vi "Q14070-Z060B.vi"() -> ()   [LabVIEW 2013]
uses:
  <vilib>/Utility/file.llb/Read From Spreadsheet File (string).vi
  <vilib>/express/express arith-compare/Formula/XNode/ExpressFormulaBlockNode.xnode
  PCI8622_32.dll
  <vilib>/printing/EasyPrintingControls.llb/contents.ctl
  <vilib>/Utility/NIReport.llb/NI_ReportGenerationCore.lvlib
  <vilib>/printing/EasyPrintingControls.llb/report_type.ctl
  <vilib>/Utility/NIReport.llb/NI_report.lvclass
  <vilib>/printing/EasyPrinting.llb/Easy Print VI Panel or Documentation (path).vi
panel:
  in  "?":bool
  in  "密码":string
  in  "?":bool
  in  "?":bool
  in  "截取百分比":dbl=0.05
  in  "半行程":dbl=70.0
  in  "是否取消放行按钮":bool
  out "PLC":bool
  out "齿条传动比":dbl=200.0 caption="L+Lmax(mm)" format="%#.3f"
  out "右平均轴向力(N)":dbl caption="L+Lmax(mm)" format="%#.3f"
  out "左平均轴向力(N)":dbl caption="最大位移偏离Lmax(mm)" format="%#.3f"
  in  "确定按钮":bool
  out "员工ID":string
  in  "出支线工步号":dbl
  out "报警提示":string
  in  "报警工步号":dbl
  out "急停":bool
  out "DeviceHandle":u32
  in  "轴向力设定次数":dbl=5.0
  in  "最小间隙(mm)":dbl=0.0005 format="%#.3f"
  out "本备料状态H":bool
  out "本测试状态H":bool
  out "本自动状态H":bool
  out "夹头松开":bool
  out "测头右位":bool
  out "测头左位":bool
  in  "测头气缸右移":bool
  in  "测头气缸左移":bool
  in  "轴向力已做次数":dbl
  out "轴向力及全行程间隙合格":bool
  out "轴向力启动":bool
  out "间隙启动":bool
  out "夹头夹紧位":bool
  in  "夹头松开":bool
  in  "夹头夹紧":bool
  out "找帽扭矩":dbl=5.0 caption="压力传感器" format="%#.2f"
  out "error out":errorcluster
  out "型号数量":i32
  out "error out 4":errorcluster
  in  "间隙设定调整次数":dbl=5.0
  out "读取产品ID":string
  out "本备料状态":bool
  out "本测试状态":bool
  out "本自动状态":bool
  out "FGCS":string
  out "KSJJ":string
  out "Z060BRFID":string
  out "轴向力Y":dbl[](array[numeric])
  out "轴向力X":dbl[](array[numeric])
  out "间隙X数组":dbl[](array[numeric])
  out "间隙Y数组":dbl[](array[numeric])
  out "error out 3":errorcluster caption="错误输出"
  out "rfid工步号":u32
  out "芯片ID":string="201209190001"
  out "rfid完成":bool
  out "rfid触发":bool
  out "本序已做":bool
  in  "回零完成":bool
  in  "电动缸回零":bool
  in  "单点间隙已调试次数":dbl
  in  "需调整角度(度)":dbl
  in  "转向器中心":dbl
  out "扭矩到达":bool
  out "黄灯":bool
  out "红灯":bool
  out "基准位移":dbl caption="压力传感器" format="%#.4f"
  out "上序不合格":bool
  out "单点间隙合格":bool
  out "上序合格":bool
  out "测头机构电机":u32
  out "复位":bool
  in  "型号选择":u16(ring)=1 items=["J709", "J728", "J706"]
  in  "联线按钮":bool
  in  "工步号":u32
  in  "产品ID":string="201209190001"
  out "间隙位移(mm)":dbl caption="压力传感器" format="%#.3f"
  out "齿条推拉力(N)":dbl format="%#.2f"
  out "齿条扭矩(Nm)":dbl format="%#.2f"
  out "通讯状态":bool
  out "员工姓名":string
  out "工步提示":string
  out "ADODB._Connection Out 2":refnum<k7>
  out "旋转齿条电机":u32
  out "电动缸电机":u32
  in  "停止":bool
  in  "参数加载":bool
  in  "选项卡控件":T1(tab)
  in  "180°外全行程间隙标准(mm)":dbl=0.1 format="%#.3f"
  out "扭动曲线":cluster{"Y":dbl[], "Y":dbl[]}[](graph) caption="压球涨堵头1"
  out "中间位置间隙":dbl caption="间隙值L(mm)" format="%#.3f"
  in  "中间位置最大间隙标准(mm)":dbl=0.07 format="%#.3f"
  out "右180°外全行程间隙":dbl caption="正向最大间隙L1(mm)" format="%#.3f"
  out "左180°外全行程间隙":dbl caption="正向最大间隙L1(mm)" format="%#.3f"
  out "右180°内全行程间隙":dbl caption="正向最大间隙L1(mm)" format="%#.3f"
  out "左180°内全行程间隙":dbl caption="正向最大间隙L1(mm)" format="%#.3f"
  in  "180°内全行程间隙标准(mm)":dbl=0.07 format="%#.3f"
  in  "找帽OK":bool
  out "左全行程间隙":dbl caption="正向最大间隙L1(mm)" format="%#.3f"
  out "右全行程间隙":dbl caption="正向最大间隙L1(mm)" format="%#.3f"
  out "总圈数最大值":dbl
  out "总圈数标准":dbl
  out "总行程最大值":dbl
  out "总行程标准(mm)":dbl
  out "力波动标准(N)":dbl=60.0 caption="L+Lmax(mm)" format="%#.3f"
  out "轴向力标准(N)":dbl=100.0 caption="L+Lmax(mm)" format="%#.3f"
  out "右轴向力波动(N)":dbl caption="L+Lmax(mm)" format="%_4g"
  out "右最大轴向力(N)":dbl caption="L+Lmax(mm)" format="%_4g"
  out "左轴向力波动(N)":dbl caption="最大位移偏离Lmax(mm)" format="%_4g"
  out "左最大轴向力(N)":dbl caption="最大位移偏离Lmax(mm)" format="%_4g"
  out "行程跳动曲线":cluster{"Y":dbl[], "Y":dbl[]}[](graph) caption="压球涨堵头1"
  out "平均轴向力标准(N) max":dbl=200.0 caption="L+Lmax(mm)" format="%#.3f"
  out "总行程":dbl format="%_4g"
  out "总圈数":dbl format="%_4g"
  in  "不合格品":bool
  in  "扭矩停止值":dbl=16.0
  in  "齿条右极限":dbl=-70.0 caption="压力传感器" format="%#.2f"
  in  "齿条左极限":dbl=-262.0 caption="压力传感器" format="%#.2f"
  in  "齿条移动速度":dbl=5.0 caption="压力传感器" format="%#.2f"
  in  "旋转齿条轴找帽转速":dbl=5.0 caption="压力传感器" format="%#.2f"
  in  "测量点扭矩":dbl=4.0 caption="压力传感器" format="%#.2f"
  in  "旋转齿条轴测量转速":dbl caption="压力传感器" format="%#.2f"
  in  "测头机构轴后退位":dbl=30.0 caption="压力传感器" format="%#.2f"
  in  "测头机构轴待检位":dbl caption="压力传感器" format="%#.2f"
  in  "测头机构轴检测位":dbl caption="压力传感器" format="%#.2f"
  in  "测头机构轴移动速度":dbl caption="压力传感器" format="%#.2f"
  in  "机械间隙值":dbl=3.5
  in  "阻挡":bool
  in  "放行":bool
  in  "夹头松开":bool
  in  "夹头夹紧":bool
  in  "测头气缸右移":bool
  in  "测头气缸左移":bool
  in  "支线下降":bool
  in  "支线顶升":bool
  in  "出支线":bool
  in  "进支线":bool
  in  "主线下降":bool
  in  "主线顶升":bool
  in  "下阻挡器放行":bool
  in  "上阻挡器放行":bool
  in  "测头机构轴使能":bool
  in  "测头机构轴后退":bool
  in  "测头机构轴前进":bool
  in  "电动缸速度(mm/s)":dbl=10.0 format="%#.3f"
  out "电动缸位置(mm)":dbl=10000.0 format="%#.3f"
  in  "旋转齿条轴速度(°/s)":dbl=10.0 format="%#.3f"
  out "旋转齿条轴位置(°)":dbl=10000.0 format="%#.3f"
  in  "测头机构轴速度(mm/s)":dbl=10.0 format="%#.3f"
  out "测头机构轴位置(mm)":dbl=10000.0 format="%#.3f"
  in  "旋转齿条轴右转":bool
  in  "旋转齿条轴左转":bool
  in  "旋转齿条轴使能":bool
  in  "电动缸后退":bool
  in  "电动缸使能":bool
  in  "电动缸前进":bool
  in  "齿条扭矩比例偏移":dbl=1.0 format="%#.2f"
  in  "齿条扭矩零点偏移":dbl format="%#.2f"
  in  "齿条推拉力比例偏移":dbl=1.0 format="%#.2f"
  in  "齿条推拉力零点偏移":dbl format="%#.2f"
  in  "间隙位移比例偏移":dbl=1.0 format="%#.2f"
  in  "间隙位移零点偏移":dbl format="%#.2f"
  in  "传感器参数保存":bool
  in  "参数修改":bool
  in  "参数查询":bool
  in  "参数浏览表":string[][](table)
  # "芜湖机械转向器装配线"
  # "间隙及轴向力检测"
  # "Q14070机械转向器装配线"
  # "湖北唯思凌科装备制造有限公司 设计开发 (C)2015"
  # "间隙测量结果"
  # "间隙测量判定值"
  # "≤"
  # "≤"
  # "≤"
  # "轴向力测量结果"
  # "轴向力测量标准"
  # "≥"
  # "≤"
  # "≥"
  # "≤"
  # "≤"
  # "≥"
  # "不得大于20NM"
  # "传感器校验区"
  # "关于传感器校验：\n1、传感器校验需要由具备资质的单位或部门进行校验。\n2、具备权限的用户才能够修改传感器校验参数和试验参数。\n3、修改校验参数方法：先将比例偏移置为1，修改零点偏移，使零点值与校验的传感器一致；然后根据增幅调整比例偏移。"
  # "注意：\n具备权限的用户才能够修改传感器校验参数和试验参数！"
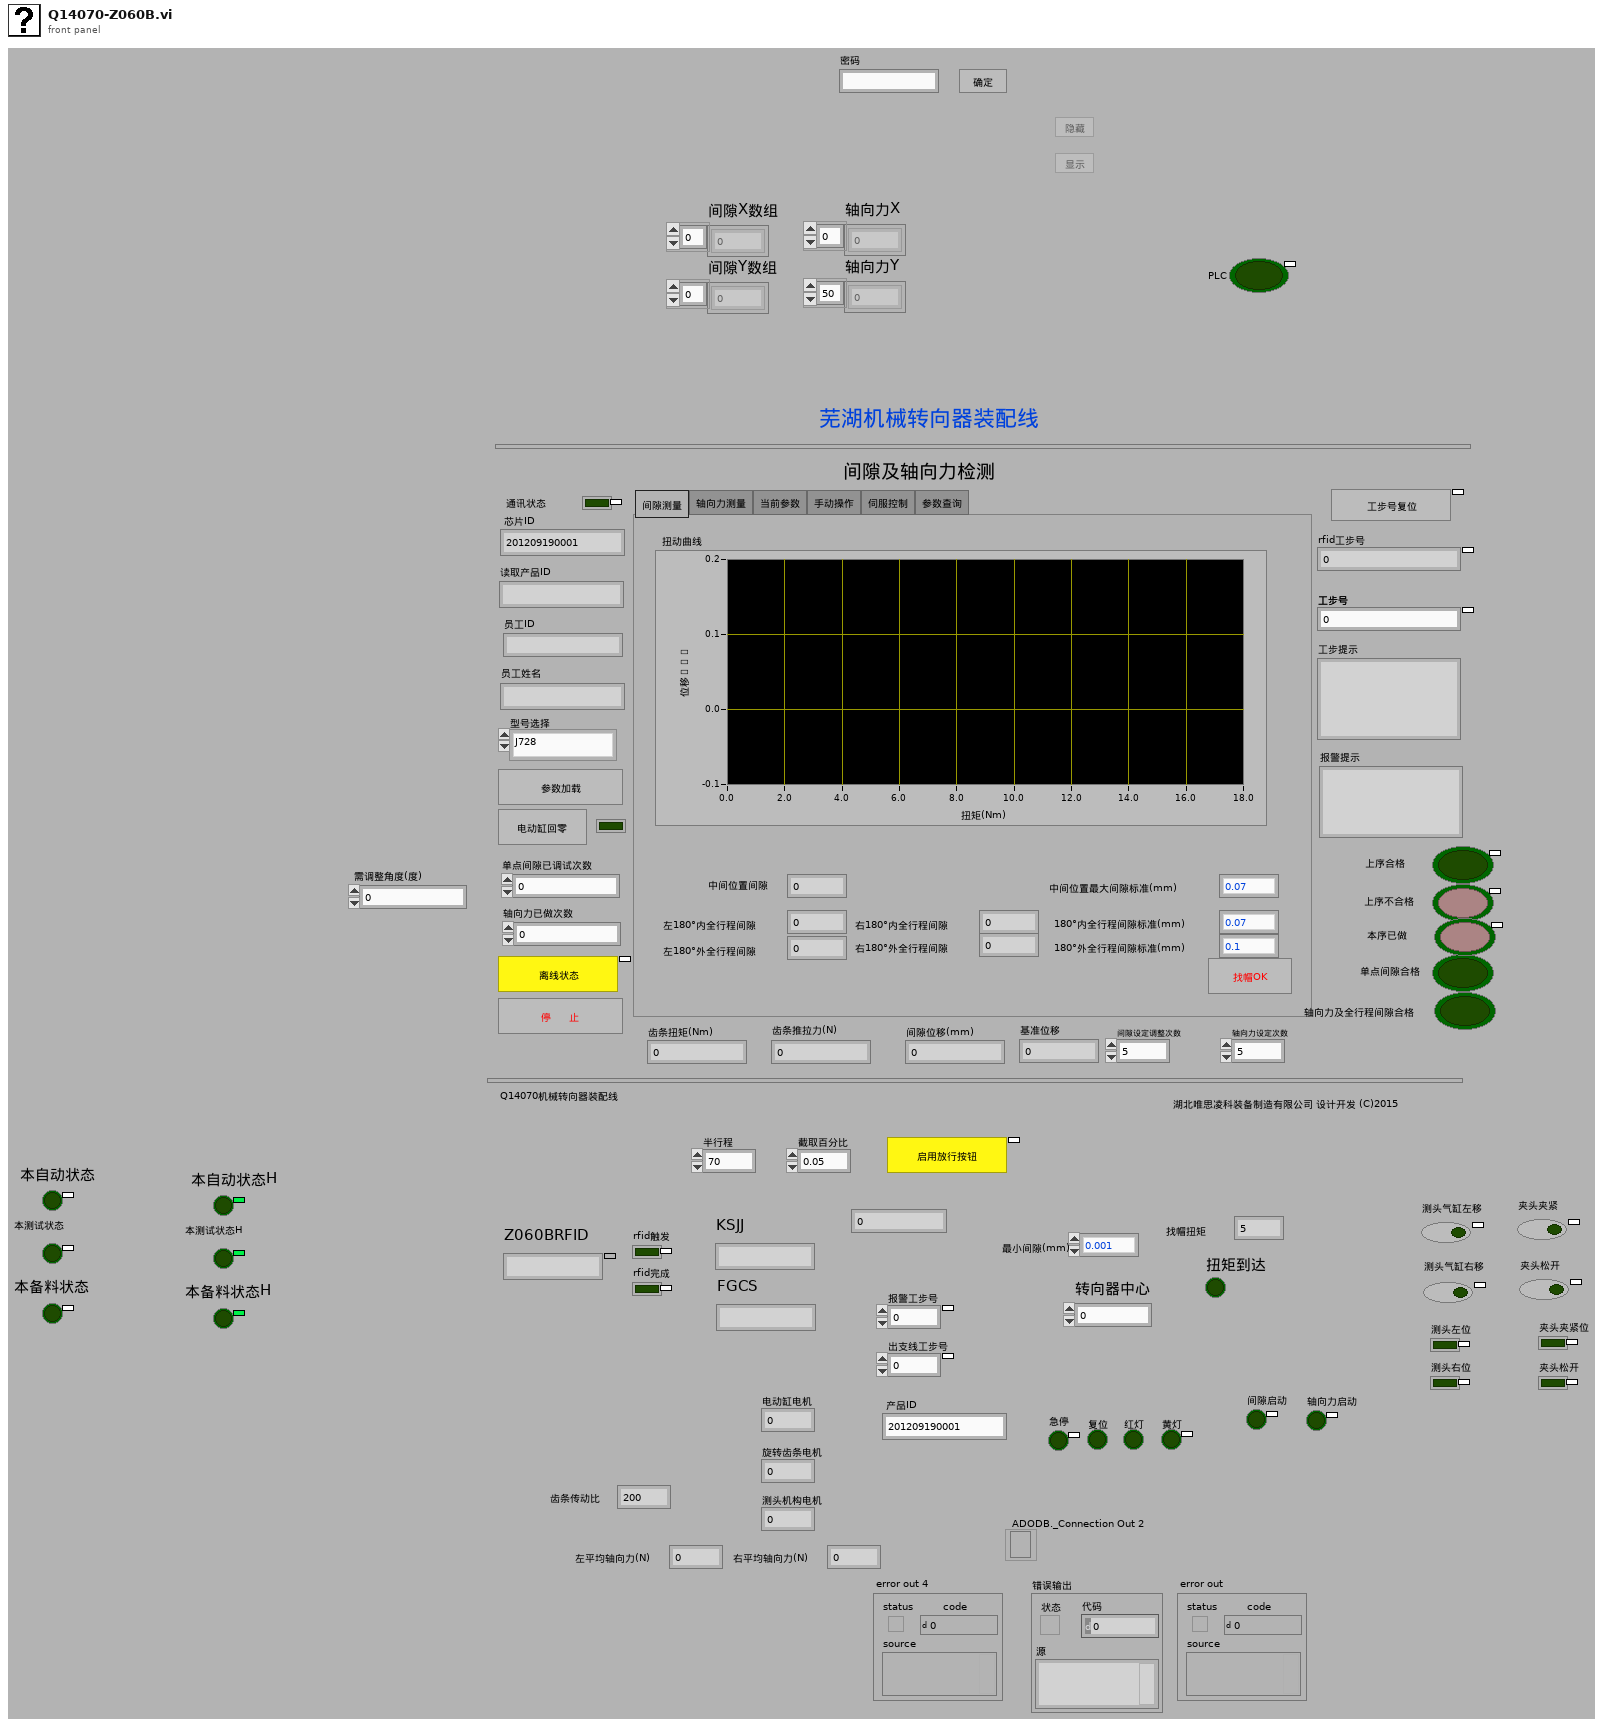
[diagram p1: front panel]
types:
  T1 = enum32{"间隙测量", "轴向力测量", "当前参数", "手动操作", "伺服控制", "传感器校验", "参数查询"}
  T2 = typedef "NI_ReportGenerationCore.lvlib/report_type.ctl" = u16
  T3 = typedef "NI_ReportGenerationCore.lvlib/contents.ctl" = u16
  T4 = typedef "imagedata.ctl" = cluster{"image type":i32, "image depth":i32, "image":u8[], "mask":u8[], "colors":u32[], "Rectangle":cluster{"left":i16, "top":i16, "right":i16, "bottom":i16}}
  T5 = enum8{"Enabled", "Disabled", "Disabled and Grayed Out"}
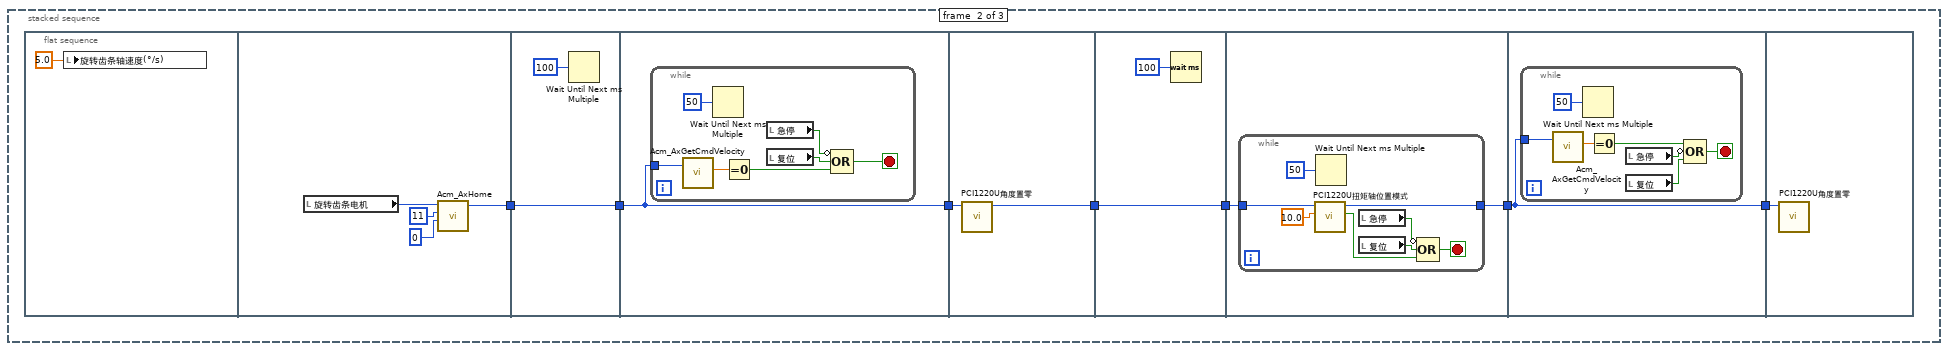
[diagram p2: hidden frame]
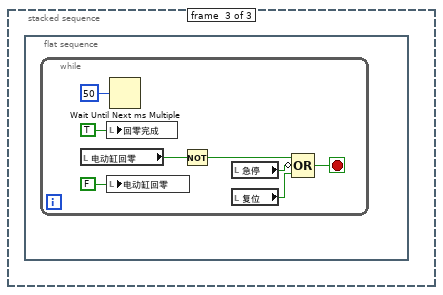
[diagram p3: hidden frame]
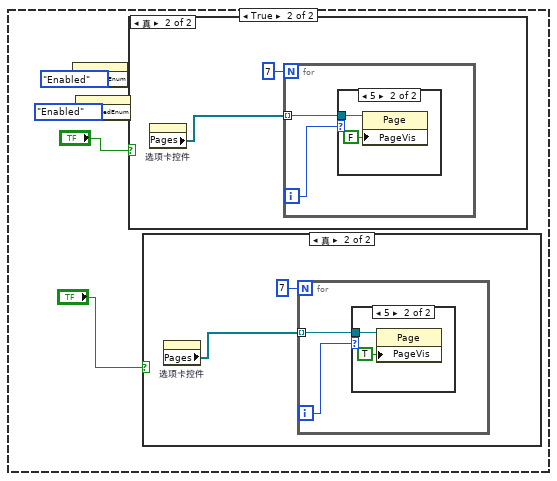
[diagram p5: hidden frame]
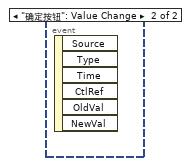
[diagram p10: hidden frame]
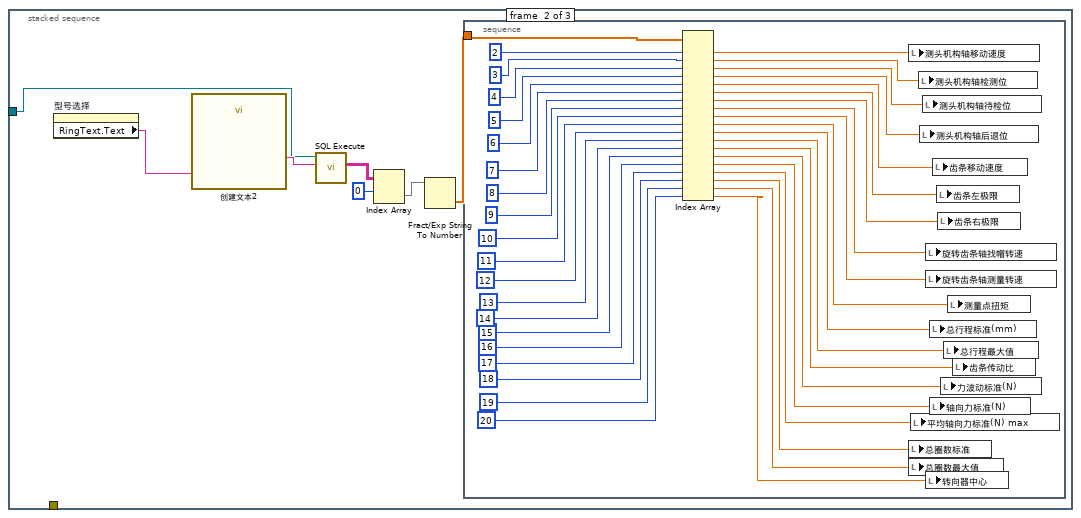
[diagram p13: hidden frame]
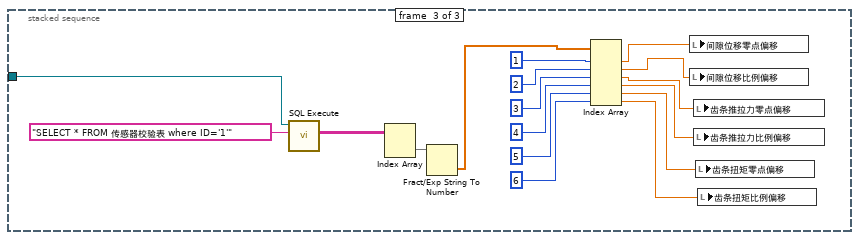
[diagram p14: hidden frame]
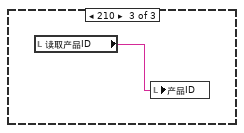
[diagram p16: hidden frame]
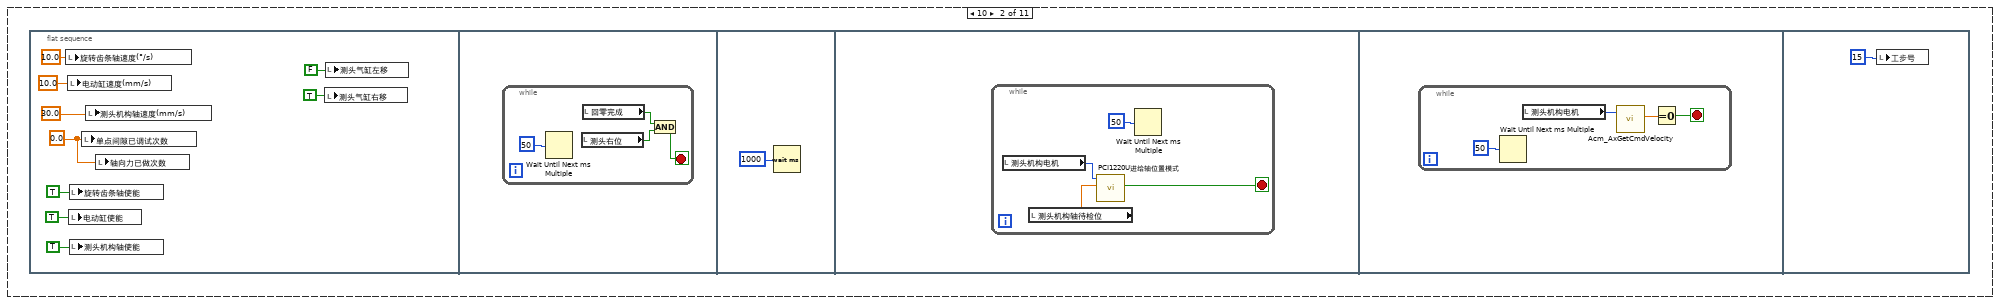
[diagram p18: hidden frame]
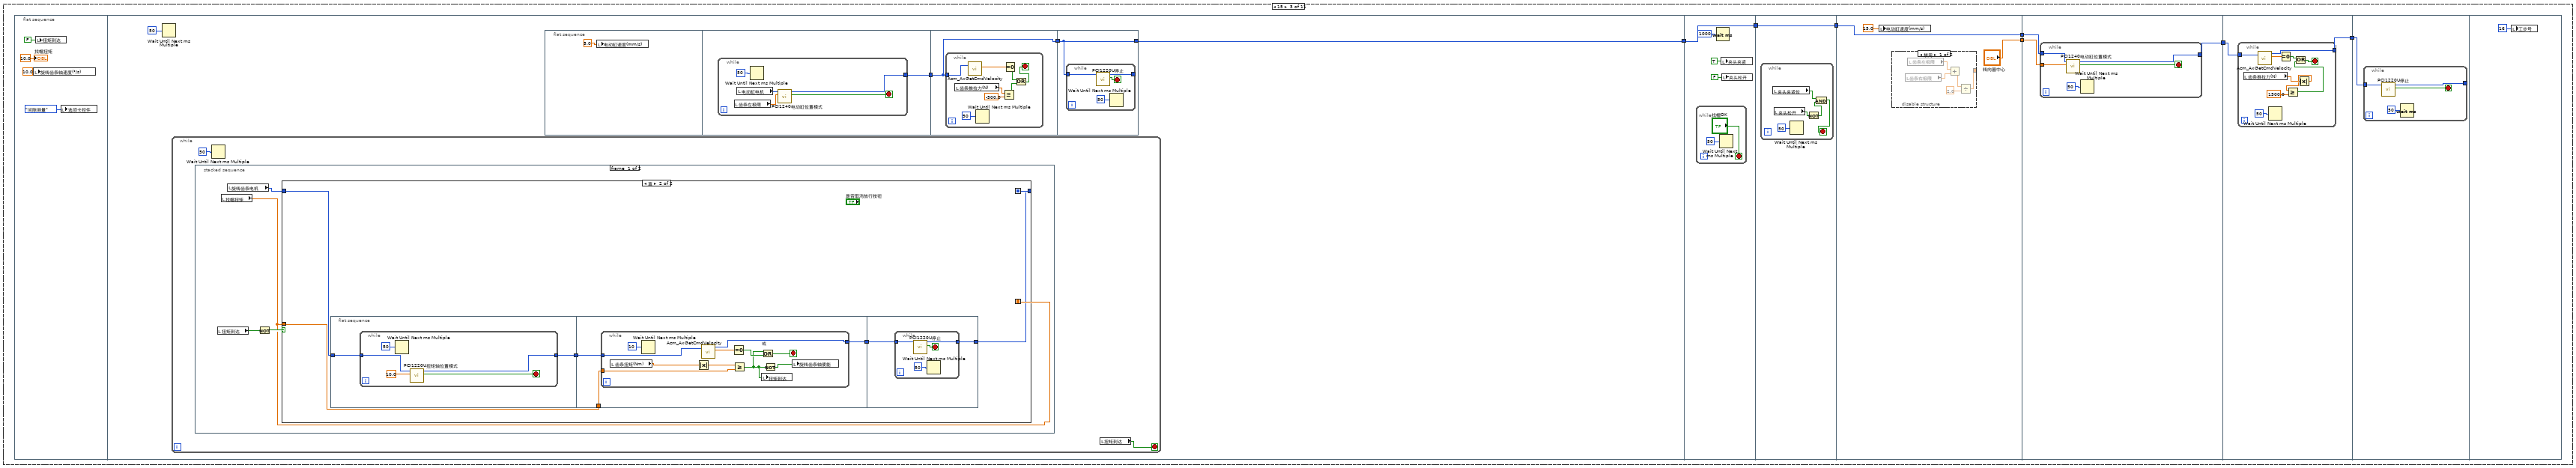
[diagram p19: hidden frame]
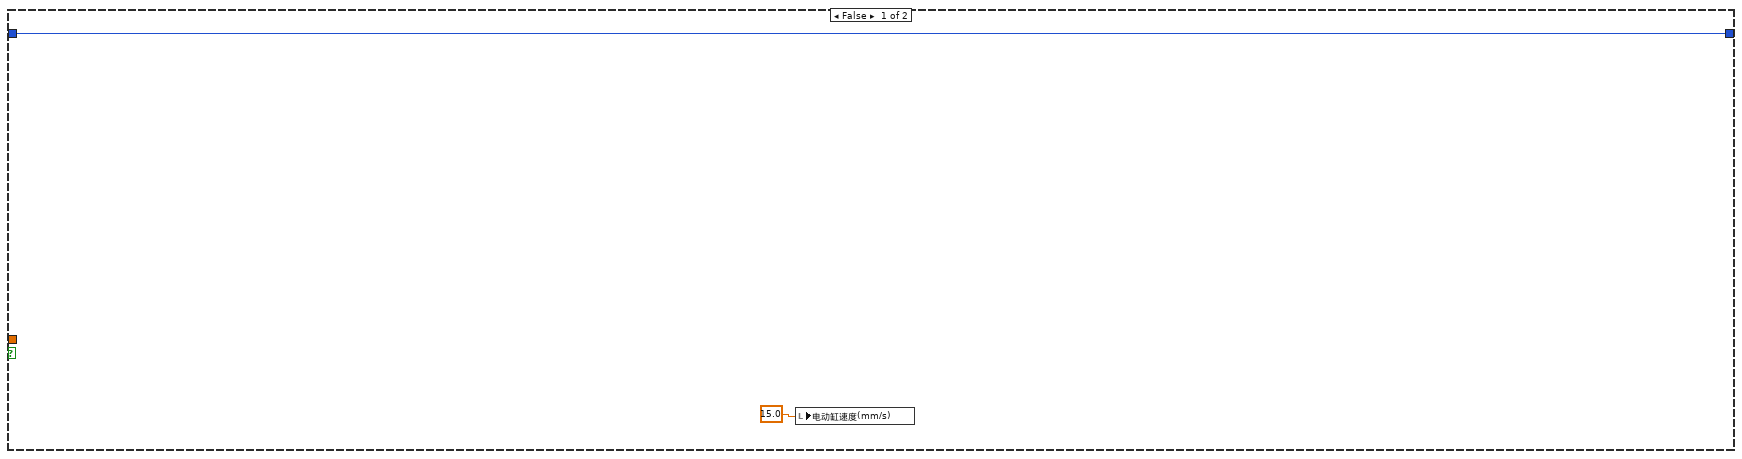
[diagram p20: hidden frame]
diagram:
  n1 = while {
    stop <- w7 stop-if-true
    n2 = local read "工步号"() -> (w5:u32)
    n3 = case shown="40" w5 {
      frame 0, Default {
      }
      frame 10 {
        n4 = flat-sequence {
          frame #0 {
            w8 = 0.0 ("已调试次数")
            n5 = local write "旋转齿条轴速度(°/s)"(10.0 ("旋转齿条轴速度(°/s)")) -> ()
            n6 = local write "电动缸速度(mm/s)"(10.0 ("电动缸速度(mm/s)")) -> ()
            n7 = local write "电动缸使能"(TRUE ("电动缸使能")) -> ()
            n8 = local write "旋转齿条轴使能"(TRUE ("旋转齿条轴使能")) -> ()
            n9 = local write "测头机构轴使能"(TRUE ("调整机构轴使能")) -> ()
            n10 = local write "单点间隙已调试次数"(w8) -> ()
            n11 = local write "测头机构轴速度(mm/s)"(30.0 ("调整机构轴速度(mm/s)")) -> ()
            n12 = local write "轴向力已做次数"(w8) -> ()
            n13 = local write "测头气缸右移"(TRUE ("测头气缸右移")) -> ()
            n14 = local write "测头气缸左移"(FALSE ("测头气缸左移")) -> ()
          }
          frame #1 {
            n15 = while {
              stop <- w17 stop-if-true
              n16 = Wait Until Next ms Multiple(millisecond multiple=u32 50 ("毫秒倍数")) -> ()  [unwired: 1 out]
              n17 = local read "测头右位"() -> (w18:bool)
              n18 = local read "回零完成"() -> (w19:bool)
              n19 = And(x=w19, y=w18) -> (x .and. y?=w17:bool)
            }
          }
          frame #2 {
            n20 = Wait (ms)(milliseconds to wait=u32 1000 ("等待时间（毫秒）")) -> ()  [unwired: 1 out]
          }
          frame #3 {
            n21 = while {
              stop <- w25 stop-if-true
              n22 = local read "测头机构电机"() -> (w23:u32)
              n23 = local read "测头机构轴待检位"() -> (w22:dbl)
              n24 = call "PCI1220U进给轴位置模式.vi"("Distance"=w22, "AxisHandle IN"=w23) -> ("AbsSuccess"=w25:bool)  [unwired: 8 in, 1 out]
              n25 = Wait Until Next ms Multiple(millisecond multiple=u32 50 ("毫秒倍数")) -> ()  [unwired: 1 out]
            }
          }
          frame #4 {
            n26 = while {
              stop <- w28 stop-if-true
              n27 = Wait Until Next ms Multiple(millisecond multiple=u32 50 ("毫秒倍数")) -> ()  [unwired: 1 out]
              n28 = local read "测头机构电机"() -> (w26:u32)
              n29 = call <userlib>:"Acm_AxGetCmdVelocity.vi"("AxisHandle"=w26) -> ("Velocity"=w29:dbl)  [unwired: 1 in, 3 out]
              n30 = Equal To 0?(x=w29) -> (x = 0?=w28:bool)
            }
          }
          frame #5 {
            n31 = local write "工步号"(u32 15 ("工步号")) -> ()
          }
        }
      }
      frame 15 {
        n32 = flat-sequence {
          tunnel: [w43] -> w34
          tunnel: w34 -> [w145]
          tunnel: [w145] -> w32
          tunnel: w32 -> [w149]
          tunnel: [w149] -> w31
          tunnel: [w156] -> w37
          tunnel: ["转向器中心"] -> w36
          tunnel: w31 -> [w156]
          tunnel: w37 -> [w165]
          tunnel: w36 -> [w164]
          tunnel: [w163] -> w35
          tunnel: w35 -> [w172]
          tunnel: [w171] -> w33
          tunnel: w33 -> [w183]
          frame #0 {
            n33 = local write "旋转齿条轴速度(°/s)"(10.0 ("旋转齿条轴速度(°/s)")) -> ()
            n34 = local write "扭矩到达"(FALSE ("扭矩到达")) -> ()
            n35 = local write "选项卡控件"(T1."间隙测量" ("选项卡控件")) -> ()
            "找帽扭矩" <- 10.0 ("找帽扭矩")
          }
          frame #1 {
            n36 = Wait Until Next ms Multiple(millisecond multiple=u32 50 ("毫秒倍数")) -> ()  [unwired: 1 out]
            n37 = while {
              stop <- w46 stop-if-true
              n38 = stacked-sequence {
                seq-local: [w48 _] -> [_ w89]
                seq-local: [w52 _] -> [_ w88]
                frame #0 {
                  n39 = local read "扭矩到达"() -> (w50:bool)
                  n40 = local read "找帽扭矩"() -> (w48:dbl)
                  n41 = local read "旋转齿条电机"() -> (w49:u32)
                  n42 = Not(x=w50) -> (.not. x?=w51:bool)
                  n43 = case shown="真" w51 {
                    tunnel: [w54 w55] -> w52
                    tunnel: w49 -> [w54 w59]
                    tunnel: w48 -> [_ w57]
                    frame False {
                      n44 = local write "电动缸速度(mm/s)"(15.0 ("电动缸速度(mm/s)")) -> ()
                    }
                    frame True {
                      n45 = flat-sequence {
                        tunnel: w59 -> [w61]
                        tunnel: [w60] -> w58
                        tunnel: w58 -> [w69]
                        tunnel: w57 -> [w68]
                        tunnel: [w67] -> w56
                        tunnel: w56 -> [w82]
                        tunnel: [w81] -> w55
                        frame #0 {
                          n46 = while {
                            tunnel: [w65] -> w60
                            tunnel: w61 -> [w62]
                            stop <- w64 stop-if-true
                            n47 = Wait Until Next ms Multiple(millisecond multiple=u32 50 ("毫秒倍数")) -> ()  [unwired: 1 out]
                            n48 = call "PCI1220U扭矩轴位置模式.vi"("Distance"=10.0, "AxisHandle IN"=w62) -> ("AbsSuccess"=w64:bool, "AxisHandle OUT"=w65:u32)  [unwired: 8 in]
                          }
                        }
                        frame #1 {
                          n49 = while {
                            tunnel: w69 -> [w79]
                            tunnel: w68 -> [w74]
                            tunnel: [w73] -> w67
                            stop <- w75 stop-if-true
                            n50 = local read "齿条扭矩(Nm)"() -> (w72:dbl)
                            n51 = Wait Until Next ms Multiple(millisecond multiple=u32 10 ("毫秒倍数")) -> ()  [unwired: 1 out]
                            n52 = Absolute Value(x=w72) -> (abs(x)=w77:dbl)
                            n53 = call <userlib>:"Acm_AxGetCmdVelocity.vi"("AxisHandle"=w79) -> ("Velocity"=w78:dbl, "AxisHandle"=w73:u32)  [unwired: 1 in, 2 out]
                            n54 = Equal To 0?(x=w78) -> (x = 0?=w76:bool)
                            n55 = Greater Or Equal?(x=w77, y=w74) -> (x >= y?=w71:bool)
                            n56 = Or "或"(x=w71, y=w76) -> (x .or. y?=w75:bool)
                            n57 = local write "扭矩到达"(w71) -> ()
                            n58 = Not(x=w71) -> (.not. x?=w70:bool)
                            n59 = local write "旋转齿条轴使能"(w70) -> ()
                          }
                        }
                        frame #2 {
                          n60 = while {
                            tunnel: w82 -> [w86]
                            tunnel: [w83] -> w81
                            stop <- w85 stop-if-true
                            n61 = call "PCI1220U停止.vi"("AxisHandle IN"=w86) -> ("完成"=w85:bool, "AxisHandle OUT"=w83:u32)  [unwired: 9 in]
                            n62 = Wait Until Next ms Multiple(millisecond multiple=u32 50 ("毫秒倍数")) -> ()  [unwired: 1 out]
                          }
                        }
                      }
                    }
                  }
                }
                frame #1 {
                  n63 = local read "扭矩到达"() -> (w87:bool)
                  n64 = Not(x=w87) -> (.not. x?=w90:bool)
                  n65 = case shown="假" w90 {
                    tunnel: w88 -> [_ w95]
                    tunnel: w89 -> [_ w93]
                    frame False {
                      n66 = local write "电动缸速度(mm/s)"(15.0 ("电动缸速度(mm/s)")) -> ()
                    }
                    frame True {
                      n67 = flat-sequence {
                        tunnel: w95 -> [w96]
                        tunnel: [w97] -> w94
                        tunnel: w94 -> [w105]
                        tunnel: w93 -> [w104]
                        tunnel: [w103] -> w92
                        tunnel: w92 -> [w117]
                        frame #0 {
                          n68 = while {
                            tunnel: [w101] -> w97
                            tunnel: w96 -> [w98]
                            stop <- w100 stop-if-true
                            n69 = Wait Until Next ms Multiple(millisecond multiple=u32 50 ("毫秒倍数")) -> ()  [unwired: 1 out]
                            n70 = call "PCI1220U扭矩轴位置模式.vi"("Distance"=-29.0, "AxisHandle IN"=w98) -> ("AbsSuccess"=w100:bool, "AxisHandle OUT"=w101:u32)  [unwired: 8 in]
                          }
                        }
                        frame #1 {
                          n71 = while {
                            tunnel: w105 -> [w115]
                            tunnel: [w110] -> w103
                            tunnel: w104 -> [w109]
                            stop <- w111 stop-if-true
                            n72 = local read "齿条扭矩(Nm)"() -> (w108:dbl)
                            n73 = Wait Until Next ms Multiple(millisecond multiple=u32 50 ("毫秒倍数")) -> ()  [unwired: 1 out]
                            n74 = Absolute Value(x=w108) -> (abs(x)=w113:dbl)
                            n75 = call <userlib>:"Acm_AxGetCmdVelocity.vi"("AxisHandle"=w115) -> ("Velocity"=w114:dbl, "AxisHandle"=w110:u32)  [unwired: 1 in, 2 out]
                            n76 = Equal To 0?(x=w114) -> (x = 0?=w112:bool)
                            n77 = Greater Or Equal?(x=w113, y=w109) -> (x >= y?=w106:bool)
                            n78 = Or(x=w106, y=w112) -> (x .or. y?=w111:bool)
                            n79 = Not(x=w106) -> (.not. x?=w107:bool)
                            n80 = local write "扭矩到达"(w106) -> ()
                            n81 = local write "旋转齿条轴使能"(w107) -> ()
                          }
                        }
                        frame #2 {
                          n82 = while {
                            tunnel: w117 -> [w121]
                            tunnel: [w118] -> _
                            stop <- w120 stop-if-true
                            n83 = call "PCI1220U停止.vi"("AxisHandle IN"=w121) -> ("完成"=w120:bool, "AxisHandle OUT"=w118:u32)  [unwired: 9 in]
                            n84 = Wait Until Next ms Multiple(millisecond multiple=u32 50 ("毫秒倍数")) -> ()  [unwired: 1 out]
                          }
                        }
                      }
                    }
                  }
                }
              }
              n85 = Wait Until Next ms Multiple(millisecond multiple=u32 50 ("毫秒倍数")) -> ()  [unwired: 1 out]
              n86 = local read "扭矩到达"() -> (w46:bool)
            }
            n87 = flat-sequence {
              tunnel: [w123] -> w45
              tunnel: w45 -> [w129]
              tunnel: [w129] -> w42
              tunnel: [w138] -> w43
              tunnel: w42 -> [w138]
              frame #0 {
                n88 = local write "电动缸速度(mm/s)"(5.0 ("电动缸速度(mm/s)")) -> ()
              }
              frame #1 {
                n89 = while {
                  tunnel: [w127] -> w123
                  stop <- w126 stop-if-true
                  n90 = local read "齿条左极限"() -> (w124:dbl)
                  n91 = local read "电动缸电机"() -> (w128:u32)
                  n92 = Wait Until Next ms Multiple(millisecond multiple=u32 50 ("毫秒倍数")) -> ()  [unwired: 1 out]
                  n93 = call "PCI1240电动缸位置模式 .vi"("Distance"=w124, "AxisHandle IN"=w128) -> ("AbsSuccess"=w126:bool, "AxisHandle OUT"=w127:u32)  [unwired: 8 in]
                }
              }
              frame #2 {
                n94 = while {
                  tunnel: w129 -> [w136]
                  stop <- w133 stop-if-true
                  n95 = local read "齿条推拉力(N)"() -> (w132:dbl)
                  n96 = call <userlib>:"Acm_AxGetCmdVelocity.vi"("AxisHandle"=w136) -> ("Velocity"=w137:dbl)  [unwired: 1 in, 3 out]
                  n97 = Wait Until Next ms Multiple(millisecond multiple=u32 50 ("毫秒倍数")) -> ()  [unwired: 1 out]
                  n98 = Less Or Equal?(x=w132, y=-500.0) -> (x <= y?=w130:bool)
                  n99 = Equal To 0?(x=w137) -> (x = 0?=w134:bool)
                  n100 = Or(x=w134, y=w130) -> (x .or. y?=w133:bool)
                }
              }
              frame #3 {
                n101 = while {
                  tunnel: w138 -> [w142]
                  tunnel: [w139] -> _
                  stop <- w141 stop-if-true
                  n102 = call "PCI1220U停止.vi"("AxisHandle IN"=w142) -> ("完成"=w141:bool, "AxisHandle OUT"=w139:u32)  [unwired: 9 in]
                  n103 = Wait Until Next ms Multiple(millisecond multiple=u32 50 ("毫秒倍数")) -> ()  [unwired: 1 out]
                }
              }
            }
          }
          frame #2 {
            n104 = while {
              stop <- "找帽OK" stop-if-true
              n105 = Wait Until Next ms Multiple(millisecond multiple=u32 50 ("毫秒倍数")) -> ()  [unwired: 1 out]
            }
            n106 = Wait (ms)(milliseconds to wait=u32 1000 ("毫秒倍数")) -> ()  [unwired: 1 out]
            n107 = local write "夹头夹紧"(TRUE ("夹头夹紧")) -> ()
            n108 = local write "夹头松开"(FALSE ("夹头松开")) -> ()
          }
          frame #3 {
            n109 = while {
              stop <- w151 stop-if-true
              n110 = local read "夹头夹紧位"() -> (w152:bool)
              n111 = local read "夹头松开"() -> (w154:bool)
              n112 = Wait Until Next ms Multiple(millisecond multiple=u32 50 ("毫秒倍数")) -> ()  [unwired: 1 out]
              n113 = Not(x=w154) -> (.not. x?=w153:bool)
              n114 = And(x=w152, y=w153) -> (x .and. y?=w151:bool)
            }
          }
          frame #4 {
            n115 = local write "电动缸速度(mm/s)"(15.0 ("电动缸轴移动速度")) -> ()
            n116 = disable-structure shown="禁用" {
              disable-tunnel: [w158 _] -> _
              frame Disabled {
                n117 = local read "齿条右极限"() -> (w161:dbl)
                n118 = local read "齿条左极限"() -> (w162:dbl)
                n119 = Add(x=w162, y=w161) -> (x+y=w160:dbl)
                n120 = Divide(x=w160, y=2.0) -> (x/y=w158:dbl)
              }
              frame Enabled {
              }
            }
          }
          frame #5 {
            n121 = while {
              tunnel: w165 -> [w170]
              tunnel: w164 -> [w169]
              tunnel: [w166] -> w163
              stop <- w168 stop-if-true
              n122 = call "PCI1240电动缸位置模式 .vi"("Distance"=w169, "AxisHandle IN"=w170) -> ("AbsSuccess"=w168:bool, "AxisHandle OUT"=w166:u32)  [unwired: 8 in]
              n123 = Wait Until Next ms Multiple(millisecond multiple=u32 50 ("毫秒倍数")) -> ()  [unwired: 1 out]
            }
          }
          frame #6 {
            n124 = while {
              tunnel: w172 -> [w182]
              tunnel: [w173] -> w171
              stop <- w174 stop-if-true
              n125 = local read "齿条推拉力(N)"() -> (w179:dbl)
              n126 = call <userlib>:"Acm_AxGetCmdVelocity.vi"("AxisHandle"=w182) -> ("Velocity"=w181:dbl, "AxisHandle"=w173:u32)  [unwired: 1 in, 2 out]
              n127 = Wait Until Next ms Multiple(millisecond multiple=u32 50 ("毫秒倍数")) -> ()  [unwired: 1 out]
              n128 = Equal To 0?(x=w181) -> (x = 0?=w176:bool)
              n129 = Absolute Value(x=w179) -> (abs(x)=w178:dbl)
              n130 = Greater Or Equal?(x=w178, y=1500.0) -> (x >= y?=w175:bool)
              n131 = Or(x=w176, y=w175) -> (x .or. y?=w174:bool)
            }
          }
          frame #7 {
            n132 = while {
              tunnel: w183 -> [w187]
              tunnel: [w186] -> _
              stop <- w185 stop-if-true
              n133 = call "PCI1220U停止.vi"("AxisHandle IN"=w187) -> ("完成"=w185:bool, "AxisHandle OUT"=w186:u32)  [unwired: 9 in]
              n134 = Wait (ms)(milliseconds to wait=u32 50 ("毫秒倍数")) -> ()  [unwired: 1 out]
            }
          }
          frame #8 {
            n135 = local write "工步号"(u32 16 ("工步号")) -> ()
          }
        }
      }
      frame 16 {
        n136 = flat-sequence {
          tunnel: [w201] -> w198
          tunnel: [w200] -> w197
          tunnel: w198 -> [w204]
          tunnel: w197 -> [w203]
          tunnel: [w202] -> w196
          tunnel: w196 -> [w211]
          tunnel: [w211] -> w195
          tunnel: w195 -> [w213]
          tunnel: [w212] -> w194
          tunnel: w194 -> [w225]
          tunnel: [w224] -> w192
          tunnel: [w231] -> w193
          tunnel: w192 -> [w231]
          tunnel: w193 -> [w234]
          tunnel: [w233] -> w191
          tunnel: w191 -> [w246]
          tunnel: [w245] -> w189
          tunnel: [w252] -> w190
          tunnel: w189 -> [w252]
          tunnel: w190 -> [w254]
          frame #0 {
            n137 = local read "电动缸电机"() -> (w201:u32)
            n138 = local read "齿条左极限"() -> (w200:dbl)
            n139 = local write "电动缸速度(mm/s)"(30.0 ("齿条移动速度")) -> ()
          }
          frame #1 {
            n140 = while {
              tunnel: w204 -> [w209]
              tunnel: w203 -> [w208]
              tunnel: [w205] -> w202
              stop <- w207 stop-if-true
              n141 = call "PCI1240电动缸位置模式 .vi"("Distance"=w208, "AxisHandle IN"=w209) -> ("AbsSuccess"=w207:bool, "AxisHandle OUT"=w205:u32)  [unwired: 8 in]
              n142 = Wait Until Next ms Multiple(millisecond multiple=u32 50 ("毫秒倍数")) -> ()  [unwired: 1 out]
            }
          }
          frame #2 {
            n143 = Wait Until Next ms Multiple(millisecond multiple=u32 200 ("毫秒倍数")) -> ()  [unwired: 1 out]
          }
          frame #3 {
            n144 = while {
              tunnel: w213 -> [w223]
              tunnel: [w214] -> w212
              stop <- w215 stop-if-true
              n145 = local read "齿条推拉力(N)"() -> (w220:dbl)
              n146 = call <userlib>:"Acm_AxGetCmdVelocity.vi"("AxisHandle"=w223) -> ("Velocity"=w222:dbl, "AxisHandle"=w214:u32)  [unwired: 1 in, 2 out]
              n147 = Wait Until Next ms Multiple(millisecond multiple=u32 50 ("毫秒倍数")) -> ()  [unwired: 1 out]
              n148 = Equal To 0?(x=w222) -> (x = 0?=w217:bool)
              n149 = Absolute Value(x=w220) -> (abs(x)=w219:dbl)
              n150 = Greater Or Equal?(x=w219, y=1500.0) -> (x >= y?=w216:bool)
              n151 = Or(x=w217, y=w216) -> (x .or. y?=w215:bool)
            }
          }
          frame #4 {
            n152 = while {
              tunnel: w225 -> [w230]
              tunnel: [w227] -> w224
              stop <- w229 stop-if-true
              n153 = local read "齿条右极限"() -> (w226:dbl)
              n154 = call "PCI1240电动缸位置模式 .vi"("Distance"=w226, "AxisHandle IN"=w230) -> ("AbsSuccess"=w229:bool, "AxisHandle OUT"=w227:u32)  [unwired: 8 in]
              n155 = Wait Until Next ms Multiple(millisecond multiple=u32 50 ("毫秒倍数")) -> ()  [unwired: 1 out]
            }
          }
          frame #5 {
            n156 = Wait Until Next ms Multiple(millisecond multiple=u32 200 ("毫秒倍数")) -> ()  [unwired: 1 out]
          }
          frame #6 {
            n157 = while {
              tunnel: w234 -> [w244]
              tunnel: [w235] -> w233
              stop <- w236 stop-if-true
              n158 = local read "齿条推拉力(N)"() -> (w241:dbl)
              n159 = call <userlib>:"Acm_AxGetCmdVelocity.vi"("AxisHandle"=w244) -> ("Velocity"=w243:dbl, "AxisHandle"=w235:u32)  [unwired: 1 in, 2 out]
              n160 = Wait Until Next ms Multiple(millisecond multiple=u32 50 ("毫秒倍数")) -> ()  [unwired: 1 out]
              n161 = Equal To 0?(x=w243) -> (x = 0?=w238:bool)
              n162 = Absolute Value(x=w241) -> (abs(x)=w240:dbl)
              n163 = Greater Or Equal?(x=w240, y=1000.0) -> (x >= y?=w237:bool)
              n164 = Or(x=w238, y=w237) -> (x .or. y?=w236:bool)
            }
          }
          frame #7 {
            n165 = while {
              tunnel: w246 -> [w251]
              tunnel: [w248] -> w245
              stop <- w250 stop-if-true
              n166 = local read "转向器中心"() -> (w247:dbl)
              n167 = call "PCI1240电动缸位置模式 .vi"("Distance"=w247, "AxisHandle IN"=w251) -> ("AbsSuccess"=w250:bool, "AxisHandle OUT"=w248:u32)  [unwired: 8 in]
              n168 = Wait Until Next ms Multiple(millisecond multiple=u32 50 ("毫秒倍数")) -> ()  [unwired: 1 out]
            }
          }
          frame #8 {
            n169 = Wait Until Next ms Multiple(millisecond multiple=u32 200 ("毫秒倍数")) -> ()  [unwired: 1 out]
          }
          frame #9 {
            n170 = while {
              tunnel: w254 -> [w264]
              tunnel: [w255] -> _
              stop <- w256 stop-if-true
              n171 = local read "齿条推拉力(N)"() -> (w261:dbl)
              n172 = call <userlib>:"Acm_AxGetCmdVelocity.vi"("AxisHandle"=w264) -> ("Velocity"=w263:dbl, "AxisHandle"=w255:u32)  [unwired: 1 in, 2 out]
              n173 = Wait Until Next ms Multiple(millisecond multiple=u32 50 ("毫秒倍数")) -> ()  [unwired: 1 out]
              n174 = Equal To 0?(x=w263) -> (x = 0?=w258:bool)
              n175 = Absolute Value(x=w261) -> (abs(x)=w260:dbl)
              n176 = Greater Or Equal?(x=w260, y=1500.0) -> (x >= y?=w257:bool)
              n177 = Or(x=w258, y=w257) -> (x .or. y?=w256:bool)
            }
          }
          frame #10 {
            n178 = local write "工步号"(u32 20 ("工步号")) -> ()
          }
        }
      }
      frame 20 {
        n179 = flat-sequence {
          tunnel: [w294] -> w275
          tunnel: w275 -> [w300]
          tunnel: [w307] -> w271
          tunnel: w271 -> [w314]
          tunnel: [w314] -> w270
          tunnel: w270 -> [w322]
          tunnel: [w322] -> w269
          tunnel: w269 -> [w323]
          tunnel: [w329] -> w273
          tunnel: [w331] -> w274
          tunnel: w273 -> [w331]
          tunnel: [w333] -> w280
          tunnel: w274 -> [w333]
          tunnel: w280 -> [w340]
          tunnel: [w339] -> w279
          tunnel: [w344] -> w278
          tunnel: [w343] -> w277
          tunnel: w279 -> [w342]
          tunnel: [w342] -> w276
          tunnel: [w371] -> w283
          tunnel: [w368] -> w282
          tunnel: w278 -> [w368]
          tunnel: [w367] -> w281
          tunnel: w277 -> [w367]
          tunnel: w276 -> [w371]
          tunnel: w283 -> [w375]
          tunnel: [w374] -> w272
          tunnel: w282 -> [w372]
          tunnel: w281 -> [w373]
          tunnel: w272 -> [w381]
          tunnel: [w380] -> w267
          tunnel: w267 -> [w388]
          tunnel: [w388] -> w266
          tunnel: w266 -> [w390]
          tunnel: [w389] -> w268
          tunnel: w268 -> [w400]
          frame #0 {
            n180 = local write "选项卡控件"(T1."间隙测量" ("选项卡控件")) -> ()
          }
          frame #1 {
            n181 = while {
              stop <- w285 stop-if-true
              n182 = local read "夹头松开"() -> (w287:bool)
              n183 = local read "夹头夹紧位"() -> (w286:bool)
              n184 = Wait Until Next ms Multiple(millisecond multiple=u32 50 ("毫秒倍数")) -> ()  [unwired: 1 out]
              n185 = Not(x=w287) -> (.not. x?=w288:bool)
              n186 = And(x=w286, y=w288) -> (x .and. y?=w285:bool)
            }
          }
          frame #2 {
            n187 = local read "转向器中心"() -> (w290:dbl)
            n188 = local read "电动缸电机"() -> (w293:u32)
            n189 = Add(x=w290, y=0.0) -> (x+y=w292:dbl)
            n190 = while {
              tunnel: w293 -> [w299]
              tunnel: w292 -> [w298]
              tunnel: [w295] -> w294
              stop <- w297 stop-if-true
              n191 = call "PCI1240电动缸位置模式 .vi"("Distance"=w298, "AxisHandle IN"=w299) -> ("AbsSuccess"=w297:bool, "AxisHandle OUT"=w295:u32)  [unwired: 8 in]
              n192 = Wait Until Next ms Multiple(millisecond multiple=u32 50 ("毫秒倍数")) -> ()  [unwired: 1 out]
            }
          }
          frame #3 {
            n193 = while {
              tunnel: w300 -> [w304]
              stop <- w302 stop-if-true
              n194 = call <userlib>:"Acm_AxGetCmdVelocity.vi"("AxisHandle"=w304) -> ("Velocity"=w303:dbl)  [unwired: 1 in, 3 out]
              n195 = Wait Until Next ms Multiple(millisecond multiple=u32 50 ("毫秒倍数")) -> ()  [unwired: 1 out]
              n196 = Equal To 0?(x=w303) -> (x = 0?=w302:bool)
            }
          }
          frame #4 {
            n197 = local write "测头机构轴速度(mm/s)"(30.0 ("测头机构轴速度(mm/s)")) -> ()
          }
          frame #5 {
            n198 = local read "测头机构电机"() -> (w308:u32)
            n199 = local read "测头机构轴检测位"() -> (w306:dbl)
            n200 = while {
              tunnel: w308 -> [w311]
              tunnel: w306 -> [w310]
              tunnel: [w309] -> w307
              stop <- w313 stop-if-true
              n201 = Wait Until Next ms Multiple(millisecond multiple=u32 50 ("毫秒倍数")) -> ()  [unwired: 1 out]
              n202 = call "PCI1220U进给轴位置模式.vi"("Distance"=w310, "AxisHandle IN"=w311) -> ("AbsSuccess"=w313:bool, "AxisHandle OUT"=w309:u32)  [unwired: 8 in]
            }
          }
          frame #6 {
            n203 = while {
              stop <- w317 stop-if-true
              n204 = local read "测头机构轴检测位"() -> (w319:dbl)
              n205 = local read "测头机构轴位置(mm)"() -> (w316:dbl)
              n206 = Wait Until Next ms Multiple(millisecond multiple=u32 50 ("毫秒倍数")) -> ()  [unwired: 1 out]
              n207 = Subtract(x=w319, y=20.0) -> (x-y=w315:dbl)
              n208 = Greater Or Equal?(x=w316, y=w315) -> (x >= y?=w317:bool)
            }
          }
          frame #7 {
            n209 = local write "测头机构轴速度(mm/s)"(10.0 ("测头机构轴速度(mm/s)")) -> ()
          }
          frame #8 {
            n210 = while {
              tunnel: w323 -> [w327]
              stop <- w325 stop-if-true
              n211 = call <userlib>:"Acm_AxGetCmdVelocity.vi"("AxisHandle"=w327) -> ("Velocity"=w326:dbl)  [unwired: 1 in, 3 out]
              n212 = Wait Until Next ms Multiple(millisecond multiple=u32 50 ("毫秒倍数")) -> ()  [unwired: 1 out]
              n213 = Equal To 0?(x=w326) -> (x = 0?=w325:bool)
            }
          }
          frame #9 {
            n214 = local write "旋转齿条轴使能"(TRUE ("旋转齿条轴使能")) -> ()
          }
          frame #10 {
            n215 = local read "旋转齿条电机"() -> (w329:u32)
            n216 = call "PCI1220U角度置零.vi"("AxisHandle IN"=w329) -> ()  [unwired: 10 in, 1 out]
          }
          frame #11 {
            n217 = local write "旋转齿条轴速度(°/s)"(1.0 ("旋转齿条轴速度(°/s)")) -> ()
            n218 = Wait Until Next ms Multiple(millisecond multiple=u32 2000 ("毫秒倍数")) -> ()  [unwired: 1 out]
          }
          frame #12 {
            n219 = while {
              i -> [w336]
              stop <- w334 stop-if-true
              n220 = local read "间隙位移(mm)"() -> (→"基准位移":dbl)
              n221 = Wait Until Next ms Multiple(millisecond multiple=u32 500 ("毫秒倍数")) -> ()  [unwired: 1 out]
              n222 = Greater Or Equal?(x=w336, y=4) -> (x >= y?=w334:bool)
            }
          }
          frame #13 {
            n223 = call "PCI1220U运行.vi"("方向"=enum32{"Negative", "Positive"}."Negative" ("Direction"), "AxisHandle IN"=w340) -> ("AxisHandle OUT"=w339:u32)  [unwired: 9 in]
          }
          frame #14 {
            w345 = dbl[] []
            n224 = while {
              shift-right: [w356] -> w344
              shift-left: w345 -> [w358]
              shift-right: [w355] -> w343
              shift-left: w345 -> [w357]
              stop <- w348 stop-if-true
              n225 = Wait (ms)(milliseconds to wait=u32 10 ("毫秒倍数")) -> ()  [unwired: 1 out]
              n226 = local read "间隙位移(mm)"() -> (w351:dbl)
              n227 = local read "基准位移"() -> (w349:dbl)
              n228 = local read "齿条扭矩(Nm)"() -> (w352:dbl)
              n229 = Subtract(x=w351, y=w349) -> (x-y=w350:dbl)
              n230 = Absolute Value(x=w352) -> (abs(x)=w347:dbl)
              n231 = Build Array (concatenate) ("创建数组")(w357, w350) -> (w355:dbl[])
              n232 = Build Array (concatenate) ("创建数组")(w358, w347) -> (w356:dbl[])
              n233 = Greater Or Equal?(x=w347, y="扭矩停止值") -> (x >= y?=w348:bool)
              n234 = Bundle ("捆绑")(w356, w355) -> (w353:cluster{dbl[], dbl[]})  [unwired: 1 in]
              n235 = Build Array ("创建数组")(w353) -> (w354:cluster{dbl[], dbl[]}[])
              n236 = local write "扭动曲线"(w354) -> ()
            }
          }
          frame #15 {
            n237 = Absolute Value(x=w368) -> (abs(x)=w369:dbl[])
            n238 = local read "测量点扭矩"() -> (w370:dbl)
            n239 = local read "基准位移"() -> (w364:dbl)
            n240 = call "自定义插值.vi"("压力"=w370, "扭矩数组"=w369, "位移数组"=w367) -> ("扭矩值"=w365:dbl)  [unwired: 8 in]
            n241 = Array Max & Min(array=w367) -> (min value=w366:dbl)  [unwired: 3 out]
            n242 = Absolute Value(x=w366) -> (abs(x)=w363:dbl)
            n243 = Subtract(x=w364, y=w363) -> (x-y=w362:dbl)
            n244 = Add(x=w363, y=w365) -> (x+y=w360:dbl)
            n245 = Absolute Value(x=w360) -> (abs(x)=w361:dbl)
            n246 = local write "中间位置间隙"(w361) -> ()
            n247 = local write "基准位移"(w362) -> ()
          }
          frame #16 {
            n248 = while {
              tunnel: w375 -> [w379]
              tunnel: [w378] -> w374
              stop <- w377 stop-if-true
              n249 = call "PCI1220U停止.vi"("AxisHandle IN"=w379) -> ("完成"=w377:bool, "AxisHandle OUT"=w378:u32)  [unwired: 9 in]
              n250 = Wait (ms)(milliseconds to wait=u32 50 ("毫秒倍数")) -> ()  [unwired: 1 out]
            }
            "间隙Y数组" <- w373
            "间隙X数组" <- w372
          }
          frame #17 {
            n251 = while {
              tunnel: [w386] -> w380
              tunnel: w381 -> [w384]
              stop <- w385 stop-if-true
              n252 = Wait Until Next ms Multiple(millisecond multiple=u32 50 ("毫秒倍数")) -> ()  [unwired: 1 out]
              n253 = call "PCI1220U扭矩轴位置模式.vi"("Distance"=0.0, "AxisHandle IN"=w384) -> ("AbsSuccess"=w385:bool, "AxisHandle OUT"=w386:u32)  [unwired: 8 in]
            }
          }
          frame #18 {
            n254 = Wait (ms)(milliseconds to wait=u32 500 ("等待时间（毫秒）")) -> ()  [unwired: 1 out]
          }
          frame #19 {
            n255 = while {
              tunnel: w390 -> [w398]
              tunnel: [w394] -> w389
              stop <- w395 stop-if-true
              n256 = local read "齿条扭矩(Nm)"() -> (w393:dbl)
              n257 = call <userlib>:"Acm_AxGetCmdVelocity.vi"("AxisHandle"=w398) -> ("Velocity"=w399:dbl, "AxisHandle"=w394:u32)  [unwired: 1 in, 2 out]
              n258 = Greater Or Equal?(x=w393, y=3.0) -> (x >= y?=w391:bool)
              n259 = Equal To 0?(x=w399) -> (x = 0?=w396:bool)
              n260 = Or(x=w396, y=w391) -> (x .or. y?=w395:bool)
              n261 = Wait Until Next ms Multiple(millisecond multiple=u32 50 ("毫秒倍数")) -> ()  [unwired: 1 out]
            }
          }
          frame #20 {
            n262 = while {
              tunnel: w400 -> [w404]
              tunnel: [w403] -> _
              stop <- w402 stop-if-true
              n263 = call "PCI1220U停止.vi"("AxisHandle IN"=w404) -> ("完成"=w402:bool, "AxisHandle OUT"=w403:u32)  [unwired: 9 in]
              n264 = Wait (ms)(milliseconds to wait=u32 50 ("毫秒倍数")) -> ()  [unwired: 1 out]
            }
          }
          frame #21 {
            n265 = local write "旋转齿条轴使能"(FALSE ("旋转齿条轴使能")) -> ()
            n266 = Wait (ms)(milliseconds to wait=u32 500 ("毫秒倍数")) -> ()  [unwired: 1 out]
          }
          frame #22 {
            n267 = local write "工步号"(u32 25 ("工步号")) -> ()
          }
        }
      }
      frame 25 {
        n268 = flat-sequence {
          frame #0 {
            n269 = local read "中间位置最大间隙标准(mm)"() -> (w409:dbl)
            n270 = local read "中间位置间隙"() -> (w410:dbl)
            n271 = local read "最小间隙(mm)"() -> (w408:dbl)
            n272 = In Range and Coerce(upper limit=w409, x=w410, lower limit=w408) -> (In Range?=w413:bool)  [unwired: 1 out]
            n273 = case shown="假" w413 {
              tunnel: [FALSE ("本序合格") TRUE ("本序合格")] -> w412
              tunnel: [w418 0.0 ("需调整角度(度)")] -> w411
              tunnel: w410 -> [w416 _]
              tunnel: w409 -> [w415 _]
              tunnel: w408 -> [w414 _]
              frame False {
                n274 = xnode "公式"("X"=w416, "Xmax"=w415, "Xmin"=w414) -> ("结果"=w418:dbl)  [unwired: 1 in, 1 out]
              }
              frame True {
              }
            }
            n275 = local write "单点间隙合格"(w412) -> ()
            n276 = local write "需调整角度(度)"(w411) -> ()
          }
          frame #1 {
            n277 = local read "单点间隙合格"() -> (w433:bool)
            n278 = case shown="假" w433 {
              frame False {
                n279 = local read "单点间隙已调试次数"() -> (w436:dbl)
                n280 = Less?(x=w436, y="间隙设定调整次数") -> (x < y?=w435:bool)
                n281 = case shown="假" w435 {
                  frame False {
                    n282 = local write "工步号"(u32 45 ("变更工步号")) -> ()
                  }
                  frame True {
                    n283 = local write "工步号"(u32 30 ("变更工步号")) -> ()
                  }
                }
              }
              frame True {
                n284 = local write "工步号"(u32 40 ("变更工步号")) -> ()
              }
            }
          }
        }
      }
      frame 30 {
        # "人工调整"
        n285 = flat-sequence {
          tunnel: [w442] -> w440
          tunnel: w440 -> [w449]
          frame #0 {
            n286 = local write "测头机构轴速度(mm/s)"(30.0 ("测头机构轴速度(mm/s)")) -> ()
          }
          frame #1 {
            n287 = local read "测头机构电机"() -> (w443:u32)
            n288 = while {
              tunnel: w443 -> [w446]
              tunnel: [w445] -> w442
              stop <- w448 stop-if-true
              n289 = local read "测头机构轴待检位"() -> (w444:dbl)
              n290 = call "PCI1220U进给轴位置模式.vi"("Distance"=w444, "AxisHandle IN"=w446) -> ("AbsSuccess"=w448:bool, "AxisHandle OUT"=w445:u32)  [unwired: 8 in]
              n291 = Wait Until Next ms Multiple(millisecond multiple=u32 50 ("毫秒倍数")) -> ()  [unwired: 1 out]
            }
          }
          frame #2 {
            n292 = while {
              tunnel: w449 -> [w453]
              stop <- w451 stop-if-true
              n293 = call <userlib>:"Acm_AxGetCmdVelocity.vi"("AxisHandle"=w453) -> ("Velocity"=w452:dbl)  [unwired: 1 in, 3 out]
              n294 = Wait Until Next ms Multiple(millisecond multiple=u32 50 ("毫秒倍数")) -> ()  [unwired: 1 out]
              n295 = Equal To 0?(x=w452) -> (x = 0?=w451:bool)
            }
          }
          frame #3 {
            n296 = while {
              stop <- w455 stop-if-true
              n297 = local read "测头机构轴位置(mm)"() -> (w457:dbl)
              n298 = Wait Until Next ms Multiple(millisecond multiple=u32 50 ("毫秒倍数")) -> ()  [unwired: 1 out]
              n299 = Less Or Equal?(x=w457, y=35.0) -> (x <= y?=w455:bool)
            }
          }
          frame #4 {
            n300 = local write "测头气缸左移"(TRUE ("测头气缸左移")) -> ()
            n301 = local write "测头气缸右移"(FALSE ("测头气缸右移")) -> ()
          }
          frame #5 {
            n302 = while {
              stop <- w460 stop-if-true
              # "等待启动"
              n303 = local read "间隙启动"() -> (w460:bool)
              n304 = Wait Until Next ms Multiple(millisecond multiple=u32 50 ("毫秒倍数")) -> ()  [unwired: 1 out]
            }
          }
          frame #6 {
            n305 = local read "不合格品"() -> (w462:bool)
            n306 = case shown="真" w462 {
              frame False {
                n307 = flat-sequence {
                  frame #0 {
                    n308 = local read "单点间隙已调试次数"() -> (w465:dbl)
                    n309 = local write "测头气缸左移"(FALSE ("测头气缸左移")) -> ()
                    n310 = local write "测头气缸右移"(TRUE ("测头气缸左移")) -> ()
                    n311 = Add(x=w465, y=1.0 ("已调试次数")) -> (x+y=w467:dbl)
                    n312 = local write "单点间隙已调试次数"(w467) -> ()
                  }
                  frame #1 {
                    n313 = while {
                      stop <- w468 stop-if-true
                      n314 = Wait Until Next ms Multiple(millisecond multiple=u32 50 ("毫秒倍数")) -> ()  [unwired: 1 out]
                      n315 = local read "测头右位"() -> (w468:bool)
                    }
                  }
                  frame #2 {
                    n316 = local write "工步号"(u32 20 ("工步号")) -> ()
                  }
                }
              }
              frame True {
                n317 = local write "工步号"(u32 45 ("工步号")) -> ()
              }
            }
          }
        }
      }
      frame 40 {
        n318 = flat-sequence {
          tunnel: [w632] -> w628
          tunnel: w628 -> [w634]
          tunnel: [w633] -> w626
          tunnel: w626 -> [w640]
          tunnel: [w640] -> w479
          tunnel: w479 -> [w650]
          tunnel: [w650] -> w478
          tunnel: w478 -> [w652]
          tunnel: [w651] -> w477
          tunnel: w477 -> [w658]
          tunnel: [w658] -> w480
          tunnel: w480 -> [w667]
          tunnel: [w667] -> w617
          tunnel: w617 -> [w674]
          tunnel: [w674] -> w625
          tunnel: w625 -> [w676]
          tunnel: [w677] -> w562
          tunnel: [w675] -> w561
          tunnel: w562 -> [w688]
          tunnel: [w688] -> w558
          tunnel: w561 -> [w687]
          tunnel: [w687] -> w557
          tunnel: [w685] -> w549
          tunnel: [w684] -> w545
          tunnel: [w683] -> w541
          tunnel: w558 -> [w725]
          tunnel: [w725] -> w556
          tunnel: w557 -> [w724]
          tunnel: [w724] -> w554
          tunnel: [w723] -> w550
          tunnel: w549 -> [w723]
          tunnel: [w722] -> w546
          tunnel: w545 -> [w722]
          tunnel: [w721] -> w542
          tunnel: w541 -> [w721]
          tunnel: w556 -> [w732]
          tunnel: [w732] -> w555
          tunnel: w554 -> [w731]
          tunnel: [w731] -> w553
          tunnel: [w729] -> w551
          tunnel: w550 -> [w729]
          tunnel: [w728] -> w547
          tunnel: w546 -> [w728]
          tunnel: [w727] -> w543
          tunnel: w542 -> [w727]
          tunnel: w555 -> [w738]
          tunnel: [w738] -> w560
          tunnel: w553 -> [w737]
          tunnel: [w733] -> w559
          tunnel: [w736] -> w552
          tunnel: w551 -> [w736]
          tunnel: [w735] -> w548
          tunnel: w547 -> [w735]
          tunnel: [w734] -> w544
          tunnel: w543 -> [w734]
          tunnel: [w752] -> w622
          tunnel: [w751] -> w621
          tunnel: [w750] -> w620
          tunnel: w560 -> [w749]
          tunnel: [w749] -> w619
          tunnel: [w748] -> w618
          tunnel: w559 -> [w747]
          tunnel: w552 -> [w746]
          tunnel: w548 -> [w745]
          tunnel: w544 -> [w744]
          tunnel: w622 -> [w797]
          tunnel: [w797] -> w502
          tunnel: w621 -> [w787]
          tunnel: [w787] -> w500
          tunnel: w620 -> [w800]
          tunnel: [w800] -> w498
          tunnel: w619 -> [w802]
          tunnel: [w802] -> w496
          tunnel: [w799] -> w494
          tunnel: w618 -> [w799]
          tunnel: [w801] -> w492
          tunnel: [w789] -> w490
          tunnel: [w798] -> w488
          tunnel: [w790] -> w486
          tunnel: [w796] -> w484
          tunnel: w502 -> [w818]
          tunnel: [w818] -> w501
          tunnel: w500 -> [w817]
          tunnel: [w817] -> w499
          tunnel: w498 -> [w816]
          tunnel: [w816] -> w497
          tunnel: w496 -> [w815]
          tunnel: [w815] -> w495
          tunnel: w494 -> [w814]
          tunnel: [w814] -> w493
          tunnel: w492 -> [w813]
          tunnel: [w813] -> w491
          tunnel: w490 -> [w812]
          tunnel: [w812] -> w489
          tunnel: w488 -> [w811]
          tunnel: [w811] -> w487
          tunnel: w486 -> [w810]
          tunnel: [w810] -> w485
          tunnel: w484 -> [w809]
          tunnel: [w809] -> w483
          tunnel: w501 -> [w836]
          tunnel: [w836] -> w540
          tunnel: w499 -> [w835]
          tunnel: [w835] -> w539
          tunnel: w497 -> [w834]
          tunnel: [w819] -> w538
          tunnel: w495 -> [w833]
          tunnel: [w833] -> w537
          tunnel: [w832] -> w536
          tunnel: w493 -> [w832]
          tunnel: [w831] -> w535
          tunnel: w491 -> [w831]
          tunnel: w489 -> [w827]
          tunnel: w487 -> [w830]
          tunnel: w485 -> [w828]
          tunnel: w483 -> [w829]
          tunnel: [w829] -> w534
          tunnel: [w821] -> w533
          tunnel: [w820] -> w532
          tunnel: w540 -> [w846]
          tunnel: w539 -> [w845]
          tunnel: w538 -> [w849]
          tunnel: [w848] -> w531
          tunnel: w537 -> [w850]
          tunnel: [w850] -> w530
          tunnel: w536 -> [w847]
          tunnel: [w843] -> w529
          tunnel: w535 -> [w854]
          tunnel: [w854] -> w528
          tunnel: w534 -> [w853]
          tunnel: [w853] -> w527
          tunnel: w533 -> [w852]
          tunnel: [w852] -> w526
          tunnel: w532 -> [w851]
          tunnel: [w851] -> w525
          tunnel: [w844] -> w482
          tunnel: [w842] -> w476
          tunnel: [w891] -> w517
          tunnel: w531 -> [w889]
          tunnel: w530 -> [w897]
          tunnel: [w897] -> w514
          tunnel: w529 -> [w896]
          tunnel: [w896] -> w512
          tunnel: w528 -> [w895]
          tunnel: [w895] -> w510
          tunnel: w527 -> [w894]
          tunnel: [w894] -> w508
          tunnel: w526 -> [w893]
          tunnel: [w893] -> w506
          tunnel: w525 -> [w892]
          tunnel: [w892] -> w504
          tunnel: w482 -> [w891]
          tunnel: w476 -> [w890]
          tunnel: [w890] -> w473
          tunnel: [w889] -> w472
          tunnel: w517 -> [w911]
          tunnel: [w911] -> w516
          tunnel: [w910] -> w515
          tunnel: w514 -> [w909]
          tunnel: [w909] -> w513
          tunnel: w512 -> [w908]
          tunnel: [w908] -> w511
          tunnel: w510 -> [w907]
          tunnel: [w907] -> w509
          tunnel: w508 -> [w906]
          tunnel: [w906] -> w507
          tunnel: w506 -> [w905]
          tunnel: [w905] -> w505
          tunnel: w504 -> [w904]
          tunnel: [w904] -> w503
          tunnel: [w902] -> w474
          tunnel: w473 -> [w902]
          tunnel: w472 -> [w910]
          tunnel: w516 -> [w920]
          tunnel: [w920] -> w524
          tunnel: w515 -> [w912]
          tunnel: w513 -> [w919]
          tunnel: [w919] -> w523
          tunnel: w511 -> [w918]
          tunnel: [w918] -> w522
          tunnel: w509 -> [w917]
          tunnel: [w917] -> w521
          tunnel: w507 -> [w916]
          tunnel: [w916] -> w520
          tunnel: w505 -> [w915]
          tunnel: [w915] -> w519
          tunnel: w503 -> [w914]
          tunnel: [w914] -> w518
          tunnel: [w912] -> w481
          tunnel: [w913] -> w475
          tunnel: w474 -> [w913]
          tunnel: [w937] -> w616
          tunnel: [w936] -> w615
          tunnel: w524 -> [w925]
          tunnel: [w935] -> w613
          tunnel: w523 -> [w928]
          tunnel: [w928] -> w611
          tunnel: w522 -> [w929]
          tunnel: w521 -> [w933]
          tunnel: [w934] -> w609
          tunnel: [w933] -> w607
          tunnel: w520 -> [w932]
          tunnel: [w932] -> w600
          tunnel: w519 -> [w930]
          tunnel: w518 -> [w931]
          tunnel: [w931] -> w582
          tunnel: [w930] -> w581
          tunnel: w481 -> [w927]
          tunnel: w475 -> [w926]
          tunnel: w616 -> [w976]
          tunnel: w615 -> [w984]
          tunnel: [w984] -> w614
          tunnel: w613 -> [w980]
          tunnel: [w980] -> w612
          tunnel: w611 -> [w983]
          tunnel: [w983] -> w610
          tunnel: w609 -> [w982]
          tunnel: [w982] -> w608
          tunnel: w607 -> [w981]
          tunnel: [w981] -> w606
          tunnel: w600 -> [w977]
          tunnel: [w977] -> w599
          tunnel: [w976] -> w598
          tunnel: [w975] -> w597
          tunnel: [w974] -> w596
          tunnel: w582 -> [w972]
          tunnel: w581 -> [w973]
          tunnel: [w973] -> w580
          tunnel: [w972] -> w579
          tunnel: w614 -> [w991]
          tunnel: [w1029] -> w627
          tunnel: w612 -> [w1029]
          tunnel: [w1028] -> w623
          tunnel: w610 -> [w1028]
          tunnel: w608 -> [w1027]
          tunnel: w606 -> [w992]
          tunnel: [w1025] -> w605
          tunnel: w599 -> [w1024]
          tunnel: w598 -> [w1023]
          tunnel: w597 -> [w1021]
          tunnel: w596 -> [w1020]
          tunnel: [w1018] -> w595
          tunnel: [w1017] -> w594
          tunnel: [w1016] -> w593
          tunnel: [w1013] -> w584
          tunnel: [w1012] -> w583
          tunnel: w580 -> [w1011]
          tunnel: w579 -> [w1010]
          tunnel: [w1011] -> w578
          tunnel: [w1010] -> w577
          tunnel: [w1009] -> w572
          tunnel: [w1008] -> w570
          tunnel: [w1005] -> w567
          tunnel: [w1000] -> w565
          tunnel: [w995] -> w563
          tunnel: w627 -> [w1056]
          tunnel: [w1056] -> w592
          tunnel: w623 -> [_]
          tunnel: [w1052] -> w590
          tunnel: w605 -> [w1054]
          tunnel: [w1051] -> w588
          tunnel: w595 -> [w1050]
          tunnel: w594 -> [w1049]
          tunnel: w593 -> [w1048]
          tunnel: [w1047] -> w586
          tunnel: [w1046] -> w585
          tunnel: w584 -> [w1045]
          tunnel: w583 -> [w1044]
          tunnel: w578 -> [w1039]
          tunnel: w577 -> [w1038]
          tunnel: [w1039] -> w576
          tunnel: [w1038] -> w575
          tunnel: [w1037] -> w574
          tunnel: [w1036] -> w573
          tunnel: w572 -> [w1036]
          tunnel: [w1035] -> w571
          tunnel: w570 -> [w1035]
          tunnel: [w1034] -> w569
          tunnel: [w1033] -> w568
          tunnel: w567 -> [w1032]
          tunnel: [w1031] -> w566
          tunnel: w565 -> [w1031]
          tunnel: [w1030] -> w564
          tunnel: w563 -> [w1030]
          tunnel: w592 -> [w1073]
          tunnel: [w1073] -> w591
          tunnel: w590 -> [w1072]
          tunnel: [w1072] -> w589
          tunnel: w588 -> [w1071]
          tunnel: [w1071] -> w587
          tunnel: w586 -> [w1066]
          tunnel: w585 -> [w1065]
          tunnel: w576 -> [w1068]
          tunnel: w575 -> [w1067]
          tunnel: w574 -> [w1064]
          tunnel: w573 -> [w1063]
          tunnel: w571 -> [w1062]
          tunnel: w569 -> [w1061]
          tunnel: w568 -> [w1060]
          tunnel: w566 -> [w1058]
          tunnel: w564 -> [w1057]
          tunnel: w591 -> [w1077]
          tunnel: [w1076] -> w624
          tunnel: w589 -> [w1075]
          tunnel: w587 -> [w1074]
          tunnel: [w1074] -> w602
          tunnel: w624 -> [w1084]
          tunnel: [w1084] -> w604
          tunnel: w602 -> [w1083]
          tunnel: [w1083] -> w601
          tunnel: w604 -> [w1091]
          tunnel: [w1090] -> w603
          tunnel: w601 -> [w1089]
          tunnel: w603 -> [w1097]
          frame #0 {
            n319 = local write "选项卡控件"(T1."轴向力测量" ("选项卡控件")) -> ()
          }
          frame #1 {
            n320 = local write "电动缸速度(mm/s)"(15.0 ("电动缸速度(mm/s)")) -> ()
            n321 = local write "单点间隙已调试次数"(0.0 ("单点间隙已调试次数")) -> ()
            n322 = local read "电动缸电机"() -> (w632:u32)
          }
          frame #2 {
            n323 = while {
              tunnel: w634 -> [w639]
              tunnel: [w638] -> w633
              stop <- w637 stop-if-true
              n324 = local read "齿条左极限"() -> (w635:dbl)
              n325 = Wait (ms)(milliseconds to wait=u32 50 ("毫秒倍数")) -> ()  [unwired: 1 out]
              n326 = call "PCI1240电动缸位置模式 .vi"("Distance"=w635, "AxisHandle IN"=w639) -> ("AbsSuccess"=w637:bool, "AxisHandle OUT"=w638:u32)  [unwired: 8 in]
            }
          }
          frame #3 {
            n327 = while {
              tunnel: w640 -> [w648]
              stop <- w641 stop-if-true
              n328 = local read "齿条推拉力(N)"() -> (w645:dbl)
              n329 = call <userlib>:"Acm_AxGetCmdVelocity.vi"("AxisHandle"=w648) -> ("Velocity"=w647:dbl)  [unwired: 1 in, 3 out]
              n330 = Wait (ms)(milliseconds to wait=u32 50 ("毫秒倍数")) -> ()  [unwired: 1 out]
              n331 = Equal To 0?(x=w647) -> (x = 0?=w643:bool)
              n332 = Less Or Equal?(x=w645, y=-500.0) -> (x <= y?=w642:bool)
              n333 = Or ("或")(x=w643, y=w642) -> (x .or. y?=w641:bool)
            }
          }
          frame #4 {
            n334 = local write "电动缸速度(mm/s)"(1.0 ("电动缸速度(mm/s)")) -> ()
          }
          frame #5 {
            n335 = while {
              tunnel: w652 -> [w657]
              tunnel: [w654] -> w651
              stop <- w655 stop-if-true
              n336 = Wait (ms)(milliseconds to wait=u32 50 ("毫秒倍数")) -> ()  [unwired: 1 out]
              n337 = call "PCI1240电动缸位置模式 .vi"("Distance"=10000.0, "AxisHandle IN"=w657) -> ("AbsSuccess"=w655:bool, "AxisHandle OUT"=w654:u32)  [unwired: 8 in]
            }
          }
          frame #6 {
            n338 = while {
              tunnel: w658 -> [w665]
              stop <- w659 stop-if-true
              n339 = local read "齿条推拉力(N)"() -> (w664:dbl)
              n340 = call <userlib>:"Acm_AxGetCmdVelocity.vi"("AxisHandle"=w665) -> ("Velocity"=w662:dbl)  [unwired: 1 in, 3 out]
              n341 = Wait (ms)(milliseconds to wait=u32 50 ("毫秒倍数")) -> ()  [unwired: 1 out]
              n342 = Less Or Equal?(x=w664, y=-500.0) -> (x <= y?=w660:bool)
              n343 = Equal To 0?(x=w662) -> (x = 0?=w661:bool)
              n344 = Or ("或")(x=w661, y=w660) -> (x .or. y?=w659:bool)
            }
          }
          frame #7 {
            n345 = while {
              tunnel: w667 -> [w671]
              tunnel: [w670] -> _
              stop <- w669 stop-if-true
              n346 = call "PCI1220U停止.vi"("AxisHandle IN"=w671) -> ("完成"=w669:bool, "AxisHandle OUT"=w670:u32)  [unwired: 9 in]
              n347 = Wait (ms)(milliseconds to wait=u32 50 ("毫秒倍数")) -> ()  [unwired: 1 out]
            }
          }
          frame #8 {
            n348 = Wait Until Next ms Multiple(millisecond multiple=u32 50 ("毫秒倍数")) -> ()  [unwired: 1 out]
            n349 = local write "电动缸速度(mm/s)"(15.0 ("电动缸速度(mm/s)")) -> ()
          }
          frame #9 {
            n350 = while {
              tunnel: w676 -> [w682]
              tunnel: [w679] -> w675
              stop <- w680 stop-if-true
              n351 = local read "齿条右极限"() -> (w678:dbl)
              n352 = Wait (ms)(milliseconds to wait=u32 50 ("毫秒倍数")) -> ()  [unwired: 1 out]
              n353 = call "PCI1240电动缸位置模式 .vi"("Distance"=w678, "AxisHandle IN"=w682) -> ("AbsSuccess"=w680:bool, "AxisHandle OUT"=w679:u32)  [unwired: 8 in]
            }
            n354 = local read "转向器中心"() -> (w677:dbl)
          }
          frame #10 {
            w686 = dbl[] []
            n355 = while {
              shift-right: [w708] -> w684
              shift-left: w686 -> [w719]
              shift-right: [w717] -> w685
              shift-left: w686 -> [w718]
              tunnel: w687 -> [w713]
              tunnel: [w713] -> _
              tunnel: w688 -> [w711]
              shift-right: [w707] -> w683
              shift-left: w686 -> [w709]
              stop <- w701 stop-if-true
              n356 = local read "中间位置间隙"() -> (w698:dbl)
              n357 = local read "基准位移"() -> (w714:dbl)
              n358 = local read "间隙位移(mm)"() -> (w697:dbl)
              n359 = call <userlib>:"Acm_AxGetCmdVelocity.vi"("AxisHandle"=w713) -> ("Velocity"=w706:dbl)  [unwired: 1 in, 3 out]
              n360 = Wait (ms)(milliseconds to wait=u32 40 ("毫秒倍数")) -> ()  [unwired: 1 out]
              n361 = local read "齿条推拉力(N)"() -> (w704:dbl)
              n362 = call "PCI1240电动缸读取位置.vi"("AxisHandle IN"=w713) -> ("位置"=w712:dbl)  [unwired: 9 in, 1 out]
              n363 = Subtract(x=w697, y=w714) -> (x-y=w700:dbl)
              n364 = Subtract(x=w712, y=w711) -> (x-y=w691:dbl)
              n365 = Add(x=w700, y=w698) -> (x+y=w699:dbl)
              n366 = Multiply(x=w691, y=1.0) -> (x*y=w689:dbl)
              n367 = Build Array (concatenate) ("创建数组")(w718, w699) -> (w717:dbl[])
              n368 = Build Array (concatenate) ("创建数组")(w719, w689) -> (w708:dbl[])
              n369 = Build Array (concatenate) ("创建数组")(w709, w704) -> (w707:dbl[])
              n370 = Greater Or Equal?(x=w704, y=500.0) -> (x >= y?=w702:bool)
              n371 = Less Or Equal?(x=w697, y=-1.0) -> (x <= y?=w696:bool)
              n372 = Greater Or Equal?(x=w697, y=4.0) -> (x >= y?=w695:bool)
              n373 = Equal To 0?(x=w706) -> (x = 0?=w703:bool)
              n374 = Or(x=w695, y=w696) -> (x .or. y?=w694:bool)
              n375 = Bundle ("捆绑")(w708, w717) -> (w715:cluster{dbl[], dbl[]})  [unwired: 1 in]
              n376 = Or(x=w703, y=w702) -> (x .or. y?=w701:bool)
              n377 = Bundle ("捆绑")(w708, w707) -> (w710:cluster{dbl[], dbl[]})  [unwired: 1 in]
              n378 = property on="间隙位移(mm)" class="DigNum (严格)"("Blinking"=w694) -> ()  [unwired: 2 in, 2 out]
              n379 = Build Array ("创建数组")(w715, w710) -> (w716:cluster{dbl[], dbl[]}[])
              n380 = local write "行程跳动曲线"(w716) -> ()
            }
          }
          frame #11 {
            n381 = disable-structure shown="禁用" {
              disable-tunnel: w724 -> [w726 _]
              frame Disabled {
                n382 = call "PCI1220U停止.vi"("AxisHandle IN"=w726) -> ()  [unwired: 9 in, 2 out]
              }
              frame Enabled {
              }
            }
          }
          frame #12 {
            n383 = local write "电动缸速度(mm/s)"(1.0 ("电动缸速度(mm/s)")) -> ()
          }
          frame #13 {
            n384 = while {
              tunnel: w737 -> [w743]
              tunnel: [w740] -> w733
              stop <- w741 stop-if-true
              # "该位置为最右边"
              n385 = Wait (ms)(milliseconds to wait=u32 50 ("毫秒倍数")) -> ()  [unwired: 1 out]
              n386 = call "PCI1240电动缸位置模式 .vi"("Distance"=-10.0, "AxisHandle IN"=w743) -> ("AbsSuccess"=w741:bool, "AxisHandle OUT"=w740:u32)  [unwired: 8 in]
            }
          }
          frame #14 {
            n387 = while {
              shift-right: [w772] -> w751
              shift-left: w745 -> [w783]
              shift-right: [w781] -> w752
              shift-left: w746 -> [w782]
              tunnel: w747 -> [w777]
              tunnel: [w777] -> w750
              tunnel: w749 -> [w775]
              shift-right: [w771] -> w748
              shift-left: w744 -> [w773]
              stop <- w765 stop-if-true
              n388 = local read "中间位置间隙"() -> (w762:dbl)
              n389 = local read "基准位移"() -> (w778:dbl)
              n390 = local read "间隙位移(mm)"() -> (w761:dbl)
              n391 = call <userlib>:"Acm_AxGetCmdVelocity.vi"("AxisHandle"=w777) -> ("Velocity"=w770:dbl)  [unwired: 1 in, 3 out]
              n392 = Wait (ms)(milliseconds to wait=u32 40 ("毫秒倍数")) -> ()  [unwired: 1 out]
              n393 = local read "齿条推拉力(N)"() -> (w768:dbl)
              n394 = call "PCI1240电动缸读取位置.vi"("AxisHandle IN"=w777) -> ("位置"=w776:dbl)  [unwired: 9 in, 1 out]
              n395 = Subtract(x=w761, y=w778) -> (x-y=w764:dbl)
              n396 = Subtract(x=w776, y=w775) -> (x-y=w755:dbl)
              n397 = Add(x=w764, y=w762) -> (x+y=w763:dbl)
              n398 = Multiply(x=w755, y=1.0) -> (x*y=w753:dbl)
              n399 = Build Array (concatenate) ("创建数组")(w782, w763) -> (w781:dbl[])
              n400 = Build Array (concatenate) ("创建数组")(w783, w753) -> (w772:dbl[])
              n401 = Build Array (concatenate) ("创建数组")(w773, w768) -> (w771:dbl[])
              n402 = Greater Or Equal?(x=w768, y=500.0) -> (x >= y?=w766:bool)
              n403 = Less Or Equal?(x=w761, y=-1.0) -> (x <= y?=w760:bool)
              n404 = Greater Or Equal?(x=w761, y=4.0) -> (x >= y?=w759:bool)
              n405 = Equal To 0?(x=w770) -> (x = 0?=w767:bool)
              n406 = Or(x=w759, y=w760) -> (x .or. y?=w758:bool)
              n407 = Bundle ("捆绑")(w772, w781) -> (w779:cluster{dbl[], dbl[]})  [unwired: 1 in]
              n408 = Or(x=w767, y=w766) -> (x .or. y?=w765:bool)
              n409 = Bundle ("捆绑")(w772, w771) -> (w774:cluster{dbl[], dbl[]})  [unwired: 1 in]
              n410 = property on="间隙位移(mm)" class="DigNum (严格)"("Blinking"=w758) -> ()  [unwired: 2 in, 2 out]
              n411 = Build Array ("创建数组")(w779, w774) -> (w780:cluster{dbl[], dbl[]}[])
              n412 = local write "行程跳动曲线"(w780) -> ()
            }
          }
          frame #15 {
            n413 = while {
              tunnel: w800 -> [w807]
              tunnel: [w806] -> _
              stop <- w805 stop-if-true
              n414 = call "PCI1220U停止.vi"("AxisHandle IN"=w807) -> ("完成"=w805:bool, "AxisHandle OUT"=w806:u32)  [unwired: 9 in]
              n415 = Wait (ms)(milliseconds to wait=u32 50 ("毫秒倍数")) -> ()  [unwired: 1 out]
            }
            n416 = Array Size(array=w799) -> (size(s)=w801:i32)
            n417 = Array Size(array=w797) -> (size(s)=w796:i32)
            n418 = call "功能计算_何 截取位移左.vi"("位移数组"=w787, "拉压力数组"=w799, "半行程"="半行程", "截取百分比"="截取百分比") -> ("峰值扭矩"=w789:dbl, "平均扭矩"=w798:dbl, "扭差"=w790:dbl)  [unwired: 12 in, 1 out]
            "左轴向力波动(N)" <- w790
            "左最大轴向力(N)" <- w789
            n419 = call "间隙计算.vi"("扭矩数组"=w797) -> ("峰值间隙1"=w795:dbl, "峰值间隙2"=w794:dbl)  [unwired: 6 in, 3 out]
            n420 = local read "180°内全行程间隙标准(mm)"() -> (w793:dbl)
            n421 = local read "180°外全行程间隙标准(mm)"() -> (w788:dbl)
            n422 = local write "左平均轴向力(N)"(w798) -> ()
            n423 = local write "左180°外全行程间隙"(w794) -> ()
            n424 = local write "左180°内全行程间隙"(w795) -> ()
            n425 = disable-structure shown="禁用" {
              frame Disabled {
                n426 = Wait Until Next ms Multiple(millisecond multiple=u32 500 ("毫秒倍数")) -> ()  [unwired: 1 out]
              }
              frame Enabled {
              }
            }
            n427 = Greater?(x=w795, y=w793) -> (0:w792:bool)
            n428 = Greater?(x=w794, y=w788) -> (0:w791:bool)
            n429 = property on="左180°内全行程间隙" class="DigNum (严格)"("Blinking"=w792) -> ()  [unwired: 2 in, 2 out]
            n430 = property on="左180°外全行程间隙" class="DigNum (严格)"("Blinking"=w791) -> ()  [unwired: 2 in, 2 out]
          }
          frame #16 {
            n431 = local write "电动缸速度(mm/s)"(15.0 ("电动缸速度(mm/s)")) -> ()
          }
          frame #17 {
            n432 = while {
              tunnel: w834 -> [w841]
              tunnel: w833 -> [_]
              tunnel: [w837] -> w819
              stop <- w840 stop-if-true
              n433 = Wait (ms)(milliseconds to wait=u32 50 ("毫秒倍数")) -> ()  [unwired: 1 out]
              n434 = local read "齿条左极限"() -> (w838:dbl)
              n435 = call "PCI1240电动缸位置模式 .vi"("Distance"=w838, "AxisHandle IN"=w841) -> ("AbsSuccess"=w840:bool, "AxisHandle OUT"=w837:u32)  [unwired: 8 in]
            }
            n436 = local read "齿条传动比"() -> (w825:dbl)
            n437 = local read "轴向力标准(N)"() -> (w824:dbl)
            n438 = local read "平均轴向力标准(N) max"() -> (w823:dbl)
            n439 = local read "力波动标准(N)"() -> (w822:dbl)
            n440 = call "判断.vi"("y 3"=w822, "y 2-2"=w823, "y 2-1"=w824, "y"=w825, "x 3"=w828, "x 2"=w830, "x"=w827) -> ("非x? 3"=w820:bool, "非x? 2"=w826:bool, "非x?"=w821:bool)  [unwired: 2 in]
            n441 = property on="左最大轴向力(N)" class="DigNum (严格)"("Blinking"=w821) -> ()  [unwired: 2 in, 2 out]
            n442 = property on="左平均轴向力(N)" class="DigNum (严格)"("Blinking"=w826) -> ()  [unwired: 2 in, 2 out]
            n443 = property on="左轴向力波动(N)" class="DigNum (严格)"("Blinking"=w820) -> ()  [unwired: 2 in, 2 out]
          }
          frame #18 {
            n444 = while {
              shift-right: [w877] -> w842
              shift-left: w845 -> [w887]
              shift-right: [w885] -> w844
              shift-left: w846 -> [w886]
              tunnel: w849 -> [w880]
              tunnel: [w880] -> w848
              tunnel: w850 -> [w878]
              shift-right: [w874] -> w843
              shift-left: w847 -> [w875]
              stop <- w869 stop-if-true
              n445 = call <userlib>:"Acm_AxGetCmdVelocity.vi"("AxisHandle"=w880) -> ("Velocity"=w867:dbl)  [unwired: 1 in, 3 out]
              n446 = local read "间隙位移(mm)"() -> (w861:dbl)
              n447 = local read "基准位移"() -> (w881:dbl)
              n448 = Wait (ms)(milliseconds to wait=u32 40 ("毫秒倍数")) -> ()  [unwired: 1 out]
              n449 = local read "中间位置间隙"() -> (w866:dbl)
              n450 = local read "齿条推拉力(N)"() -> (w873:dbl)
              n451 = call "PCI1240电动缸读取位置.vi"("AxisHandle IN"=w880) -> ("位置"=w879:dbl)  [unwired: 9 in, 1 out]
              n452 = Add(x=1.47, y=w879) -> (x+y=w856:dbl)
              n453 = Subtract(x=w861, y=w881) -> (x-y=w882:dbl)
              n454 = Subtract(x=w856, y=w878) -> (x-y=w859:dbl)
              n455 = Add(x=w882, y=w866) -> (x+y=w868:dbl)
              n456 = Multiply(x=w859, y=1.0) -> (x*y=w857:dbl)
              n457 = Build Array (concatenate) ("创建数组")(w887, w857) -> (w877:dbl[])
              n458 = Less Or Equal?(x=w873, y=-500.0) -> (x <= y?=w870:bool)
              n459 = Build Array (concatenate) ("创建数组")(w875, w873) -> (w874:dbl[])
              n460 = Equal To 0?(x=w867) -> (x = 0?=w871:bool)
              n461 = Build Array (concatenate) ("创建数组")(w886, w868) -> (w885:dbl[])
              n462 = Bundle ("捆绑")(w877, w874) -> (w876:cluster{dbl[], dbl[]})  [unwired: 1 in]
              n463 = Or(x=w871, y=w870) -> (x .or. y?=w869:bool)
              n464 = Bundle ("捆绑")(w877, w885) -> (w883:cluster{dbl[], dbl[]})  [unwired: 1 in]
              n465 = Build Array ("创建数组")(w883, w876) -> (w884:cluster{dbl[], dbl[]}[])
              n466 = Less Or Equal?(x=w861, y=-1.0) -> (x <= y?=w865:bool)
              n467 = Greater Or Equal?(x=w861, y=4.0) -> (x >= y?=w864:bool)
              n468 = local write "行程跳动曲线"(w884) -> ()
              n469 = Or(x=w864, y=w865) -> (x .or. y?=w860:bool)
              n470 = property on="间隙位移(mm)" class="DigNum (严格)"("Blinking"=w860) -> ()  [unwired: 2 in, 2 out]
            }
          }
          frame #19 {
            n471 = disable-structure shown="禁用" {
              disable-tunnel: w889 -> [w898 _]
              frame Disabled {
                n472 = while {
                  tunnel: w898 -> [w901]
                  stop <- w900 stop-if-true
                  n473 = call "PCI1220U停止.vi"("AxisHandle IN"=w901) -> ("完成"=w900:bool)  [unwired: 9 in, 1 out]
                  n474 = Wait (ms)(milliseconds to wait=u32 50 ("毫秒倍数")) -> ()  [unwired: 1 out]
                }
              }
              frame Enabled {
              }
            }
          }
          frame #20 {
            n475 = local write "电动缸速度(mm/s)"(1.0 ("电动缸速度(mm/s)")) -> ()
          }
          frame #21 {
            n476 = while {
              tunnel: w912 -> [w924]
              stop <- w922 stop-if-true
              # "该位置为最左边"
              n477 = Wait (ms)(milliseconds to wait=u32 50 ("毫秒倍数")) -> ()  [unwired: 1 out]
              n478 = call "PCI1240电动缸位置模式 .vi"("Distance"=160.0, "AxisHandle IN"=w924) -> ("AbsSuccess"=w922:bool)  [unwired: 8 in, 1 out]
            }
          }
          frame #22 {
            n479 = while {
              shift-right: [w960] -> w936
              shift-left: w926 -> [w970]
              shift-right: [w968] -> w937
              shift-left: w925 -> [w969]
              tunnel: w927 -> [w963]
              tunnel: [w963] -> w935
              tunnel: w928 -> [w961]
              shift-right: [w957] -> w934
              shift-left: w929 -> [w958]
              stop <- w952 stop-if-true
              n480 = call <userlib>:"Acm_AxGetCmdVelocity.vi"("AxisHandle"=w963) -> ("Velocity"=w950:dbl)  [unwired: 1 in, 3 out]
              n481 = local read "间隙位移(mm)"() -> (w944:dbl)
              n482 = local read "基准位移"() -> (w964:dbl)
              n483 = Wait (ms)(milliseconds to wait=u32 40 ("毫秒倍数")) -> ()  [unwired: 1 out]
              n484 = local read "中间位置间隙"() -> (w949:dbl)
              n485 = local read "齿条推拉力(N)"() -> (w956:dbl)
              n486 = call "PCI1240电动缸读取位置.vi"("AxisHandle IN"=w963) -> ("位置"=w962:dbl)  [unwired: 9 in, 1 out]
              n487 = Subtract(x=w944, y=w964) -> (x-y=w965:dbl)
              n488 = Add(x=1.45, y=w962) -> (x+y=w939:dbl)
              n489 = Subtract(x=w939, y=w961) -> (x-y=w942:dbl)
              n490 = Add(x=w965, y=w949) -> (x+y=w951:dbl)
              n491 = Multiply(x=w942, y=1.0) -> (x*y=w940:dbl)
              n492 = Build Array (concatenate) ("创建数组")(w970, w940) -> (w960:dbl[])
              n493 = Less Or Equal?(x=w956, y=-500.0) -> (x <= y?=w953:bool)
              n494 = Build Array (concatenate) ("创建数组")(w958, w956) -> (w957:dbl[])
              n495 = Equal To 0?(x=w950) -> (x = 0?=w954:bool)
              n496 = Build Array (concatenate) ("创建数组")(w969, w951) -> (w968:dbl[])
              n497 = Bundle ("捆绑")(w960, w957) -> (w959:cluster{dbl[], dbl[]})  [unwired: 1 in]
              n498 = Or(x=w954, y=w953) -> (x .or. y?=w952:bool)
              n499 = Bundle ("捆绑")(w960, w968) -> (w966:cluster{dbl[], dbl[]})  [unwired: 1 in]
              n500 = Build Array ("创建数组")(w966, w959) -> (w967:cluster{dbl[], dbl[]}[])
              n501 = Less Or Equal?(x=w944, y=-1.0) -> (x <= y?=w948:bool)
              n502 = Greater Or Equal?(x=w944, y=4.0) -> (x >= y?=w947:bool)
              n503 = local write "行程跳动曲线"(w967) -> ()
              n504 = Or(x=w947, y=w948) -> (x .or. y?=w943:bool)
              n505 = property on="间隙位移(mm)" class="DigNum (严格)"("Blinking"=w943) -> ()  [unwired: 2 in, 2 out]
            }
          }
          frame #23 {
            n506 = while {
              tunnel: w980 -> [w988]
              tunnel: [w987] -> _
              stop <- w986 stop-if-true
              n507 = call "PCI1220U停止.vi"("AxisHandle IN"=w988) -> ("完成"=w986:bool, "AxisHandle OUT"=w987:u32)  [unwired: 9 in]
              n508 = Wait (ms)(milliseconds to wait=u32 50 ("毫秒倍数")) -> ()  [unwired: 1 out]
            }
            n509 = Array Max & Min(array=w976) -> (max value=w979:dbl, min value=w978:dbl)  [unwired: 2 out]
            n510 = Absolute Value(x=w979) -> (abs(x)=w975:dbl)
            n511 = Absolute Value(x=w978) -> (abs(x)=w974:dbl)
            n512 = local write "左全行程间隙"(w975) -> ()
            n513 = local write "右全行程间隙"(w974) -> ()
          }
          frame #24 {
            n514 = local read "180°内全行程间隙标准(mm)"() -> (w1019:dbl)
            n515 = local read "截取百分比"() -> (w989:dbl)
            n516 = local read "齿条传动比"() -> (w994:dbl)
            n517 = local read "半行程"() -> (w990:dbl)
            n518 = Split 1D Array(array=w1027, index=w992) -> (second subarray=w1026:dbl[])  [unwired: 1 out]
            n519 = Split 1D Array(array=w991, index=w992) -> (second subarray=w993:dbl[])  [unwired: 1 out]
            n520 = Array Max & Min(array=w991) -> (max value=w1015:dbl, min value=w1014:dbl)  [unwired: 2 out]
            n521 = local read "机械间隙值"() -> (w1006:dbl)
            n522 = local read "总圈数标准"() -> (w998:dbl)
            n523 = local read "总圈数最大值"() -> (w999:dbl)
            n524 = Subtract(x=w1015, y=w1014) -> (x-y=w1007:dbl)
            n525 = call "功能计算_何 截取位移右.vi"("位移数组"=w993, "拉压力数组"=w1026, "半行程"=w990, "截取百分比"=w989) -> ("峰值扭矩"=w1013:dbl, "平均扭矩"=w1025:dbl, "扭差"=w1012:dbl)  [unwired: 12 in, 1 out]
            n526 = Subtract(x=w1007, y=w1006) -> (x-y=w1004:dbl)
            n527 = Split 1D Array(array=w1023, index=w1024) -> (second subarray=w1022:dbl[])  [unwired: 1 out]
            n528 = Greater?(x=w1021, y=w1019) -> (0:w1009:bool)
            n529 = Greater?(x=w1020, y=w1019) -> (0:w1008:bool)
            n530 = local write "右最大轴向力(N)"(w1013) -> ()
            n531 = call "间隙计算.vi"("扭矩数组"=w1022) -> ("峰值间隙1"=w1017:dbl, "峰值间隙2"=w1016:dbl)  [unwired: 6 in, 3 out]
            n532 = Divide(x=w1004, y=w994) -> (x/y=w997:dbl)
            n533 = In Range and Coerce(upper limit=w999, x=w997, lower limit=w998) -> (In Range?=w996:bool)  [unwired: 1 out]
            n534 = Not(x=w996) -> (.not. x?=w995:bool)
            n535 = property on="总圈数" class="DigNum (严格)"("Blinking"=w995) -> ()  [unwired: 2 in, 2 out]
            n536 = property on="左全行程间隙" class="DigNum (严格)"("Blinking"=w1009) -> ()  [unwired: 2 in, 2 out]
            n537 = property on="右全行程间隙" class="DigNum (严格)"("Blinking"=w1008) -> ()  [unwired: 2 in, 2 out]
            n538 = local write "右平均轴向力(N)"(w1025) -> ()
            n539 = local write "右轴向力波动(N)"(w1012) -> ()
            n540 = local write "总圈数"(w997) -> ()
            n541 = local read "180°内全行程间隙标准(mm)"() -> (w1018:dbl)
            n542 = local read "总行程标准(mm)"() -> (w1002:dbl)
            n543 = local read "总行程最大值"() -> (w1003:dbl)
            n544 = In Range and Coerce(upper limit=w1003, x=w1004, lower limit=w1002) -> (In Range?=w1001:bool)  [unwired: 1 out]
            n545 = local write "右180°外全行程间隙"(w1016) -> ()
            n546 = local write "右180°内全行程间隙"(w1017) -> ()
            n547 = local read "180°外全行程间隙标准(mm)"() -> (w1005:dbl)
            n548 = Not(x=w1001) -> (.not. x?=w1000:bool)
            n549 = local write "总行程"(w1004) -> ()
            n550 = property on="总行程" class="DigNum (严格)"("Blinking"=w1000) -> ()  [unwired: 2 in, 2 out]
            "轴向力X" <- w991
            "轴向力Y" <- w1027
          }
          frame #25 {
            n551 = local read "齿条传动比"() -> (w1043:dbl)
            n552 = local read "轴向力标准(N)"() -> (w1042:dbl)
            n553 = local read "平均轴向力标准(N) max"() -> (w1041:dbl)
            n554 = Greater?(x=w1049, y=w1050) -> (0:w1034:bool)
            n555 = Greater?(x=w1048, y=w1032) -> (0:w1033:bool)
            n556 = local write "电动缸速度(mm/s)"(15.0 ("电动缸速度(mm/s)")) -> ()
            n557 = local read "转向器中心"() -> (w1051:dbl)
            n558 = local read "力波动标准(N)"() -> (w1040:dbl)
            n559 = call "判断.vi"("y 3"=w1040, "y 2-2"=w1041, "y 2-1"=w1042, "y"=w1043, "x 3"=w1044, "x 2"=w1054, "x"=w1045) -> ("非x? 3"=w1037:bool, "非x? 2"=w1046:bool, "非x?"=w1047:bool)  [unwired: 2 in]
            n560 = property on="右180°内全行程间隙" class="DigNum (严格)"("Blinking"=w1034) -> ()  [unwired: 2 in, 2 out]
            n561 = property on="右180°外全行程间隙" class="DigNum (严格)"("Blinking"=w1033) -> ()  [unwired: 2 in, 2 out]
            n562 = Add(x=w1051, y=-10.0) -> (x+y=w1052:dbl)
          }
          frame #26 {
            n563 = Compound Arithmetic op=OR(w1063, w1062, w1061, w1060) -> (w1059:bool)
            n564 = property on="右最大轴向力(N)" class="DigNum (严格)"("Blinking"=w1066) -> ()  [unwired: 2 in, 2 out]
            n565 = property on="右平均轴向力(N)" class="DigNum (严格)"("Blinking"=w1065) -> ()  [unwired: 2 in, 2 out]
            n566 = property on="右轴向力波动(N)" class="DigNum (严格)"("Blinking"=w1064) -> ()  [unwired: 2 in, 2 out]
            n567 = Compound Arithmetic op=OR(w1057, w1059, w1066, w1064, w1068, w1067, w1058) -> (w1070:bool)
            n568 = Not(x=w1070) -> (.not. x?=w1069:bool)
            n569 = local write "轴向力及全行程间隙合格"(w1069) -> ()
          }
          frame #27 {
            n570 = while {
              tunnel: w1077 -> [w1081]
              tunnel: [w1079] -> w1076
              tunnel: w1075 -> [w1078]
              stop <- w1080 stop-if-true
              n571 = call "PCI1240电动缸位置模式 .vi"("Distance"=w1078, "AxisHandle IN"=w1081) -> ("AbsSuccess"=w1080:bool, "AxisHandle OUT"=w1079:u32)  [unwired: 8 in]
              n572 = Wait (ms)(milliseconds to wait=u32 50 ("毫秒倍数")) -> ()  [unwired: 1 out]
            }
          }
          frame #28 {
            n573 = while {
              tunnel: w1084 -> [w1088]
              stop <- w1086 stop-if-true
              n574 = call <userlib>:"Acm_AxGetCmdVelocity.vi"("AxisHandle"=w1088) -> ("Velocity"=w1087:dbl)  [unwired: 1 in, 3 out]
              n575 = Wait Until Next ms Multiple(millisecond multiple=u32 50 ("毫秒倍数")) -> ()  [unwired: 1 out]
              n576 = Equal To 0?(x=w1087) -> (x = 0?=w1086:bool)
            }
          }
          frame #29 {
            n577 = while {
              tunnel: w1091 -> [w1095]
              tunnel: [w1093] -> w1090
              tunnel: w1089 -> [w1092]
              stop <- w1094 stop-if-true
              n578 = call "PCI1240电动缸位置模式 .vi"("Distance"=w1092, "AxisHandle IN"=w1095) -> ("AbsSuccess"=w1094:bool, "AxisHandle OUT"=w1093:u32)  [unwired: 8 in]
              n579 = Wait (ms)(milliseconds to wait=u32 50 ("毫秒倍数")) -> ()  [unwired: 1 out]
            }
          }
          frame #30 {
            n580 = while {
              tunnel: w1097 -> [w1101]
              stop <- w1099 stop-if-true
              n581 = call <userlib>:"Acm_AxGetCmdVelocity.vi"("AxisHandle"=w1101) -> ("Velocity"=w1100:dbl)  [unwired: 1 in, 3 out]
              n582 = Wait Until Next ms Multiple(millisecond multiple=u32 50 ("毫秒倍数")) -> ()  [unwired: 1 out]
              n583 = Equal To 0?(x=w1100) -> (x = 0?=w1099:bool)
            }
          }
          frame #31 {
            n584 = local read "轴向力已做次数"() -> (w1104:dbl)
            n585 = Add(x=w1104, y=1.0) -> (x+y=w1102:dbl)
            n586 = local write "轴向力已做次数"(w1102) -> ()
          }
          frame #32 {
            n587 = local read "轴向力及全行程间隙合格"() -> (w1105:bool)
            n588 = case shown="假" w1105 {
              frame False {
                n589 = Less?(x="轴向力已做次数", y="轴向力设定次数") -> (x < y?=w1107:bool)
                n590 = case shown="真" w1107 {
                  frame False {
                    n591 = local write "工步号"(u32 45 ("工步号")) -> ()
                  }
                  frame True {
                    n592 = local write "工步号"(u32 30 ("工步号")) -> ()
                  }
                }
              }
              frame True {
                n593 = local write "工步号"(u32 45 ("工步号")) -> ()
              }
            }
          }
        }
      }
      frame 45 {
        # "测头退回"
        n594 = flat-sequence {
          tunnel: [w1115] -> w1112
          tunnel: w1112 -> [w1122]
          frame #0 {
            n595 = local write "测头机构轴速度(mm/s)"(30.0 ("测头机构轴速度(mm/s)")) -> ()
          }
          frame #1 {
            n596 = local read "测头机构轴后退位"() -> (w1114:dbl)
            n597 = local read "测头机构电机"() -> (w1116:u32)
            n598 = while {
              tunnel: w1116 -> [w1120]
              tunnel: w1114 -> [w1119]
              tunnel: [w1118] -> w1115
              stop <- w1121 stop-if-true
              n599 = Wait Until Next ms Multiple(millisecond multiple=u32 50 ("毫秒倍数")) -> ()  [unwired: 1 out]
              n600 = call "PCI1220U进给轴位置模式.vi"("Distance"=w1119, "AxisHandle IN"=w1120) -> ("AbsSuccess"=w1121:bool, "AxisHandle OUT"=w1118:u32)  [unwired: 8 in]
            }
          }
          frame #2 {
            n601 = while {
              tunnel: w1122 -> [w1126]
              stop <- w1124 stop-if-true
              n602 = call <userlib>:"Acm_AxGetCmdVelocity.vi"("AxisHandle"=w1126) -> ("Velocity"=w1125:dbl)  [unwired: 1 in, 3 out]
              n603 = Wait Until Next ms Multiple(millisecond multiple=u32 50 ("毫秒倍数")) -> ()  [unwired: 1 out]
              n604 = Equal To 0?(x=w1125) -> (x = 0?=w1124:bool)
            }
          }
          frame #3 {
            n605 = while {
              stop <- w1128 stop-if-true
              n606 = local read "测头机构轴位置(mm)"() -> (w1130:dbl)
              n607 = Wait Until Next ms Multiple(millisecond multiple=u32 50 ("毫秒倍数")) -> ()  [unwired: 1 out]
              n608 = Less Or Equal?(x=w1130, y=35.0) -> (x <= y?=w1128:bool)
            }
          }
          frame #4 {
            n609 = local write "测头气缸右移"(FALSE ("测头气缸右移")) -> ()
            n610 = local write "测头气缸左移"(TRUE ("测头气缸左移")) -> ()
          }
          frame #5 {
            n611 = Wait Until Next ms Multiple(millisecond multiple=u32 500 ("毫秒倍数")) -> ()  [unwired: 1 out]
          }
          frame #6 {
            n612 = local write "工步号"(u32 50 ("工步号")) -> ()
          }
        }
      }
      frame 50 {
        n613 = flat-sequence {
          tunnel: [w1157] -> w1146
          tunnel: w1146 -> [w1164]
          tunnel: [w1163] -> w1143
          tunnel: w1143 -> [w1175]
          tunnel: [w1181] -> w1140
          tunnel: w1140 -> [w1184]
          tunnel: [w1183] -> w1139
          tunnel: w1139 -> [w1188]
          tunnel: [w1188] -> w1138
          tunnel: w1138 -> [w1190]
          tunnel: [w1189] -> w1136
          tunnel: [w1196] -> w1137
          tunnel: w1136 -> [w1197]
          tunnel: w1137 -> [w1199]
          tunnel: [w1198] -> w1135
          tunnel: [w1205] -> w1145
          tunnel: w1135 -> [w1205]
          tunnel: w1145 -> [w1208]
          tunnel: [w1207] -> w1144
          tunnel: w1144 -> [w1214]
          tunnel: [w1215] -> w1142
          tunnel: w1142 -> [w1222]
          tunnel: [w1221] -> w1141
          tunnel: w1141 -> [w1232]
          frame #0 {
            n614 = local write "旋转齿条轴速度(°/s)"(15.0 ("调整螺塞轴速度(°/s)")) -> ()
            n615 = local write "测头机构轴速度(mm/s)"(15.0 ("调整机构轴速度(mm/s)")) -> ()
            n616 = local write "电动缸速度(mm/s)"(15.0 ("电动缸速度(mm/s)")) -> ()
            n617 = local write "夹头夹紧"(FALSE ("夹头夹紧")) -> ()
            n618 = local write "夹头松开"(TRUE ("夹头松开")) -> ()
          }
          frame #1 {
            n619 = while {
              stop <- w1152 stop-if-true
              n620 = local read "夹头松开"() -> (w1153:bool)
              n621 = local read "夹头夹紧"() -> (w1155:bool)
              n622 = Wait Until Next ms Multiple(millisecond multiple=u32 50 ("毫秒倍数")) -> ()  [unwired: 1 out]
              n623 = Not(x=w1155) -> (.not. x?=w1154:bool)
              n624 = And(x=w1154, y=w1153) -> (x .and. y?=w1152:bool)
            }
          }
          frame #2 {
            n625 = while {
              tunnel: [w1160] -> w1157
              stop <- w1159 stop-if-true
              n626 = local read "电动缸电机"() -> (w1161:u32)
              n627 = Wait Until Next ms Multiple(millisecond multiple=u32 50 ("毫秒倍数")) -> ()  [unwired: 1 out]
              n628 = local read "齿条右极限"() -> (w1158:dbl)
              n629 = call "PCI1240电动缸位置模式 .vi"("Distance"=w1158, "AxisHandle IN"=w1161) -> ("AbsSuccess"=w1159:bool, "AxisHandle OUT"=w1160:u32)  [unwired: 8 in]
            }
          }
          frame #3 {
            n630 = while {
              tunnel: w1164 -> [w1173]
              tunnel: [w1165] -> w1163
              stop <- w1166 stop-if-true
              n631 = local read "齿条推拉力(N)"() -> (w1171:dbl)
              n632 = Wait Until Next ms Multiple(millisecond multiple=u32 50 ("毫秒倍数")) -> ()  [unwired: 1 out]
              n633 = call <userlib>:"Acm_AxGetCmdVelocity.vi"("AxisHandle"=w1173) -> ("Velocity"=w1174:dbl, "AxisHandle"=w1165:u32)  [unwired: 1 in, 2 out]
              n634 = Equal To 0?(x=w1174) -> (x = 0?=w1168:bool)
              n635 = Absolute Value(x=w1171) -> (abs(x)=w1170:dbl)
              n636 = Greater Or Equal?(x=w1170, y=1000.0) -> (x >= y?=w1167:bool)
              n637 = Or(x=w1168, y=w1167) -> (x .or. y?=w1166:bool)
            }
          }
          frame #4 {
            n638 = while {
              tunnel: w1175 -> [w1179]
              tunnel: [w1178] -> _
              stop <- w1177 stop-if-true
              n639 = call "PCI1220U停止.vi"("AxisHandle IN"=w1179) -> ("完成"=w1177:bool, "AxisHandle OUT"=w1178:u32)  [unwired: 9 in]
              n640 = Wait (ms)(milliseconds to wait=u32 50 ("毫秒倍数")) -> ()  [unwired: 1 out]
            }
          }
          frame #5 {
            n641 = local write "旋转齿条轴使能"(TRUE ("旋转齿条轴使能")) -> ()
          }
          frame #6 {
            n642 = local read "旋转齿条电机"() -> (w1181:u32)
            n643 = Wait Until Next ms Multiple(millisecond multiple=u32 500 ("毫秒倍数")) -> ()  [unwired: 1 out]
          }
          frame #7 {
            n644 = call <userlib>:"Acm_AxHome.vi"("DirMode"=u32 0, "HomeMode"=u32 11, "AxisHandle"=w1184) -> ("AxisHandle"=w1183:u32)  [unwired: 1 in, 2 out]
          }
          frame #8 {
            n645 = Wait Until Next ms Multiple(millisecond multiple=u32 100 ("毫秒倍数")) -> ()  [unwired: 1 out]
          }
          frame #9 {
            n646 = while {
              tunnel: w1190 -> [w1193]
              tunnel: [w1192] -> w1189
              stop <- w1191 stop-if-true
              n647 = call <userlib>:"Acm_AxGetCmdVelocity.vi"("AxisHandle"=w1193) -> ("Velocity"=w1195:dbl, "AxisHandle"=w1192:u32)  [unwired: 1 in, 2 out]
              n648 = Wait Until Next ms Multiple(millisecond multiple=u32 50 ("毫秒倍数")) -> ()  [unwired: 1 out]
              n649 = Equal To 0?(x=w1195) -> (x = 0?=w1191:bool)
            }
          }
          frame #10 {
            n650 = call "PCI1220U角度置零.vi"("AxisHandle IN"=w1197) -> ("AxisHandle OUT"=w1196:u32)  [unwired: 10 in]
          }
          frame #11 {
            n651 = while {
              tunnel: w1199 -> [w1201]
              tunnel: [w1200] -> w1198
              stop <- w1204 stop-if-true
              n652 = Wait Until Next ms Multiple(millisecond multiple=u32 50 ("毫秒倍数")) -> ()  [unwired: 1 out]
              n653 = call "PCI1220U扭矩轴位置模式.vi"("Distance"=10.0, "AxisHandle IN"=w1201) -> ("AbsSuccess"=w1204:bool, "AxisHandle OUT"=w1200:u32)  [unwired: 8 in]
            }
          }
          frame #12 {
            n654 = Wait Until Next ms Multiple(millisecond multiple=u32 500 ("毫秒倍数")) -> ()  [unwired: 1 out]
          }
          frame #13 {
            n655 = while {
              tunnel: w1208 -> [w1211]
              tunnel: [w1210] -> w1207
              stop <- w1209 stop-if-true
              n656 = call <userlib>:"Acm_AxGetCmdVelocity.vi"("AxisHandle"=w1211) -> ("Velocity"=w1213:dbl, "AxisHandle"=w1210:u32)  [unwired: 1 in, 2 out]
              n657 = Wait Until Next ms Multiple(millisecond multiple=u32 50 ("毫秒倍数")) -> ()  [unwired: 1 out]
              n658 = Equal To 0?(x=w1213) -> (x = 0?=w1209:bool)
            }
          }
          frame #14 {
            n659 = call "PCI1220U角度置零.vi"("AxisHandle IN"=w1214) -> ()  [unwired: 10 in, 1 out]
          }
          frame #15 {
            n660 = while {
              tunnel: [w1218] -> w1215
              stop <- w1217 stop-if-true
              n661 = local read "电动缸电机"() -> (w1219:u32)
              n662 = Wait Until Next ms Multiple(millisecond multiple=u32 50 ("毫秒倍数")) -> ()  [unwired: 1 out]
              n663 = local read "齿条右极限"() -> (w1216:dbl)
              n664 = call "PCI1240电动缸位置模式 .vi"("Distance"=w1216, "AxisHandle IN"=w1219) -> ("AbsSuccess"=w1217:bool, "AxisHandle OUT"=w1218:u32)  [unwired: 8 in]
            }
          }
          frame #16 {
            n665 = while {
              tunnel: w1222 -> [w1230]
              tunnel: [w1228] -> w1221
              stop <- w1223 stop-if-true
              n666 = local read "齿条推拉力(N)"() -> (w1227:dbl)
              n667 = Wait Until Next ms Multiple(millisecond multiple=u32 50 ("毫秒倍数")) -> ()  [unwired: 1 out]
              n668 = call <userlib>:"Acm_AxGetCmdVelocity.vi"("AxisHandle"=w1230) -> ("Velocity"=w1231:dbl, "AxisHandle"=w1228:u32)  [unwired: 1 in, 2 out]
              n669 = Equal To 0?(x=w1231) -> (x = 0?=w1225:bool)
              n670 = Greater Or Equal?(x=w1227, y=300.0) -> (x >= y?=w1224:bool)
              n671 = Or(x=w1225, y=w1224) -> (x .or. y?=w1223:bool)
            }
          }
          frame #17 {
            n672 = while {
              tunnel: w1232 -> [w1236]
              tunnel: [w1235] -> _
              stop <- w1234 stop-if-true
              n673 = call "PCI1220U停止.vi"("AxisHandle IN"=w1236) -> ("完成"=w1234:bool, "AxisHandle OUT"=w1235:u32)  [unwired: 9 in]
              n674 = Wait (ms)(milliseconds to wait=u32 50 ("毫秒倍数")) -> ()  [unwired: 1 out]
            }
          }
          frame #18 {
            n675 = local write "工步号"(u32 100 ("工步号")) -> ()
          }
        }
      }
      frame 100 {
        n676 = flat-sequence {
          tunnel: [w1271] -> w1261
          tunnel: [w1269] -> w1260
          tunnel: [w1263] -> w1248
          tunnel: [w1262] -> w1245
          tunnel: w1261 -> [w1278]
          tunnel: w1260 -> [w1275]
          tunnel: ["F:\\报表存储\\" ("字符串")] -> w1259
          tunnel: w1248 -> [w1277]
          tunnel: [w1278] -> w1247
          tunnel: [w1277] -> w1246
          tunnel: w1245 -> [w1276]
          tunnel: [w1276] -> w1244
          tunnel: [w1275] -> w1243
          tunnel: w1259 -> [w1290]
          tunnel: [w1297] -> w1258
          tunnel: [w1295] -> w1257
          tunnel: [w1294] -> w1256
          tunnel: [w1293] -> w1255
          tunnel: w1247 -> [w1289]
          tunnel: w1246 -> [w1288]
          tunnel: w1244 -> [w1287]
          tunnel: w1243 -> [w1280]
          tunnel: [w1282] -> w1238
          tunnel: w1258 -> [w1304]
          tunnel: [w1305] -> w1254
          tunnel: w1257 -> [w1305]
          tunnel: w1256 -> [w1303]
          tunnel: w1255 -> [w1302]
          tunnel: [w1301] -> w1253
          tunnel: [w1300] -> w1252
          tunnel: [w1299] -> w1239
          tunnel: w1238 -> [w1299]
          tunnel: [w1312] -> w1251
          tunnel: w1254 -> [w1312]
          tunnel: w1253 -> [w1311]
          tunnel: [w1311] -> w1250
          tunnel: [w1310] -> w1249
          tunnel: w1252 -> [w1310]
          tunnel: [w1308] -> w1240
          tunnel: w1239 -> [w1308]
          tunnel: w1251 -> [w1315]
          tunnel: w1250 -> [w1323]
          tunnel: w1249 -> [w1322]
          tunnel: [w1314] -> w1241
          tunnel: w1240 -> [w1314]
          tunnel: [w1331] -> w1242
          tunnel: w1241 -> [w1331]
          tunnel: w1242 -> [w1333]
          frame #0 {
            n677 = local read "产品ID"() -> (w1270:string)
            n678 = Format Date/Time String(time format string (%c)="%Y%m%d" ("时间格式字符串(%c)")) -> (date/time string=w1264:string)  [unwired: 2 in]
            n679 = String Subset(string=w1264, offset (0)=6 ("偏移量(0)"), length (rest)=2 ("长度（剩余）")) -> (substring=w1262:string)
            n680 = String Subset(string=w1264, offset (0)=4 ("偏移量(0)"), length (rest)=2 ("长度（剩余）")) -> (substring=w1263:string)
            n681 = String Subset(string=w1264, offset (0)=0 ("偏移量(0)"), length (rest)=4 ("长度（剩余）")) -> (substring=w1271:string)
            n682 = call <vilib>:"Trim Whitespace.vi"("string"=w1270) -> ("trimmed string"=w1269:string)  [unwired: 1 in]
          }
          frame #1 {
          }
          frame #2 {
            w1281 = "\\" ("字符串")
            n683 = Concatenate Strings(w1290, w1289, w1281, w1288, w1281, w1287, w1281, w1280, w1281) -> (w1284:string)
            n684 = Concatenate Strings(w1290, w1289, w1281, w1288, w1281, w1287, w1281, w1280, w1281) -> (w1298:string)
            n685 = Concatenate Strings(w1284, w1280, "间隙曲线.JPG" ("字符串")) -> (w1296:string)
            n686 = Concatenate Strings(w1284, "轴向力曲线数组.txt" ("字符串")) -> (w1293:string)
            n687 = Concatenate Strings(w1284, "扭动曲线数组.txt" ("字符串")) -> (w1294:string)
            n688 = Concatenate Strings(w1284, w1280, "轴向力曲线.JPG" ("字符串")) -> (w1286:string)
            n689 = String To Path(string=w1296) -> (path=w1295:path)
            n690 = String To Path(string=w1298) -> (path=w1297:path)
            n691 = String To Path(string=w1286) -> (path=w1282:path)
          }
          frame #3 {
            n692 = call <vilib>:"Check if File or Folder Exists.vi"("path"=w1304) -> ("file or folder exists?"=w1306:bool)  [unwired: 8 in, 2 out]
            n693 = case shown="假" w1306 {
              tunnel: w1304 -> [w1307 _]
              frame False {
                n694 = Create Folder(path (use dialog)=w1307) -> ()  [unwired: 2 in, 3 out]
              }
              frame True {
              }
            }
            n695 = String To Path(string=w1302) -> (path=w1300:path)
            n696 = String To Path(string=w1303) -> (path=w1301:path)
          }
          frame #4 {
            n697 = local write "选项卡控件"(T1."间隙测量" ("选项卡控件")) -> ()
            n698 = Wait Until Next ms Multiple(millisecond multiple=u32 1000 ("毫秒倍数")) -> ()  [unwired: 1 out]
          }
          frame #5 {
            n699 = disable-structure shown="禁用" {
              disable-tunnel: w1315 -> [w1324 _]
              frame Disabled {
                w1328 = T2 2 items=["快速打印", "标准报表", "HTML", "双字节", "Excel"] ("report type (Quick Print)")
                w1327 = T3 1 items=["完整前面板", "前面板可见部分", "图标、说明、前面板和程序框图", "说明信息: 使用前面板", "说明信息: 作为子VI使用", "说明信息: 完整", "说明信息: 自定义"] ("contents (complete front panel)")
                n700 = Current VI's Path() -> (path=w1326:path)
                n701 = call-poly <vilib>:"Easy Print VI Panel or Documentation.vi"("report type (Quick Print)"=w1328, "contents (complete front panel)"=w1327, "VI path"=w1326) -> ("error out"=w1330:errorcluster, "report out"=w1329:refnum<class "NI_report.lvclass">)  [unwired: 1 in, 6 out]
                n702 = call-dynamic "Save Report to File.vi"("report in"=w1329, "report file path"=w1324, "error in (no error)"=w1330) -> ("error out"=→"error out 3":errorcluster)  [unwired: 2 in, 10 out]
              }
              frame Enabled {
              }
            }
            n703 = local read "间隙Y数组"() -> (w1320:dbl[])
            n704 = local read "间隙X数组"() -> (w1321:dbl[])
            n705 = local read "轴向力Y"() -> (w1318:dbl[])
            n706 = local read "轴向力X"() -> (w1319:dbl[])
            n707 = call "导出曲线数组.vi"("file path (dialog if empty)"=w1323, "数组 2"=w1320, "数组"=w1321) -> ()  [unwired: 9 in]
            n708 = call "导出曲线数组.vi"("file path (dialog if empty)"=w1322, "数组 2"=w1318, "数组"=w1319) -> ()  [unwired: 9 in]
            n709 = control-ref of="本VI"() -> (w1317:refnum<vi>)
            n710 = invoke class="VI" method="FP.Get Image"(reference=w1317) -> ("image data"=w1316:T4)  [unwired: 5 in, 5 out]
            n711 = call <vilib>:"Write JPEG File.vi"("image data"=w1316, "path to JPEG file"=w1315) -> ()  [unwired: 8 in, 2 out]
          }
          frame #6 {
            n712 = local write "选项卡控件"(T1."轴向力测量" ("选项卡控件")) -> ()
          }
          frame #7 {
            n713 = control-ref of="本VI"() -> (w1334:refnum<vi>)
            n714 = invoke class="VI" method="FP.Get Image"(reference=w1334) -> ("image data"=w1335:T4)  [unwired: 5 in, 5 out]
            n715 = call <vilib>:"Write JPEG File.vi"("image data"=w1335, "path to JPEG file"=w1333) -> ()  [unwired: 8 in, 2 out]
          }
          frame #8 {
            n716 = local read "联线按钮"() -> (w1336:bool)
            n717 = case shown="真" w1336 {
              frame False {
              }
              frame True {
                n718 = flat-sequence {
                  tunnel: [w1339] -> w1337
                  tunnel: [w1367] -> w1338
                  tunnel: w1337 -> [w1363]
                  tunnel: w1338 -> [w1379]
                  frame #0 {
                    n719 = local read "轴向力及全行程间隙合格"() -> (w1340:bool)
                    n720 = local read "单点间隙合格"() -> (w1341:bool)
                    n721 = And(x=w1341, y=w1340) -> (x .and. y?=w1339:bool)
                  }
                  frame #1 {
                    w1361 = i16 3 ("精度(6)")
                    n722 = local read "右180°内全行程间隙"() -> (w1360:dbl)
                    n723 = local read "右180°外全行程间隙"() -> (w1353:dbl)
                    n724 = local read "左180°外全行程间隙"() -> (w1352:dbl)
                    n725 = local read "左180°内全行程间隙"() -> (w1370:dbl)
                    n726 = local read "右最大轴向力(N)"() -> (w1355:dbl)
                    n727 = local read "左轴向力波动(N)"() -> (w1356:dbl)
                    n728 = local read "左最大轴向力(N)"() -> (w1354:dbl)
                    n729 = local read "员工ID"() -> (w1342:string)
                    n730 = local read "右轴向力波动(N)"() -> (w1357:dbl)
                    n731 = Boolean To (0,1)(Boolean=w1363) -> (0, 1=w1365:i16)
                    n732 = local read "中间位置间隙"() -> (w1372:dbl)
                    n733 = local read "总圈数"() -> (w1359:dbl)
                    n734 = local read "总行程"() -> (w1358:dbl)
                    n735 = local read "FGCS"() -> (w1374:string)
                    n736 = local read "KSJJ"() -> (w1376:string)
                    n737 = local read "产品ID"() -> (w1377:string)
                    n738 = Number To Decimal String(number=w1365, width (-)=i16 1 ("宽度(-)")) -> (decimal integer string=w1362:string)
                    n739 = Format Date/Time String(time format string (%c)="%Y%m%d%H%M" ("时间格式字符串(%c)")) -> (date/time string=w1375:string)  [unwired: 2 in]
                    n740 = Number To Fractional String(number=w1358, precision (6)=w1361) -> (F-format string=w1344:string)  [unwired: 2 in]
                    n741 = Number To Fractional String(number=w1353, precision (6)=w1361) -> (F-format string=w1349:string)  [unwired: 2 in]
                    n742 = Number To Fractional String(number=w1356, precision (6)=w1361) -> (F-format string=w1346:string)  [unwired: 2 in]
                    n743 = Number To Fractional String(number=w1360, precision (6)=w1361) -> (F-format string=w1351:string)  [unwired: 2 in]
                    n744 = Number To Fractional String(number=w1355, precision (6)=w1361) -> (F-format string=w1347:string)  [unwired: 2 in]
                    n745 = Number To Fractional String(number=w1357, precision (6)=w1361) -> (F-format string=w1345:string)  [unwired: 2 in]
                    n746 = Number To Fractional String(number=w1370, precision (6)=w1361) -> (F-format string=w1368:string)  [unwired: 2 in]
                    n747 = Number To Fractional String(number=w1354, precision (6)=w1361) -> (F-format string=w1348:string)  [unwired: 2 in]
                    n748 = Number To Fractional String(number=w1359, precision (6)=w1361) -> (F-format string=w1343:string)  [unwired: 2 in]
                    n749 = Number To Fractional String(number=w1352, precision (6)=w1361) -> (F-format string=w1350:string)  [unwired: 2 in]
                    n750 = Number To Fractional String(number=w1372, precision (6)=i16 3 ("精度(6)")) -> (F-format string=w1369:string)  [unwired: 2 in]
                    n751 = Build Array(w1377, w1342, "1", w1362, w1376, w1375, w1374, "Q14073-11A", w1369, w1368, w1351, w1350, w1349, w1348, w1347, w1346, w1345, w1344, w1343) -> (w1367:string[])
                  }
                  frame #2 {
                    n752 = Wait (ms)(milliseconds to wait=u32 500 ("等待时间（毫秒）")) -> ()  [unwired: 1 out]
                    n753 = call "数据库更新.vi"("设备号"="06", "数据"=w1379) -> ()  [unwired: 13 in, 1 out]
                  }
                  frame #3 {
                  }
                }
              }
            }
          }
          frame #9 {
            n754 = local write "产品ID"("") -> ()
            n755 = local write "工步号"(u32 0 ("工步号")) -> ()
          }
        }
      }
    }
    n756 = Wait (ms)(milliseconds to wait=u32 50 ("毫秒倍数")) -> ()  [unwired: 1 out]
    n757 = local read "停止"() -> (w7:bool)
  }
  n758 = while {
    stop <- w1384 stop-if-true
    n759 = event shown="[6] \"电动缸回零\": 鼠标按下" {
      selector: _ -> [_ _ _ _ _ _ _]
      dyn-events: _ -> [_ _ _ _ _ _ _]
      timeout: 500 -> [_ _ _ _ _ _ _]
      event Timeout {
        n760 = event-data() -> ()  [unwired: 3 out]
      }
      event "停止": Value Change {
        n761 = event-data() -> ()  [unwired: 6 out]
        n762 = flat-sequence {
          frame #0 {
            n763 = Wait (ms)(milliseconds to wait=u32 1000 ("毫秒倍数")) -> ()  [unwired: 1 out]
          }
          frame #1 {
            n764 = Quit LabVIEW(quit? (T)=TRUE ("停止？(T)")) -> ()
          }
        }
      }
      event "参数修改": Value Change {
        n765 = event-data() -> ()  [unwired: 6 out]
        n766 = while {
          i -> [w1391]
          stop <- w1390 stop-if-true
          n767 = local read "型号数量"() -> (w1392:i32)
          n768 = local read "参数浏览表"() -> (w1393:string[][])
          n769 = Wait Until Next ms Multiple(millisecond multiple=u32 50 ("毫秒倍数")) -> ()  [unwired: 1 out]
          n770 = Greater Or Equal?(x=w1391, y=w1392) -> (x >= y?=w1390:bool)
          n771 = Index Array(array=w1393, index (col)=w1391) -> (element=w1389:string[])  [unwired: 1 in]
          n772 = stacked-sequence {
            tunnel: w1389 -> [w1429]
            frame #0 {
              n773 = Index Array(array=w1429, index #1=0 ("索引"), index #2=2 ("索引"), index #3=3 ("索引"), index #4=4 ("索引"), index #5=5 ("索引"), index #6=6 ("索引"), index #7=7 ("索引"), index #8=8 ("索引"), index #9=9 ("索引"), index #10=10 ("索引"), index #11=11 ("索引"), index #12=12 ("索引"), index #13=13 ("索引"), index #14=14 ("索引"), index #15=15 ("索引"), index #16=16 ("索引"), index #17=17 ("索引"), index #18=18 ("索引"), index #19=19 ("索引"), index #20=20 ("索引")) -> (element #1=w1396:string, element #2=w1425:string, element #3=w1424:string, element #4=w1423:string, element #5=w1422:string, element #6=w1421:string, element #7=w1420:string, element #8=w1419:string, element #9=w1418:string, element #10=w1417:string, element #11=w1416:string, element #12=w1407:string, element #13=w1406:string, element #14=w1405:string, element #15=w1404:string, element #16=w1403:string, element #17=w1402:string, element #18=w1399:string, element #19=w1398:string, element #20=w1395:string)
              n774 = call "创建文本"("测头机构轴移动速度"=w1425, "测头机构轴检测位"=w1424, "测头机构轴待检位"=w1423, "测头机构轴后退位"=w1422, "齿条移动速度"=w1421, "齿条左极限"=w1420, "齿条右极限"=w1419, "旋转齿条轴找帽转速"=w1418, "旋转齿条轴测量转速"=w1417, "测量点扭矩"=w1416, "总行程最小值"=w1407, "总行程最大值"=w1406, "最大轴向力"=w1405, "轴向力波动"=w1404, "平均轴向力最小值"=w1403, "平均轴向力最大值"=w1402, "总圈数最小值"=w1399, "总圈数最大值"=w1398, "中间位置"=w1395, "产品型号"=w1396) -> ("Result"=w1415:string)  [unwired: 6 in, 1 out]
              n775 = local read "ADODB._Connection Out 2"() -> (w1414:refnum<k7>)
              n776 = call "SQL Execute.vi"("Command Text"=w1415, "ADODB._Connection In"=w1414) -> ("error out"=w1427:errorcluster, "ADODB._Connection Out"=w1428:refnum<k7>)  [unwired: 6 in, 2 out]
              n777 = call "ADO Connection Close.vi"("error in (no error)"=w1427, "ADODB._Connection In"=w1428) -> ("error out"=→"error out":errorcluster)  [unwired: 8 in, 1 out]
            }
          }
        }
      }
      event "参数查询": Value Change {
        n778 = event-data() -> ()  [unwired: 6 out]
        n779 = flat-sequence {
          tunnel: [w1452] -> w1445
          tunnel: [w1451] -> w1444
          tunnel: [w1450] -> w1441
          tunnel: w1445 -> [w1456]
          tunnel: w1444 -> [w1458]
          tunnel: [w1458] -> w1443
          tunnel: [w1457] -> w1442
          tunnel: w1441 -> [w1457]
          tunnel: w1443 -> [_]
          tunnel: w1442 -> [_]
          frame #0 {
            n780 = call-poly <vilib>:"Read From Spreadsheet File.vi"("file path (dialog if empty)"=path "D:/Q14070-Z060人机界面/参数/参数项.txt") -> ("first row"=w1446:string[])  [unwired: 6 in, 4 out]
            n781 = property on="参数浏览表" class="Tbl (严格)"("Row Headers[]"=w1446) -> ()  [unwired: 2 in, 2 out]
          }
          frame #1 {
            n782 = local read "ADODB._Connection Out 2"() -> (w1449:refnum<k7>)
            n783 = call "SQL Execute.vi"("Command Text"="SELECT * FROM 测试参数表;", "ADODB._Connection In"=w1449) -> ("error out"=w1450:errorcluster, "Data"=w1454:string[][], "ADODB._Connection Out"=w1451:refnum<k7>)  [unwired: 6 in, 1 out]
            n784 = Transpose 2D Array "二维数组转置"(2D array=w1454) -> (transposed array=w1452:string[][])
            n785 = Index Array(array=w1452, index (row)=0 ("索引 (行)")) -> (element=w1453:string[])  [unwired: 1 in]
            n786 = property on="参数浏览表" class="Tbl (严格)"("Column Headers[]"=w1453) -> ()  [unwired: 2 in, 2 out]
          }
          frame #2 {
            n787 = local write "参数浏览表"(w1456) -> ()
          }
          frame #3 {
          }
        }
      }
      event "传感器参数保存": Value Change {
        n788 = event-data() -> ()  [unwired: 6 out]
        n789 = flat-sequence {
          tunnel: [w1484] -> w1481
          tunnel: [w1483] -> w1480
          tunnel: [w1482] -> w1479
          tunnel: [w1490] -> w1478
          tunnel: w1481 -> [w1490]
          tunnel: [w1489] -> w1477
          tunnel: w1480 -> [w1489]
          tunnel: [w1488] -> w1476
          tunnel: w1479 -> [w1488]
          tunnel: [w1487] -> w1475
          tunnel: [w1486] -> w1474
          tunnel: [w1485] -> w1473
          tunnel: [w1491] -> w1472
          tunnel: [w1497] -> w1471
          tunnel: w1478 -> [w1497]
          tunnel: [w1496] -> w1470
          tunnel: w1477 -> [w1496]
          tunnel: w1476 -> [w1495]
          tunnel: [w1495] -> w1469
          tunnel: [w1494] -> w1468
          tunnel: w1475 -> [w1494]
          tunnel: [w1493] -> w1467
          tunnel: w1474 -> [w1493]
          tunnel: [w1492] -> w1466
          tunnel: w1473 -> [w1492]
          tunnel: w1472 -> [w1516]
          tunnel: [w1516] -> w1465
          tunnel: w1471 -> [w1515]
          tunnel: w1470 -> [w1508]
          tunnel: w1469 -> [w1507]
          tunnel: w1468 -> [w1501]
          tunnel: w1467 -> [w1500]
          tunnel: w1466 -> [w1506]
          tunnel: [w1505] -> w1464
          tunnel: [w1504] -> w1463
          tunnel: [w1503] -> w1462
          tunnel: [w1499] -> w1461
          tunnel: [w1498] -> w1460
          tunnel: [w1502] -> w1459
          tunnel: w1465 -> [w1524]
          tunnel: w1464 -> [w1523]
          tunnel: w1463 -> [w1522]
          tunnel: w1462 -> [w1521]
          tunnel: w1461 -> [w1520]
          tunnel: w1460 -> [w1519]
          tunnel: w1459 -> [w1518]
          frame #0 {
            n790 = local read "齿条推拉力零点偏移"() -> (w1483:dbl)
            n791 = local read "间隙位移零点偏移"() -> (w1484:dbl)
            n792 = local read "齿条扭矩零点偏移"() -> (w1482:dbl)
          }
          frame #1 {
            n793 = local read "齿条推拉力比例偏移"() -> (w1486:dbl)
            n794 = local read "间隙位移比例偏移"() -> (w1487:dbl)
            n795 = local read "齿条扭矩比例偏移"() -> (w1485:dbl)
          }
          frame #2 {
            n796 = local read "ADODB._Connection Out 2"() -> (w1491:refnum<k7>)
          }
          frame #3 {
            n797 = Number To Fractional String(number=w1515, precision (6)=i16 2 ("精度(6)")) -> (F-format string=w1505:string)  [unwired: 2 in]
            n798 = Number To Fractional String(number=w1507, precision (6)=i16 2 ("精度(6)")) -> (F-format string=w1503:string)  [unwired: 2 in]
            n799 = Number To Fractional String(number=w1506, precision (6)=i16 2 ("精度(6)")) -> (F-format string=w1502:string)  [unwired: 2 in]
            n800 = Number To Fractional String(number=w1508, precision (6)=i16 2 ("精度(6)")) -> (F-format string=w1504:string)  [unwired: 2 in]
            n801 = Number To Fractional String(number=w1501, precision (6)=i16 2 ("精度(6)")) -> (F-format string=w1499:string)  [unwired: 2 in]
            n802 = Number To Fractional String(number=w1500, precision (6)=i16 2 ("精度(6)")) -> (F-format string=w1498:string)  [unwired: 2 in]
          }
          frame #4 {
            n803 = call "创建文本3"("4"=w1520, "6"=w1518, "1"=w1523, "2"=w1522, "3"=w1521, "5"=w1519) -> ("Result"=w1525:string)  [unwired: 8 in, 1 out]
            n804 = call "SQL Execute.vi"("Command Text"=w1525, "ADODB._Connection In"=w1524) -> ("error out"=→"error out 4":errorcluster)  [unwired: 6 in, 3 out]
          }
        }
      }
      event "产品ID": Value Change {
        n805 = event-data() -> ()  [unwired: 7 out]
        n806 = Format Date/Time String(time format string (%c)="%Y%m%d%H%M" ("时间格式字符串(%c)")) -> (date/time string=w1526:string)  [unwired: 2 in]
        n807 = local write "KSJJ"(w1526) -> ()
      }
      event "电动缸回零": Mouse Down {
        n808 = event-data() -> ()  [unwired: 6 out]
        n809 = Wait Until Next ms Multiple(millisecond multiple=u32 50 ("毫秒倍数")) -> ()  [unwired: 1 out]
      }
    }
    n810 = Wait (ms)(milliseconds to wait=u32 50 ("毫秒倍数")) -> ()  [unwired: 1 out]
    n811 = local read "停止"() -> (w1384:bool)
  }
  n812 = stacked-sequence {
    frame #0 {
      n813 = flat-sequence {
        tunnel: [w1544] -> w1534
        tunnel: [w1537] -> w1533
        tunnel: w1534 -> [w1547]
        tunnel: [w1547] -> w1532
        tunnel: [w1545] -> w1531
        tunnel: w1533 -> [w1545]
        tunnel: w1532 -> [w1549]
        tunnel: [w1549] -> w1530
        tunnel: w1531 -> [w1548]
        tunnel: [w1548] -> w1529
        tunnel: w1530 -> [w1565]
        tunnel: w1529 -> [w1564]
        frame #0 {
          n814 = local write "电动缸速度(mm/s)"(15.0 ("电动缸速度(mm/s)")) -> ()
          n815 = local write "测头机构轴速度(mm/s)"(10.0 ("电动缸速度(mm/s)")) -> ()
        }
        frame #1 {
          n816 = local read "测头机构电机"() -> (w1541:u32)
          n817 = local read "电动缸电机"() -> (w1538:u32)
          n818 = call <userlib>:"Acm_AxHome.vi"("DirMode"=u32 1, "HomeMode"=u32 11, "AxisHandle"=w1538) -> ("AxisHandle"=w1537:u32)  [unwired: 1 in, 2 out]
          n819 = call <userlib>:"Acm_AxHome.vi"("DirMode"=u32 0, "HomeMode"=u32 11, "AxisHandle"=w1541) -> ("AxisHandle"=w1544:u32)  [unwired: 1 in, 2 out]
        }
        frame #2 {
          n820 = Wait Until Next ms Multiple(millisecond multiple=u32 100 ("毫秒倍数")) -> ()  [unwired: 1 out]
        }
        frame #3 {
          n821 = while {
            tunnel: w1548 -> [w1556]
            stop <- w1551 stop-if-true
            n822 = call <userlib>:"Acm_AxGetCmdVelocity.vi"("AxisHandle"=w1556) -> ("Velocity"=w1555:dbl)  [unwired: 1 in, 3 out]
            n823 = Wait Until Next ms Multiple(millisecond multiple=u32 50 ("毫秒倍数")) -> ()  [unwired: 1 out]
            n824 = Equal To 0?(x=w1555) -> (x = 0?=w1550:bool)
            n825 = local read "急停"() -> (w1552:bool)
            n826 = local read "复位"() -> (w1553:bool)
            n827 = Compound Arithmetic op=OR(invert w1552, w1553, w1550) -> (w1551:bool)
          }
          n828 = while {
            tunnel: w1549 -> [w1563]
            stop <- w1559 stop-if-true
            n829 = call <userlib>:"Acm_AxGetCmdVelocity.vi"("AxisHandle"=w1563) -> ("Velocity"=w1562:dbl)  [unwired: 1 in, 3 out]
            n830 = Wait Until Next ms Multiple(millisecond multiple=u32 50 ("毫秒倍数")) -> ()  [unwired: 1 out]
            n831 = Equal To 0?(x=w1562) -> (x = 0?=w1560:bool)
            n832 = local read "急停"() -> (w1557:bool)
            n833 = local read "复位"() -> (w1558:bool)
            n834 = Compound Arithmetic op=OR(invert w1557, w1558, w1560) -> (w1559:bool)
          }
        }
        frame #4 {
          n835 = call "PCI1220U角度置零.vi"("AxisHandle IN"=w1564) -> ()  [unwired: 10 in, 1 out]
          n836 = call "PCI1220U角度置零.vi"("AxisHandle IN"=w1565) -> ()  [unwired: 10 in, 1 out]
        }
      }
    }
    frame #1 {
      n837 = flat-sequence {
        tunnel: [w1577] -> w1572
        tunnel: w1572 -> [w1579]
        tunnel: [w1579] -> w1571
        tunnel: w1571 -> [w1580]
        tunnel: [w1580] -> w1570
        tunnel: w1570 -> [w1589]
        tunnel: [w1588] -> w1567
        tunnel: w1567 -> [w1591]
        tunnel: [w1591] -> w1566
        tunnel: w1566 -> [w1593]
        tunnel: [w1592] -> w1569
        tunnel: w1569 -> [w1602]
        tunnel: [w1602] -> w1568
        tunnel: w1568 -> [w1610]
        frame #0 {
          n838 = local write "旋转齿条轴速度(°/s)"(5.0 ("电动缸速度(mm/s)")) -> ()
        }
        frame #1 {
          n839 = local read "旋转齿条电机"() -> (w1574:u32)
          n840 = call <userlib>:"Acm_AxHome.vi"("DirMode"=u32 0, "HomeMode"=u32 11, "AxisHandle"=w1574) -> ("AxisHandle"=w1577:u32)  [unwired: 1 in, 2 out]
        }
        frame #2 {
          n841 = Wait Until Next ms Multiple(millisecond multiple=u32 100 ("毫秒倍数")) -> ()  [unwired: 1 out]
        }
        frame #3 {
          n842 = while {
            tunnel: w1580 -> [w1587]
            stop <- w1581 stop-if-true
            n843 = call <userlib>:"Acm_AxGetCmdVelocity.vi"("AxisHandle"=w1587) -> ("Velocity"=w1586:dbl)  [unwired: 1 in, 3 out]
            n844 = Wait Until Next ms Multiple(millisecond multiple=u32 50 ("毫秒倍数")) -> ()  [unwired: 1 out]
            n845 = Equal To 0?(x=w1586) -> (x = 0?=w1582:bool)
            n846 = local read "急停"() -> (w1584:bool)
            n847 = local read "复位"() -> (w1583:bool)
            n848 = Compound Arithmetic op=OR(invert w1584, w1583, w1582) -> (w1581:bool)
          }
        }
        frame #4 {
          n849 = call "PCI1220U角度置零.vi"("AxisHandle IN"=w1589) -> ("AxisHandle OUT"=w1588:u32)  [unwired: 10 in]
        }
        frame #5 {
          n850 = Wait (ms)(milliseconds to wait=u32 100 ("等待时间（毫秒）")) -> ()  [unwired: 1 out]
        }
        frame #6 {
          n851 = while {
            tunnel: [w1600] -> w1592
            tunnel: w1593 -> [w1598]
            stop <- w1595 stop-if-true
            n852 = call "PCI1220U扭矩轴位置模式.vi"("Distance"=10.0, "AxisHandle IN"=w1598) -> ("AbsSuccess"=w1594:bool, "AxisHandle OUT"=w1600:u32)  [unwired: 8 in]
            n853 = Wait Until Next ms Multiple(millisecond multiple=u32 50 ("毫秒倍数")) -> ()  [unwired: 1 out]
            n854 = local read "急停"() -> (w1597:bool)
            n855 = local read "复位"() -> (w1596:bool)
            n856 = Compound Arithmetic op=OR(invert w1597, w1596, w1594) -> (w1595:bool)
          }
        }
        frame #7 {
          n857 = while {
            tunnel: w1602 -> [w1608]
            stop <- w1603 stop-if-true
            n858 = call <userlib>:"Acm_AxGetCmdVelocity.vi"("AxisHandle"=w1608) -> ("Velocity"=w1609:dbl)  [unwired: 1 in, 3 out]
            n859 = Wait Until Next ms Multiple(millisecond multiple=u32 50 ("毫秒倍数")) -> ()  [unwired: 1 out]
            n860 = Equal To 0?(x=w1609) -> (x = 0?=w1604:bool)
            n861 = local read "急停"() -> (w1606:bool)
            n862 = local read "复位"() -> (w1605:bool)
            n863 = Compound Arithmetic op=OR(w1604, invert w1606, w1605) -> (w1603:bool)
          }
        }
        frame #8 {
          n864 = call "PCI1220U角度置零.vi"("AxisHandle IN"=w1610) -> ()  [unwired: 10 in, 1 out]
        }
      }
    }
    frame #2 {
      n865 = flat-sequence {
        frame #0 {
          n866 = while {
            stop <- w1611 stop-if-true
            n867 = local read "电动缸回零"() -> (w1618:bool)
            n868 = local write "回零完成"(TRUE ("回零完成")) -> ()
            n869 = local write "电动缸回零"(FALSE ("电动缸回零")) -> ()
            n870 = Wait Until Next ms Multiple(millisecond multiple=u32 50 ("毫秒倍数")) -> ()  [unwired: 1 out]
            n871 = Not(x=w1618) -> (.not. x?=w1612:bool)
            n872 = local read "急停"() -> (w1613:bool)
            n873 = local read "复位"() -> (w1614:bool)
            n874 = Compound Arithmetic op=OR(w1612, invert w1613, w1614) -> (w1611:bool)
          }
        }
      }
    }
  }
  n875 = while {
    stop <- w1620 stop-if-true
    n876 = stacked-sequence {
      frame #0 {
        n877 = flat-sequence {
          frame #0 {
          }
          frame #1 {
            "PLC" <- "阻挡"
          }
          frame #2 {
            n878 = First Call?() -> (First Call?: T/F=w1622:bool)
            n879 = case shown="真" w1622 {
              frame False {
              }
              frame True {
                n880 = call "员工管理测试程序.vi"() -> ("员工姓名"=w1624:string, "员工ID"=w1623:string)  [unwired: 10 in]
                n881 = local write "员工ID"(w1623) -> ()
                n882 = local write "员工姓名"(w1624) -> ()
              }
            }
          }
          frame #3 {
          }
          frame #4 {
          }
          frame #5 {
          }
          frame #6 {
          }
        }
      }
      frame #1 {
        n883 = flat-sequence {
          frame #0 {
            n884 = property on="型号选择" class="Ring (严格)"() -> ("RingText.Text"=w1625:string)  [unwired: 2 in, 2 out]
            n885 = case shown="\"J728\"" w1625 {
              frame "J709", Default {
                w1626 = FALSE ("可见")
                w1627 = TRUE ("可见")
                n886 = property on="右180°内全行程间隙" class="DigNum (严格)"("Visible"=w1626) -> ()  [unwired: 2 in, 2 out]
                n887 = property on="右180°外全行程间隙" class="DigNum (严格)"("Visible"=w1626) -> ()  [unwired: 2 in, 2 out]
                n888 = property on="左180°外全行程间隙" class="DigNum (严格)"("Visible"=w1626) -> ()  [unwired: 2 in, 2 out]
                n889 = property on="左180°内全行程间隙" class="DigNum (严格)"("Visible"=w1626) -> ()  [unwired: 2 in, 2 out]
                n890 = property on="右全行程间隙" class="DigNum (严格)"("Visible"=w1627) -> ()  [unwired: 2 in, 2 out]
                n891 = property on="左全行程间隙" class="DigNum (严格)"("Visible"=w1627) -> ()  [unwired: 2 in, 2 out]
              }
              frame "J706" {
                w1628 = TRUE ("可见")
                w1629 = FALSE ("可见")
                n892 = property on="右180°内全行程间隙" class="DigNum (严格)"("Visible"=w1628) -> ()  [unwired: 2 in, 2 out]
                n893 = property on="右180°外全行程间隙" class="DigNum (严格)"("Visible"=w1628) -> ()  [unwired: 2 in, 2 out]
                n894 = property on="左180°外全行程间隙" class="DigNum (严格)"("Visible"=w1628) -> ()  [unwired: 2 in, 2 out]
                n895 = property on="左180°内全行程间隙" class="DigNum (严格)"("Visible"=w1628) -> ()  [unwired: 2 in, 2 out]
                n896 = property on="右全行程间隙" class="DigNum (严格)"("Visible"=w1629) -> ()  [unwired: 2 in, 2 out]
                n897 = property on="左全行程间隙" class="DigNum (严格)"("Visible"=w1629) -> ()  [unwired: 2 in, 2 out]
              }
              frame "J728" {
                w1630 = TRUE ("可见")
                w1631 = FALSE ("可见")
                n898 = property on="右180°内全行程间隙" class="DigNum (严格)"("Visible"=w1630) -> ()  [unwired: 2 in, 2 out]
                n899 = property on="右180°外全行程间隙" class="DigNum (严格)"("Visible"=w1630) -> ()  [unwired: 2 in, 2 out]
                n900 = property on="左180°外全行程间隙" class="DigNum (严格)"("Visible"=w1630) -> ()  [unwired: 2 in, 2 out]
                n901 = property on="左180°内全行程间隙" class="DigNum (严格)"("Visible"=w1630) -> ()  [unwired: 2 in, 2 out]
                n902 = property on="右全行程间隙" class="DigNum (严格)"("Visible"=w1631) -> ()  [unwired: 2 in, 2 out]
                n903 = property on="左全行程间隙" class="DigNum (严格)"("Visible"=w1631) -> ()  [unwired: 2 in, 2 out]
              }
            }
          }
          frame #1 {
            (unwired) string[] ["I急停按钮", "I自动旋钮", "I启动按钮", "I备用按钮", "I复位按钮", "I上阻挡器放行", "I下阻挡器放行", "I进支线按钮"] ("I0说明")
            (unwired) string[] ["I出支线按钮", "I主线顶升按钮", "I主线下降按钮", "I支线顶升按钮", "I支线下降按钮", "I气压报警", "未使用", "未使用"] ("I0说明")
            n904 = local read "间隙位移(mm)"() -> (w1634:dbl)
            n905 = Greater Or Equal?(x=w1634, y=4.0) -> (x >= y?=w1632:bool)
            n906 = case shown="真" w1632 {
              frame False {
              }
              frame True {
                n907 = local write "测头机构轴使能"(FALSE ("测头机构轴使能")) -> ()
              }
            }
          }
          frame #2 {
            (unwired) string[] ["I电动缸SRDY", "I电动缸ZSPD", "I电动缸ALRM", "I间隙进给SRDY", "I间隙进给ZSPD", "I间隙进给ALRM", "I间隙旋转SRPD", "I间隙旋转ZSPD"] ("I0说明")
            n908 = local read "测头机构轴位置(mm)"() -> (w1638:dbl)
            n909 = Greater Or Equal?(x=w1638, y=90.0) -> (x >= y?=w1636:bool)
            n910 = case shown="假" w1636 {
              frame False {
                w1639 = T5."Enabled" ("禁用")
                n911 = property on="测头气缸右移" class="Bool"("DisabledEnum"=w1639) -> ()  [unwired: 2 in, 2 out]
                n912 = property on="测头气缸左移" class="Bool"("DisabledEnum"=w1639) -> ()  [unwired: 2 in, 2 out]
                n913 = property on="测头气缸右移" class="Bool (严格)"("DisabledEnum"=w1639) -> ()  [unwired: 2 in, 2 out]
                n914 = property on="测头气缸左移" class="Bool (严格)"("DisabledEnum"=w1639) -> ()  [unwired: 2 in, 2 out]
              }
              frame True {
                w1640 = T5."Disabled" ("禁用")
                w1641 = FALSE ("测头气缸右移")
                n915 = local write "测头气缸右移"(w1641) -> ()
                n916 = local write "测头气缸左移"(w1641) -> ()
                n917 = property on="测头气缸右移" class="Bool"("DisabledEnum"=w1640) -> ()  [unwired: 2 in, 2 out]
                n918 = property on="测头气缸左移" class="Bool"("DisabledEnum"=w1640) -> ()  [unwired: 2 in, 2 out]
                n919 = property on="测头气缸右移" class="Bool (严格)"("DisabledEnum"=w1640) -> ()  [unwired: 2 in, 2 out]
                n920 = property on="测头气缸左移" class="Bool (严格)"("DisabledEnum"=w1640) -> ()  [unwired: 2 in, 2 out]
              }
            }
          }
          frame #3 {
            (unwired) string[] ["I间隙旋转ALRM", "I扭矩旋转SRPD", "I扭矩旋转ZSPD", "I扭矩旋转ALRM", "I拧紧机合格", "I拧紧机不合格", "I拧紧机报警", "未使用"] ("I0说明")
          }
        }
      }
      frame #2 {
        n921 = flat-sequence {
          frame #0 {
            (unwired) string[] ["I自制气缸进位", "I自制气缸原位", "I上工位检测", "I本工位检测", "I下工位检测", "I主线顶升上位", "I主线顶升下位", "I支线顶升上位"] ("I0说明")
          }
          frame #1 {
            (unwired) string[] ["I支线顶升下位", "I支线进到位", "I支线退到位", "I位移气缸原位", "I位移气缸进位", "I拧紧机在位", "I电动缸原位", "I电动缸进位"] ("I0说明")
          }
          frame #2 {
            (unwired) string[] ["未使用", "未使用", "未使用", "未使用", "未使用", "未使用", "未使用", "未使用"] ("I0说明")
          }
          frame #3 {
            (unwired) string[] ["未使用", "未使用", "未使用", "未使用", "未使用", "未使用", "未使用", "未使用"] ("I0说明")
          }
        }
        n922 = local read "本测试状态"() -> (w1643:bool)
        n923 = local read "本自动状态"() -> (w1644:bool)
        n924 = local read "本备料状态"() -> (w1642:bool)
        n925 = local write "本测试状态H"(w1643) -> ()
        n926 = local write "本自动状态H"(w1644) -> ()
        n927 = local write "本备料状态H"(w1642) -> ()
      }
      frame #3 {
        n928 = local read "报警工步号"() -> (w1646:dbl)
        n929 = local read "工步号"() -> (w1648:u32)
        n930 = case shown="50" w1648 {
          tunnel: [w1658 "请取胶瓶" ("工步描述") "请对锁紧螺母加力" ("工步描述") "灵敏度测试中" ("工步描述") "有油刚度测试中" ("工步描述") "安装好锁紧螺母后，按顶升按钮，夹具夹紧" ("工步描述") "请点击启动按钮进行试验" ("工步描述") "探头气缸右移" ("工步描述") "电动缸前进找中" ("工步描述") "探头前进测试开始" ("工步描述") "探头退回" ("工步描述") "轴向力测试中" ("工步描述") "测头后退夹抓松开" ("工步描述") "伺服回零" ("工步描述") "力特性试验完成" ("工步描述") "套好输出轴把手，按启动按钮，做回正力试验" ("工步描述") "回正力试验中" ("工步描述") "试验完成，将把手拉回，取下油管，按顶升按钮" ("工步描述") "拆下锁紧螺母和输入轴万向节，按顶升按钮" ("工步描述")] -> w1647
          frame 0, Default {
            n931 = local read "联线按钮"() -> (w1657:bool)
            n932 = case shown="真" w1657 {
              tunnel: ["等待工件" ("工步描述") "等待扫描条码" ("工步描述")] -> w1658
              frame False {
              }
              frame True {
              }
            }
          }
          frame 1 {
          }
          frame 2 {
          }
          frame 3 {
          }
          frame 4 {
          }
          frame 5 {
          }
          frame 6 {
          }
          frame 10 {
          }
          frame 15 {
          }
          frame 20 {
          }
          frame 30 {
          }
          frame 40 {
          }
          frame 45 {
          }
          frame 50 {
          }
          frame 55 {
          }
          frame 60 {
          }
          frame 70 {
          }
          frame 80 {
          }
          frame 56 {
          }
        }
        "工步提示" <- w1647
        n933 = case shown="3" w1646 {
          tunnel: [_ "操作步骤错请取胶瓶" "操作步骤错误请点标" "测头气缸不在原位" "急停被按下" "气压报警" "电动缸伺服报警" "旋转伺服服报警" "测头伺服服报警"] -> w1645
          frame 0, Default {
          }
          frame 1 {
          }
          frame 3 {
          }
          frame 2 {
          }
          frame 4 {
          }
          frame 5 {
          }
          frame 6 {
          }
          frame 7 {
          }
          frame 8 {
          }
        }
        "报警提示" <- w1645
      }
      frame #4 {
        n934 = local read "急停"() -> (w1679:bool)
        n935 = local read "红灯"() -> (w1681:bool)
        n936 = local read "复位"() -> (w1682:bool)
        n937 = local read "复位"() -> (w1684:bool)
        n938 = local read "红灯"() -> (w1683:bool)
        n939 = case shown="假" w1679 {
          frame False {
            w1687 = TRUE ("红灯")
            n940 = local write "红灯"(w1687) -> ()
            n941 = local write "复位"(w1687) -> ()
          }
          frame True {
            w1688 = FALSE ("复位")
            n942 = local write "红灯"(w1688) -> ()
            n943 = local write "复位"(w1688) -> ()
          }
        }
        n944 = Or(x=w1681, y=w1682) -> (x .or. y?=w1680:bool)
        n945 = case shown="真" w1680 {
          frame False {
          }
          frame True {
            n946 = local write "回零完成"(FALSE ("夹头夹紧控制")) -> ()
          }
        }
        n947 = local read "停止"() -> (w1686:bool)
        n948 = Compound Arithmetic op=OR(w1684, w1686, w1683) -> (w1685:bool)
        n949 = case shown="真" w1685 {
          frame False {
          }
          frame True {
            n950 = local read "测头机构电机"() -> (w1690:u32)
            n951 = local read "旋转齿条电机"() -> (w1691:u32)
            n952 = local read "电动缸电机"() -> (w1692:u32)
            n953 = call "PCI1220U停止.vi"("AxisHandle IN"=w1691) -> ()  [unwired: 9 in, 2 out]
            n954 = call "PCI1220U停止.vi"("AxisHandle IN"=w1692) -> ()  [unwired: 9 in, 2 out]
            n955 = call "PCI1220U停止.vi"("AxisHandle IN"=w1690) -> ()  [unwired: 9 in, 2 out]
          }
        }
      }
      frame #5 {
        n956 = local read "齿条扭矩(Nm)"() -> (w1695:dbl)
        n957 = local read "黄灯"() -> (w1693:bool)
        n958 = local read "旋转齿条轴左转"() -> (w1701:bool)
        n959 = Absolute Value(x=w1695) -> (abs(x)=w1700:dbl)
        n960 = local read "旋转齿条轴右转"() -> (w1696:bool)
        n961 = Not(x=w1701) -> (.not. x?=w1697:bool)
        n962 = Less?(x=w1700, y=20.0) -> (x < y?=w1698:bool)
        n963 = Compound Arithmetic op=AND(w1696, w1697, w1698, w1693) -> (w1694:bool)
        n964 = case shown="真" w1694 {
          frame False {
          }
          frame True {
            n965 = flat-sequence {
              tunnel: [w1705] -> w1703
              tunnel: w1703 -> [w1707]
              tunnel: [w1707] -> w1702
              tunnel: w1702 -> [w1718]
              frame #0 {
                n966 = local read "旋转齿条电机"() -> (w1704:u32)
                n967 = call "PCI1220U运行.vi"("方向"=enum32{"Negative", "Positive"}."Negative" ("Direction"), "AxisHandle IN"=w1704) -> ("AxisHandle OUT"=w1705:u32)  [unwired: 9 in]
              }
              frame #1 {
                n968 = while {
                  stop <- w1711 stop-if-true
                  n969 = Wait (ms)(milliseconds to wait=u32 50 ("毫秒倍数")) -> ()  [unwired: 1 out]
                  n970 = local read "齿条扭矩(Nm)"() -> (w1716:dbl)
                  n971 = local read "旋转齿条轴右转"() -> (w1713:bool)
                  n972 = local read "红灯"() -> (w1708:bool)
                  n973 = local read "复位"() -> (w1709:bool)
                  n974 = Absolute Value(x=w1716) -> (abs(x)=w1715:dbl)
                  n975 = Not(x=w1713) -> (.not. x?=w1710:bool)
                  n976 = Greater?(x=w1715, y=10.0) -> (0:w1712:bool)
                  n977 = Compound Arithmetic op=OR(w1712, w1710, w1709, w1708) -> (w1711:bool)
                }
              }
              frame #2 {
                n978 = call "PCI1220U停止.vi"("AxisHandle IN"=w1718) -> ()  [unwired: 9 in, 2 out]
              }
            }
          }
        }
      }
      frame #6 {
        n979 = local read "齿条扭矩(Nm)"() -> (w1723:dbl)
        n980 = local read "旋转齿条轴右转"() -> (w1727:bool)
        n981 = Absolute Value(x=w1723) -> (abs(x)=w1722:dbl)
        n982 = local read "旋转齿条轴左转"() -> (w1725:bool)
        n983 = local read "黄灯"() -> (w1719:bool)
        n984 = Not(x=w1727) -> (.not. x?=w1724:bool)
        n985 = Less?(x=w1722, y=20.0) -> (x < y?=w1720:bool)
        n986 = Compound Arithmetic op=AND(w1725, w1724, w1720, w1719) -> (w1726:bool)
        n987 = case shown="真" w1726 {
          frame False {
          }
          frame True {
            n988 = flat-sequence {
              tunnel: [w1731] -> w1729
              tunnel: w1729 -> [w1733]
              tunnel: [w1733] -> w1728
              tunnel: w1728 -> [w1744]
              frame #0 {
                n989 = local read "旋转齿条电机"() -> (w1730:u32)
                n990 = call "PCI1220U运行.vi"("方向"=enum32{"Negative", "Positive"}."Positive" ("Direction"), "AxisHandle IN"=w1730) -> ("AxisHandle OUT"=w1731:u32)  [unwired: 9 in]
              }
              frame #1 {
                n991 = while {
                  stop <- w1736 stop-if-true
                  n992 = Wait (ms)(milliseconds to wait=u32 50 ("毫秒倍数")) -> ()  [unwired: 1 out]
                  n993 = local read "齿条扭矩(Nm)"() -> (w1742:dbl)
                  n994 = local read "旋转齿条轴左转"() -> (w1739:bool)
                  n995 = local read "红灯"() -> (w1734:bool)
                  n996 = local read "复位"() -> (w1735:bool)
                  n997 = Absolute Value(x=w1742) -> (abs(x)=w1741:dbl)
                  n998 = Not(x=w1739) -> (.not. x?=w1737:bool)
                  n999 = Greater?(x=w1741, y=10.0) -> (0:w1738:bool)
                  n1000 = Compound Arithmetic op=OR(w1735, w1734, w1738, w1737) -> (w1736:bool)
                }
              }
              frame #2 {
                n1001 = call "PCI1220U停止.vi"("AxisHandle IN"=w1744) -> ()  [unwired: 9 in, 2 out]
              }
            }
          }
        }
      }
      frame #7 {
        n1002 = local read "齿条推拉力(N)"() -> (w1749:dbl)
        n1003 = local read "电动缸前进"() -> (w1746:bool)
        n1004 = local read "电动缸后退"() -> (w1745:bool)
        n1005 = Absolute Value(x=w1749) -> (abs(x)=w1753:dbl)
        n1006 = local read "黄灯"() -> (w1747:bool)
        n1007 = Not(x=w1745) -> (.not. x?=w1750:bool)
        n1008 = Less?(x=w1753, y=1000.0) -> (x < y?=w1751:bool)
        n1009 = Compound Arithmetic op=AND(w1746, w1750, w1747, w1751) -> (w1748:bool)
        n1010 = case shown="真" w1748 {
          frame False {
          }
          frame True {
            n1011 = flat-sequence {
              tunnel: [w1757] -> w1755
              tunnel: w1755 -> [w1759]
              tunnel: [w1759] -> w1754
              tunnel: w1754 -> [w1770]
              frame #0 {
                n1012 = local read "电动缸电机"() -> (w1756:u32)
                n1013 = call "PCI1220U运行.vi"("方向"=enum32{"Negative", "Positive"}."Positive" ("Direction"), "AxisHandle IN"=w1756) -> ("AxisHandle OUT"=w1757:u32)  [unwired: 9 in]
              }
              frame #1 {
                n1014 = while {
                  stop <- w1767 stop-if-true
                  n1015 = local read "电动缸前进"() -> (w1764:bool)
                  n1016 = local read "齿条推拉力(N)"() -> (w1761:dbl)
                  n1017 = Wait (ms)(milliseconds to wait=u32 50 ("毫秒倍数")) -> ()  [unwired: 1 out]
                  n1018 = Absolute Value(x=w1761) -> (abs(x)=w1763:dbl)
                  n1019 = local read "红灯"() -> (w1765:bool)
                  n1020 = local read "复位"() -> (w1766:bool)
                  n1021 = Greater?(x=w1763, y=1000.0) -> (0:w1760:bool)
                  n1022 = Not(x=w1764) -> (.not. x?=w1768:bool)
                  n1023 = Compound Arithmetic op=OR(w1766, w1765, w1768, w1760) -> (w1767:bool)
                }
              }
              frame #2 {
                n1024 = call "PCI1220U停止.vi"("AxisHandle IN"=w1770) -> ()  [unwired: 9 in, 2 out]
              }
            }
          }
        }
      }
      frame #8 {
        n1025 = local read "电动缸前进"() -> (w1771:bool)
        n1026 = local read "齿条推拉力(N)"() -> (w1775:dbl)
        n1027 = local read "电动缸后退"() -> (w1772:bool)
        n1028 = Absolute Value(x=w1775) -> (abs(x)=w1779:dbl)
        n1029 = local read "黄灯"() -> (w1773:bool)
        n1030 = Not(x=w1771) -> (.not. x?=w1776:bool)
        n1031 = Less?(x=w1779, y=1000.0) -> (x < y?=w1777:bool)
        n1032 = Compound Arithmetic op=AND(w1772, w1776, w1773, w1777) -> (w1774:bool)
        n1033 = case shown="真" w1774 {
          frame False {
          }
          frame True {
            n1034 = flat-sequence {
              tunnel: [w1783] -> w1781
              tunnel: w1781 -> [w1785]
              tunnel: [w1785] -> w1780
              tunnel: w1780 -> [w1796]
              frame #0 {
                n1035 = local read "电动缸电机"() -> (w1782:u32)
                n1036 = call "PCI1220U运行.vi"("方向"=enum32{"Negative", "Positive"}."Negative" ("Direction"), "AxisHandle IN"=w1782) -> ("AxisHandle OUT"=w1783:u32)  [unwired: 9 in]
              }
              frame #1 {
                n1037 = while {
                  stop <- w1793 stop-if-true
                  n1038 = local read "电动缸后退"() -> (w1790:bool)
                  n1039 = local read "齿条推拉力(N)"() -> (w1789:dbl)
                  n1040 = Wait (ms)(milliseconds to wait=u32 50 ("毫秒倍数")) -> ()  [unwired: 1 out]
                  n1041 = Absolute Value(x=w1789) -> (abs(x)=w1787:dbl)
                  n1042 = local read "红灯"() -> (w1792:bool)
                  n1043 = local read "复位"() -> (w1791:bool)
                  n1044 = Greater?(x=w1787, y=1000.0) -> (0:w1786:bool)
                  n1045 = Not(x=w1790) -> (.not. x?=w1794:bool)
                  n1046 = Compound Arithmetic op=OR(w1791, w1792, w1794, w1786) -> (w1793:bool)
                }
              }
              frame #2 {
                n1047 = call "PCI1220U停止.vi"("AxisHandle IN"=w1796) -> ()  [unwired: 9 in, 2 out]
              }
            }
          }
        }
      }
      frame #9 {
        n1048 = local read "测头机构轴后退"() -> (w1797:bool)
        n1049 = local read "测头机构轴前进"() -> (w1798:bool)
        n1050 = local read "黄灯"() -> (w1799:bool)
        n1051 = Not(x=w1797) -> (.not. x?=w1801:bool)
        n1052 = Compound Arithmetic op=AND(w1798, w1801, w1799) -> (w1800:bool)
        n1053 = case shown="真" w1800 {
          frame False {
          }
          frame True {
            n1054 = flat-sequence {
              tunnel: [w1805] -> w1803
              tunnel: w1803 -> [w1807]
              tunnel: [w1807] -> w1802
              tunnel: w1802 -> [w1814]
              frame #0 {
                n1055 = local read "测头机构电机"() -> (w1804:u32)
                n1056 = call "PCI1220U运行.vi"("方向"=enum32{"Negative", "Positive"}."Positive" ("Direction"), "AxisHandle IN"=w1804) -> ("AxisHandle OUT"=w1805:u32)  [unwired: 9 in]
              }
              frame #1 {
                n1057 = while {
                  stop <- w1811 stop-if-true
                  n1058 = local read "测头机构轴前进"() -> (w1808:bool)
                  n1059 = Wait (ms)(milliseconds to wait=u32 50 ("毫秒倍数")) -> ()  [unwired: 1 out]
                  n1060 = local read "红灯"() -> (w1809:bool)
                  n1061 = local read "复位"() -> (w1810:bool)
                  n1062 = Not(x=w1808) -> (.not. x?=w1812:bool)
                  n1063 = Compound Arithmetic op=OR(w1810, w1809, w1812) -> (w1811:bool)
                }
              }
              frame #2 {
                n1064 = call "PCI1220U停止.vi"("AxisHandle IN"=w1814) -> ()  [unwired: 9 in, 2 out]
              }
            }
          }
        }
      }
      frame #10 {
        n1065 = local read "测头机构轴前进"() -> (w1815:bool)
        n1066 = local read "测头机构轴后退"() -> (w1816:bool)
        n1067 = local read "黄灯"() -> (w1817:bool)
        n1068 = Not(x=w1815) -> (.not. x?=w1819:bool)
        n1069 = Compound Arithmetic op=AND(w1816, w1819, w1817) -> (w1818:bool)
        n1070 = case shown="真" w1818 {
          frame False {
          }
          frame True {
            n1071 = flat-sequence {
              tunnel: [w1823] -> w1821
              tunnel: w1821 -> [w1825]
              tunnel: [w1825] -> w1820
              tunnel: w1820 -> [w1832]
              frame #0 {
                n1072 = local read "测头机构电机"() -> (w1822:u32)
                n1073 = call "PCI1220U运行.vi"("方向"=enum32{"Negative", "Positive"}."Negative" ("Direction"), "AxisHandle IN"=w1822) -> ("AxisHandle OUT"=w1823:u32)  [unwired: 9 in]
              }
              frame #1 {
                n1074 = while {
                  stop <- w1829 stop-if-true
                  n1075 = local read "测头机构轴后退"() -> (w1826:bool)
                  n1076 = Wait (ms)(milliseconds to wait=u32 50 ("毫秒倍数")) -> ()  [unwired: 1 out]
                  n1077 = local read "红灯"() -> (w1828:bool)
                  n1078 = local read "复位"() -> (w1827:bool)
                  n1079 = Not(x=w1826) -> (.not. x?=w1830:bool)
                  n1080 = Compound Arithmetic op=OR(w1827, w1828, w1830) -> (w1829:bool)
                }
              }
              frame #2 {
                n1081 = call "PCI1220U停止.vi"("AxisHandle IN"=w1832) -> ()  [unwired: 9 in, 2 out]
              }
            }
          }
        }
      }
      frame #11 {
        n1082 = local read "电动缸回零"() -> (w1833:bool)
        n1083 = case shown="真" w1833 {
          frame False {
          }
          frame True {
          }
        }
      }
    }
    n1084 = Wait (ms)(milliseconds to wait=u32 50 ("毫秒倍数")) -> ()  [unwired: 1 out]
    n1085 = local read "停止"() -> (w1620:bool)
  }
  n1086 = event shown="[0] 超时" {
    selector: _ -> [_ _]
    dyn-events: _ -> [_ _]
    timeout: _ -> [_ _]
    event Timeout {
      n1087 = event-data() -> ()  [unwired: 1 in, 3 out]
      n1088 = Equal?(x="密码", y="jizhuan") -> (x = y?=w1837:bool)
      n1089 = Compound Arithmetic op=AND(w1837, "?") -> (w1835:bool)
      n1090 = case shown="假" w1835 {
        frame False {
          n1091 = property class="Bool (严格)"("DisabledEnum"=T5."Disabled and Grayed Out" ("禁用")) -> ()  [unwired: 2 in, 2 out]
          n1092 = property class="Bool (严格)"("DisabledEnum"=T5."Disabled and Grayed Out" ("禁用")) -> ()  [unwired: 2 in, 2 out]
        }
        frame True {
          n1093 = property class="Bool (严格)"("DisabledEnum"=T5."Enabled" ("禁用")) -> ()  [unwired: 2 in, 2 out]
          n1094 = property class="Bool (严格)"("DisabledEnum"=T5."Enabled" ("禁用")) -> ()  [unwired: 2 in, 2 out]
          n1095 = case shown="真" "?" {
            frame False {
            }
            frame True {
              n1096 = property on="选项卡控件" class="TabCtl (严格)"() -> ("Pages"=w1847:refnum<vi>[])  [unwired: 2 in, 2 out]
              n1097 = for {
                N: 7 -> [_]
                tunnel: w1847 -> [w1849] mode=indexing
                i -> [w1850]
                n1098 = case shown="5" w1850 {
                  tunnel: w1849 -> [_ w1852]
                  frame 0, Default {
                  }
                  frame 5 {
                    n1099 = property class="Page"(reference=w1852, "PageVis"=FALSE ("选项卡可见")) -> ()  [unwired: 1 in, 2 out]
                  }
                }
              }
            }
          }
          n1100 = case shown="真" "?" {
            frame False {
            }
            frame True {
              n1101 = property on="选项卡控件" class="TabCtl (严格)"() -> ("Pages"=w1853:refnum<vi>[])  [unwired: 2 in, 2 out]
              n1102 = for {
                N: 7 -> [_]
                tunnel: w1853 -> [w1855] mode=indexing
                i -> [w1856]
                n1103 = case shown="5" w1856 {
                  tunnel: w1855 -> [_ w1858]
                  frame 0, Default {
                  }
                  frame 5 {
                    n1104 = property class="Page"(reference=w1858, "PageVis"=TRUE ("选项卡可见")) -> ()  [unwired: 1 in, 2 out]
                  }
                }
              }
            }
          }
        }
      }
      n1105 = Not(x=w1835) -> (.not. x?=w1834:bool)
      n1106 = case shown="真" w1834 {
        frame False {
        }
        frame True {
          n1107 = call "显示对话框信息"("Enable"=TRUE) -> ()  [unwired: 9 in, 2 out]
        }
      }
    }
    event "确定按钮": Value Change {
      n1108 = event-data() -> ()  [unwired: 1 in, 6 out]
    }
  }
  n1109 = flat-sequence {
    tunnel: [w1862] -> w2
    tunnel: [w1860] -> w1
    tunnel: w2 -> [w1872]
    tunnel: w1 -> [w1871]
    frame #0 {
      n1110 = First Call?() -> (First Call?: T/F=w1859:bool)
      n1111 = case shown="真" w1859 {
        frame False {
        }
        frame True {
          n1112 = while {
            i -> [w1867]
            stop <- w1865 stop-if-true
            w1870 = TRUE ("电动缸使能")
            n1113 = local write "回零完成"(FALSE ("回零完成")) -> ()
            n1114 = local write "测头机构轴使能"(w1870) -> ()
            n1115 = local write "旋转齿条轴使能"(w1870) -> ()
            n1116 = local write "电动缸使能"(w1870) -> ()
            n1117 = Wait Until Next ms Multiple(millisecond multiple=u32 50 ("毫秒倍数")) -> ()  [unwired: 1 out]
            n1118 = Greater Or Equal?(x=w1867, y=30) -> (x >= y?=w1865:bool)
          }
        }
      }
      n1119 = call "ADO Connection Create.vi"() -> ("error out"=w1863:errorcluster, "ADODB._Connection Out"=w1864:refnum<k7>)  [unwired: 10 in]
      n1120 = call "ADO Connection Open.vi"("error in (no error)"=w1863, "ConnectionString"="Provider=Microsoft.Jet.OLEDB.4.0;Data Source=D:\\Q14070-Z060人机界面\\参数\\参数Z060.mdb;Persist Security Info=False;Jet OLEDB:Database Password=1234;", "ADODB._Connection In"=w1864) -> ("error out"=w1860:errorcluster, "ADODB._Connection Out"=w1862:refnum<k7>)  [unwired: 7 in]
    }
    frame #1 {
      n1121 = while {
        tunnel: w1872 -> [w1874]
        tunnel: w1871 -> [w1873]
        stop <- w1878 stop-if-true
        n1122 = Wait (ms)(milliseconds to wait=u32 50 ("等待时间（毫秒）")) -> ()  [unwired: 1 out]
        n1123 = First Call?() -> (First Call?: T/F=w1877:bool)
        n1124 = Or(x=w1877, y="参数加载") -> (x .or. y?=w1876:bool)
        n1125 = case shown="真" w1876 {
          tunnel: w1874 -> [_ w1881]
          tunnel: w1873 -> [_ w1880]
          frame False {
          }
          frame True {
            n1126 = stacked-sequence {
              tunnel: w1881 -> [w1887 w1898 w1956]
              tunnel: w1880 -> [w1882 _ _]
              frame #0 {
                n1127 = call "SQL Execute.vi"("error in (no error)"=w1882, "Command Text"="SELECT * FROM 测试参数表", "ADODB._Connection In"=w1887) -> ("Data"=w1885:string[][])  [unwired: 5 in, 3 out]
                n1128 = Index Array(array=w1885, index (col)=0 ("索引 (行)")) -> (element=w1889:string[])  [unwired: 1 in]
                n1129 = Array Size(array=w1889) -> (size(s)=w1884:i32)
                "型号数量" <- w1884
                n1130 = while {
                  shift-right: [w1896] -> w1888
                  shift-left: i32[] [] -> [w1895]
                  tunnel: w1884 -> [w1893]
                  i -> [w1894]
                  stop <- w1892 stop-if-true
                  n1131 = Greater Or Equal?(x=w1894, y=w1893) -> (x >= y?=w1892:bool)
                  n1132 = Build Array (concatenate)(w1895, w1894) -> (w1896:i32[])
                }
                n1133 = Build Cluster Array "索引与捆绑簇数组"(w1889, w1888) -> (w1883:cluster{"String":string, i32}[])
                n1134 = property on="型号选择" class="Ring (严格)"("StringsAndValues[]"=w1883) -> ()  [unwired: 2 in, 2 out]
              }
              frame #1 {
                n1135 = property on="型号选择" class="Ring (严格)"() -> ("RingText.Text"=w1899:string)  [unwired: 2 in, 2 out]
                n1136 = call "创建文本2"("型号选择"=w1899) -> ("Result"=w1903:string)  [unwired: 13 in, 1 out]
                n1137 = call "SQL Execute.vi"("Command Text"=w1903, "ADODB._Connection In"=w1898) -> ("Data"=w1902:string[][])  [unwired: 6 in, 3 out]
                n1138 = Index Array(array=w1902, index (row)=0 ("索引 (行)")) -> (element=w1900:string[])  [unwired: 1 in]
                n1139 = Fract/Exp String To Number ("分数/指数字符串至数值转换")(string=w1900) -> (number=w1897:dbl[])  [unwired: 3 in, 1 out]
                n1140 = stacked-sequence {
                  tunnel: w1897 -> [w1932]
                  frame #0 {
                    n1141 = Index Array ("索引数组")(array=w1932, index #1=2 ("索引"), index #2=3 ("索引"), index #3=4 ("索引"), index #4=5 ("索引"), index #5=6 ("索引"), index #6=7 ("索引"), index #7=8 ("索引"), index #8=9 ("索引"), index #9=10 ("索引"), index #10=11 ("索引"), index #11=12 ("索引"), index #12=13 ("索引"), index #13=14 ("索引"), index #14=15 ("索引"), index #15=16 ("索引"), index #16=17 ("索引"), index #17=18 ("索引"), index #18=19 ("索引"), index #19=20 ("索引")) -> (element #1=w1931:dbl, element #2=w1930:dbl, element #3=w1929:dbl, element #4=w1928:dbl, element #5=w1927:dbl, element #6=w1926:dbl, element #7=w1925:dbl, element #8=w1924:dbl, element #9=w1923:dbl, element #10=w1922:dbl, element #11=w1915:dbl, element #12=w1914:dbl, element #13=w1913:dbl, element #14=w1912:dbl, element #15=w1911:dbl, element #16=w1910:dbl, element #17=w1907:dbl, element #18=w1906:dbl, element #19=w1904:dbl)
                    n1142 = local write "测头机构轴移动速度"(w1931) -> ()
                    n1143 = local write "总圈数标准"(w1907) -> ()
                    n1144 = local write "总圈数最大值"(w1906) -> ()
                    n1145 = local write "平均轴向力标准(N) max"(w1910) -> ()
                    n1146 = local write "测头机构轴检测位"(w1930) -> ()
                    n1147 = local write "测头机构轴后退位"(w1928) -> ()
                    n1148 = local write "测头机构轴待检位"(w1929) -> ()
                    n1149 = local write "旋转齿条轴找帽转速"(w1924) -> ()
                    n1150 = local write "旋转齿条轴测量转速"(w1923) -> ()
                    n1151 = local write "转向器中心"(w1904) -> ()
                    n1152 = local write "总行程标准(mm)"(w1915) -> ()
                    n1153 = local write "轴向力标准(N)"(w1911) -> ()
                    n1154 = local write "齿条移动速度"(w1927) -> ()
                    n1155 = local write "齿条左极限"(w1926) -> ()
                    n1156 = local write "齿条右极限"(w1925) -> ()
                    n1157 = local write "力波动标准(N)"(w1912) -> ()
                    n1158 = local write "总行程最大值"(w1914) -> ()
                    n1159 = local write "测量点扭矩"(w1922) -> ()
                    n1160 = local write "齿条传动比"(w1913) -> ()
                  }
                }
              }
              frame #2 {
                n1161 = call "SQL Execute.vi"("Command Text"="SELECT * FROM 传感器校验表 where ID='1'", "ADODB._Connection In"=w1956) -> ("Data"=w1958:string[][])  [unwired: 6 in, 3 out]
                n1162 = Index Array(array=w1958) -> (element=w1959:string[])  [unwired: 2 in]
                n1163 = Fract/Exp String To Number ("分数/指数字符串至数值转换")(string=w1959) -> (number=w1949:dbl[])  [unwired: 3 in, 1 out]
                n1164 = Index Array(array=w1949, index #1=1 ("索引"), index #2=2 ("索引"), index #3=3 ("索引"), index #4=4 ("索引"), index #5=5 ("索引"), index #6=6 ("索引")) -> (element #1=w1948:dbl, element #2=w1947:dbl, element #3=w1946:dbl, element #4=w1945:dbl, element #5=w1944:dbl, element #6=w1943:dbl)
                n1165 = local write "间隙位移零点偏移"(w1948) -> ()
                n1166 = local write "间隙位移比例偏移"(w1947) -> ()
                n1167 = local write "齿条推拉力零点偏移"(w1946) -> ()
                n1168 = local write "齿条推拉力比例偏移"(w1945) -> ()
                n1169 = local write "齿条扭矩零点偏移"(w1944) -> ()
                n1170 = local write "齿条扭矩比例偏移"(w1943) -> ()
              }
            }
          }
        }
        n1171 = local read "停止"() -> (w1878:bool)
        "ADODB._Connection Out 2" <- w1874
      }
    }
  }
  n1172 = while {
    stop <- w1961 stop-if-true
    n1173 = local read "rfid工步号"() -> (w1960:u32)
    n1174 = case shown="10" w1960 {
      frame 0, Default {
      }
      frame 10 {
        n1175 = flat-sequence {
          tunnel: [w1971] -> w1965
          tunnel: w1965 -> [w1973]
          tunnel: [w1972] -> w1964
          tunnel: w1964 -> [w1975]
          tunnel: [w1975] -> w1963
          tunnel: w1963 -> [w1978]
          frame #0 {
            n1176 = while {
              stop <- w1966 stop-if-true
              n1177 = local read "rfid触发"() -> (w1966:bool)
              n1178 = Wait Until Next ms Multiple(millisecond multiple=u32 50 ("毫秒倍数")) -> ()  [unwired: 1 out]
            }
          }
          frame #1 {
            n1179 = local write "芯片ID"("" ("随行板ID")) -> ()
            n1180 = local write "rfid完成"(FALSE ("RFID完成")) -> ()
            n1181 = local write "rfid触发"(FALSE ("RFID读取触发")) -> ()
          }
          frame #2 {
            n1182 = local read "Z060BRFID"() -> (w1971:string)
            n1183 = local write "芯片ID"(w1971) -> ()
          }
          frame #3 {
            n1184 = call "查询产品ID.vi"("芯片编码"=w1973) -> ("产品ID"=w1972:string)  [unwired: 8 in, 2 out]
            "读取产品ID" <- w1972
          }
          frame #4 {
            n1185 = Wait (ms)(milliseconds to wait=u32 500 ("等待时间（毫秒）")) -> ()  [unwired: 1 out]
          }
          frame #5 {
            n1186 = call "查询上序合格.vi"("产品ID"=w1978) -> ("本序已做"=w1976:bool, "上序合格"=w1977:bool)  [unwired: 8 in, 1 out]
            n1187 = Not(x=w1977) -> (.not. x?=w1979:bool)
            n1188 = local write "上序合格"(w1977) -> ()
            n1189 = local write "本序已做"(w1976) -> ()
            n1190 = local write "上序不合格"(w1979) -> ()
          }
          frame #6 {
            n1191 = local write "rfid完成"(TRUE ("RFID读取完成")) -> ()
            n1192 = Wait Until Next ms Multiple(millisecond multiple=u32 500 ("毫秒倍数")) -> ()  [unwired: 1 out]
          }
          frame #7 {
            "rfid工步号" <- 15.0 ("工步号")
          }
        }
      }
      frame 210 {
        n1193 = local read "读取产品ID"() -> (w1983:string)
        n1194 = local write "产品ID"(w1983) -> ()
      }
    }
    n1195 = Wait Until Next ms Multiple(millisecond multiple=u32 50 ("毫秒倍数")) -> ()  [unwired: 1 out]
    n1196 = local read "停止"() -> (w1961:bool)
  }
  n1197 = flat-sequence {
    tunnel: [w1984] -> w4
    tunnel: w4 -> [w1990]
    tunnel: [w1989] -> w3
    tunnel: w3 -> [w2056]
    frame #0 {
      n1198 = call "PCI1240U初始化.vi"() -> ("旋转电机"=→"旋转齿条电机":u32, "电动缸电机"=→"电动缸电机":u32, "DeviceHandle"=→"DeviceHandle":u32, "进给电机"=→"测头机构电机":u32)  [unwired: 6 in, 2 out]
      n1199 = call "PCI8622配置.vi"() -> ("DeviceID"=w1984:i32)  [unwired: 11 in]
    }
    frame #1 {
      n1200 = while {
        tunnel: w1990 -> [w1992]
        tunnel: [w1991] -> w1989
        stop <- "停止" stop-if-true
        n1201 = stacked-sequence {
          tunnel: w1992 -> [_ _ w2032]
          tunnel: [_ _ w2032] -> w1991
          frame #0 {
            n1202 = local read "测头机构电机"() -> (w2001:u32)
            n1203 = Boolean To (0,1)(Boolean="测头机构轴使能") -> (0, 1=w1999:i16)
            n1204 = call <userlib>:"Acm_AxSetSvOn.vi"("OnOff"=w1999, "AxisHandle"=w2001) -> ("AxisHandle"=w1998:u32)  [unwired: 1 in, 2 out]
            n1205 = call "PCI1220U进给轴速度设置.vi"("Change Velocity"="测头机构轴速度(mm/s)", "AxisHandle IN"=w1998) -> ("AxisHandle OUT"=w1996:u32)  [unwired: 9 in]
            n1206 = call "PCI1220U进给轴读取位置.vi"("AxisHandle IN"=w1996) -> ("位置"=→"测头机构轴位置(mm)":dbl)  [unwired: 9 in, 1 out]
          }
          frame #1 {
            n1207 = local read "电动缸电机"() -> (w2011:u32)
            n1208 = local read "旋转齿条电机"() -> (w2010:u32)
            n1209 = Boolean To (0,1)(Boolean="电动缸使能") -> (0, 1=w2015:i16)
            n1210 = Boolean To (0,1)(Boolean="旋转齿条轴使能") -> (0, 1=w2009:i16)
            n1211 = call <userlib>:"Acm_AxSetSvOn.vi"("OnOff"=w2009, "AxisHandle"=w2010) -> ("AxisHandle"=w2012:u32)  [unwired: 1 in, 2 out]
            n1212 = call <userlib>:"Acm_AxSetSvOn.vi"("OnOff"=w2015, "AxisHandle"=w2011) -> ("AxisHandle"=w2014:u32)  [unwired: 1 in, 2 out]
            n1213 = call "PCI1220U扭矩轴速度设置.vi"("Change Velocity"="旋转齿条轴速度(°/s)", "AxisHandle IN"=w2012) -> ("AxisHandle OUT"=w2013:u32)  [unwired: 9 in]
            n1214 = call "PCI1240电动缸速度设置.vi"("Change Velocity"="电动缸速度(mm/s)", "AxisHandle IN"=w2014) -> ("AxisHandle OUT"=w2002:u32)  [unwired: 9 in]
            n1215 = call "PCI1220U扭矩轴读取位置.vi"("AxisHandle IN"=w2013) -> ("位置"=→"旋转齿条轴位置(°)":dbl)  [unwired: 9 in, 1 out]
            n1216 = call "PCI1240电动缸读取位置.vi"("AxisHandle IN"=w2002) -> ("位置"=→"电动缸位置(mm)":dbl)  [unwired: 9 in, 1 out]
          }
          frame #2 {
            w2048 = 0  # nRetSizeWords
            w2049 = 2048  # nReadSizeWords
            # "hDevice"
            n1217 = Initialize Array(u16 0, 2048 ("dimension size")) -> (w2039:u16[])
            n1218 = dll-call lib="PCI8622_32.dll" fn="PCI8622_ReadDeviceProAD_Npt" label="ReadDeviceProAD_Npt"("hDevice"=w2032, "ADBuffer[]"=w2039, "nReadSizeWords"=w2049, "nRetSizeWords"=w2048) -> ("ADBuffer[]"=w2042:u16[])  [unwired: 7 in, 2 out]
            n1219 = Divide(x=w2042, y=65536.01) -> (x/y=w2043:dbl[])
            n1220 = Multiply(x=w2043, y=20) -> (x*y=w2046:dbl[])
            n1221 = Subtract(x=w2046, y=10) -> (x-y=w2038:dbl[])
            n1222 = Decimate 1D Array ("抽取一维数组")(w2038) -> (w2026:dbl[], w2027:dbl[], w2025:dbl[])  [unwired: 5 out]
            n1223 = Add Array Elements(numeric array=w2026) -> (sum=w2035:dbl)
            n1224 = Add Array Elements(numeric array=w2025) -> (sum=w2036:dbl)
            n1225 = Array Size(array=w2026) -> (size(s)=w2034:i32)
            n1226 = Add Array Elements(numeric array=w2027) -> (sum=w2031:dbl)
            n1227 = Array Size(array=w2025) -> (size(s)=w2037:i32)
            n1228 = Array Size(array=w2027) -> (size(s)=w2033:i32)
            n1229 = Divide(x=w2035, y=w2034) -> (x/y=w2024:dbl)
            n1230 = Divide(x=w2036, y=w2037) -> (x/y=w2018:dbl)
            n1231 = Divide(x=w2031, y=w2033) -> (x/y=w2021:dbl)
            n1232 = Subtract(x=w2018, y=4.43) -> (x-y=w2016:dbl)
            n1233 = Multiply(x=w2024, y=2.0) -> (x*y=w2019:dbl)
            n1234 = Multiply(x=w2021, y=200.0) -> (x*y=w2020:dbl)
            n1235 = local read "间隙位移比例偏移"() -> (w2053:dbl)
            n1236 = local read "间隙位移零点偏移"() -> (w2052:dbl)
            n1237 = local read "齿条扭矩零点偏移"() -> (w2054:dbl)
            n1238 = local read "齿条扭矩比例偏移"() -> (w2055:dbl)
            n1239 = local read "齿条推拉力比例偏移"() -> (w2051:dbl)
            n1240 = local read "齿条推拉力零点偏移"() -> (w2050:dbl)
            n1241 = call "传感器校订.vi"("零点"=w2054, "比例"=w2055, "传感器"=w2019) -> ("示值"=→"齿条扭矩(Nm)":dbl)  [unwired: 8 in]
            n1242 = call "传感器校订.vi"("零点"=w2052, "比例"=w2053, "传感器"=w2016) -> ("示值"=→"间隙位移(mm)":dbl)  [unwired: 8 in]
            n1243 = call "传感器校订.vi"("零点"=w2050, "比例"=w2051, "传感器"=w2020) -> ("示值"=→"齿条推拉力(N)":dbl)  [unwired: 8 in]
          }
        }
        n1244 = Wait Until Next ms Multiple(millisecond multiple=u32 50 ("毫秒倍数")) -> ()  [unwired: 1 out]
      }
    }
    frame #2 {
      n1245 = dll-call lib="PCI8622_32.dll" fn="PCI8622_StopDeviceProAD" label="StopDeviceProAD"("hDevice"=w2056) -> ("hDevice"=w2057:i32)  [unwired: 4 in, 2 out]
      n1246 = dll-call lib="PCI8622_32.dll" fn="PCI8622_ReleaseDeviceProAD" label="ReleaseDeviceProAD"("hDevice"=w2057) -> ()  [unwired: 5 in, 2 out]
      n1247 = dll-call lib="PCI8622_32.dll" fn="PCI8622_ReleaseDevice" label="ReleaseDevice"("hDevice"=w2056) -> ()  [unwired: 5 in, 2 out]
    }
  }
